vi "tvac_gui_chamber_backup.vi"() -> ()   [LabVIEW 2017]
uses:
  Zones.ctl
  <vilib>/Utility/miscctls.llb/LVPositionTypeDef.ctl
  <vilib>/httpClient/ClientHandle.ctl
  <vilib>/Utility/miscctls.llb/LVBoundsTypeDef.ctl
  <vilib>/Utility/error.llb/DialogType.ctl
  msg7171_linux.llb/send single message.vi
  <vilib>/httpClient/POSTBuffer.vi
  <vilib>/Utility/file.llb/Read Delimited Spreadsheet (string).vi
  <vilib>/Utility/file.llb/Write Delimited Spreadsheet (string).vi
  <vilib>/httpClient/LabVIEWHTTPClient.lvlib
panel:
  in  "TCs1to45InitialPositions":T1[](array[typedef])=[{"Left"=536, "Top"=477}, {"Left"=577, "Top"=477}, {"Left"=619, "Top"=477}, {"Left"=661, "Top"=477}, {"Left"=702, "Top"=477}, {"Left"=744, "Top"=477}, {"Left"=786, "Top"=477}, {"Left"=827, "Top"=477}, {"Left"=869, "Top"=477}, {"Left"=911, "Top"=477}, {"Left"=952, "Top"=477}, {"Left"=994, "Top"=477}, {"Left"=1036, "Top"=477}, {"Left"=1077, "Top"=477}, {"Left"=1119, "Top"=477}, {"Left"=536, "Top"=516}, {"Left"=577, "Top"=516}, {"Left"=619, "Top"=516}, {"Left"=661, "Top"=516}, {"Left"=702, "Top"=516}, {"Left"=744, "Top"=516}, {"Left"=786, "Top"=516}, {"Left"=827, "Top"=516}, {"Left"=869, "Top"=516}, {"Left"=911, "Top"=516}, {"Left"=952, "Top"=516}, {"Left"=994, "Top"=516}, {"Left"=1036, "Top"=516}, {"Left"=1077, "Top"=516}, {"Left"=1119, "Top"=516}, {"Left"=536, "Top"=555}, {"Left"=577, "Top"=555}, {"Left"=619, "Top"=555}, {"Left"=661, "Top"=555}, {"Left"=702, "Top"=555}, {"Left"=744, "Top"=555}, {"Left"=786, "Top"=555}, {"Left"=827, "Top"=555}, {"Left"=869, "Top"=555}, {"Left"=911, "Top"=555}, {"Left"=952, "Top"=555}, {"Left"=994, "Top"=555}, {"Left"=1036, "Top"=555}, {"Left"=1077, "Top"=555}, {"Left"=1119, "Top"=555}]
  in  "Moving 2":bool
  in  "Moving 1":bool
  in  "TC1to45PicRef":refnum<vi>
  in  "profilearray":dbl[][](array[numeric])
  in  "LastSetPt":i32
  in  "TVAC Labview":bool=TRUE
  in  "string":string
  in  "tprofilesheet":string[][](array[string])
  in  "Custom Graph Selector":i32
  in  "exit":bool
  in  "AlarmColor":u32(colorbox)
  in  "Alarm String":string
  in  "Plot Color":u32(colorbox)=16860
  in  "Temperature":dbl format="%#_13g"
  in  "TC Label":string
  in  "Graph ON/OFF":u32(colorbox)=4250624
  in  "index (col)":i32
  in  "index (row)":i32
  out "working array":bool[](array[boolean])
  in  "Local Debug":bool
  in  "Tab Control":T2(tab)
  in  "Log/Linear Y-Axis":u16(ring) items=["Linear", "Log"]
  in  "Total Time":dbl
  in  "Set Time TC Graph":bool
  in  "Graphing Selection":u16(ring) items=["User Selection", "Graph All Thermocouples", "Clear Graph"]
  in  "Time Scale":u16(ring) items=["Minutes", "Hours", "Seconds"]
  out "Waveform Chart":waveform(dbl)[](graph)
  out "Thermocouples":T3(array[cluster])
  in  "Log/Linear Y-Axis 6":u16(ring) items=["Linear", "Log"]
  in  "Log/Linear Y-Axis 5":u16(ring) items=["Linear", "Log"]
  in  "Log/Linear Y-Axis 3":u16(ring) items=["Linear", "Log"]
  in  "Log/Linear Y-Axis 2":u16(ring) items=["Linear", "Log"]
  in  "Total Time 6":dbl
  in  "Set Time TC Graph 6":bool
  in  "Time Scale 6":u16(ring) items=["Minutes", "Hours", "Seconds"]
  in  "Total Time 5":dbl
  in  "Set Time TC Graph 5":bool
  in  "Time Scale 5":u16(ring) items=["Minutes", "Hours", "Seconds"]
  in  "Total Time 4":dbl
  in  "Set Time TC Graph 4":bool
  in  "Time Scale 4":u16(ring) items=["Minutes", "Hours", "Seconds"]
  in  "Total Time 3":dbl
  in  "Set Time TC Graph 3":bool
  in  "Time Scale 3":u16(ring) items=["Minutes", "Hours", "Seconds"]
  in  "Total Time 2":dbl
  in  "Set Time TC Graph 2":bool
  in  "Time Scale 2":u16(ring) items=["Minutes", "Hours", "Seconds"]
  in  "Log/Linear Y-Axis 1":u16(ring) items=["Linear", "Log"]
  in  "Total Time 1":dbl
  in  "Set Time TC Graph 1":bool
  in  "Time Scale 1":u16(ring) items=["Minutes", "Hours", "Seconds"]
  in  "Custom Chart 2 Selection":i32[](listbox)=[0]
  in  "Custom Chart 1 Selection":i32[](listbox)=[0]
  out "Custom Chart 1":waveform(dbl)[](graph)
  in  "Custom Chart 3 Selection":i32[](listbox)=[0]
  in  "Custom Chart 4 Selection":i32[](listbox)=[0]
  in  "Custom Chart 5 Selection":i32[](listbox)=[0]
  in  "Custom Chart 6 Selection":i32[](listbox)=[0]
  out "Custom Chart 2":waveform(dbl)[](graph)
  out "Custom Chart 3":waveform(dbl)[](graph)
  out "Custom Chart 4":waveform(dbl)[](graph)
  out "Custom Chart 5":waveform(dbl)[](graph)
  out "Custom Chart 6":waveform(dbl)[](graph)
  in  "Log/Linear Y-Axis 4":u16(ring) items=["Linear", "Log"]
  out "ThermalProfileStatus":string
  in  "Import Profile":bool
  out "Thermal Profile":cluster{dbl, dbl, "temp":dbl[][]}(graph)
  in  "CreateTProfile":T4(tab)
  in  "ZoneSetup":T5={"Number of Set points"=0.0, "Zone Selection"=[8], "Initiate Setup"=FALSE, "Thermal Profile Name"=""}
  in  "RampSoakTimes":cluster{"RampSoakTimes":dbl[][]}
  in  "Zone 1":T6={"Zone Thermocouples"=[0], "Temperature Calculation"=0, "Thermocouples Selected"="", "Temperature Goal"=[], "Max Allowable Temp"="", "Min Allowable Temp"="", "Max Temp Slope"=""} {"Temperature Calculation" items=["Average", "Minimum", "Maximum"]}
  in  "Zone 2":T6={"Zone Thermocouples"=[0], "Temperature Calculation"=0, "Thermocouples Selected"="", "Temperature Goal"=[], "Max Allowable Temp"="", "Min Allowable Temp"="", "Max Temp Slope"=""} {"Temperature Calculation" items=["Average", "Minimum", "Maximum"]}
  in  "Zone 3":T6={"Zone Thermocouples"=[0], "Temperature Calculation"=0, "Thermocouples Selected"="", "Temperature Goal"=[], "Max Allowable Temp"="", "Min Allowable Temp"="", "Max Temp Slope"=""} {"Temperature Calculation" items=["Average", "Minimum", "Maximum"]}
  in  "Zone 4":T6={"Zone Thermocouples"=[0], "Temperature Calculation"=0, "Thermocouples Selected"="", "Temperature Goal"=[], "Max Allowable Temp"="", "Min Allowable Temp"="", "Max Temp Slope"=""} {"Temperature Calculation" items=["Average", "Minimum", "Maximum"]}
  in  "Zone 5":T6={"Zone Thermocouples"=[0], "Temperature Calculation"=0, "Thermocouples Selected"="", "Temperature Goal"=[], "Max Allowable Temp"="", "Min Allowable Temp"="", "Max Temp Slope"=""} {"Temperature Calculation" items=["Average", "Minimum", "Maximum"]}
  in  "Zone 6":T6={"Zone Thermocouples"=[0], "Temperature Calculation"=0, "Thermocouples Selected"="", "Temperature Goal"=[], "Max Allowable Temp"="", "Min Allowable Temp"="", "Max Temp Slope"=""} {"Temperature Calculation" items=["Average", "Minimum", "Maximum"]}
  in  "Zone 7":T6={"Zone Thermocouples"=[0], "Temperature Calculation"=0, "Thermocouples Selected"="", "Temperature Goal"=[], "Max Allowable Temp"="", "Min Allowable Temp"="", "Max Temp Slope"=""} {"Temperature Calculation" items=["Average", "Minimum", "Maximum"]}
  in  "Zone 8":T6={"Zone Thermocouples"=[0], "Temperature Calculation"=0, "Thermocouples Selected"="", "Temperature Goal"=[], "Max Allowable Temp"="", "Min Allowable Temp"="", "Max Temp Slope"=""} {"Temperature Calculation" items=["Average", "Minimum", "Maximum"]}
  in  "Zone 9":T6={"Zone Thermocouples"=[0], "Temperature Calculation"=0, "Thermocouples Selected"="", "Temperature Goal"=[], "Max Allowable Temp"="", "Min Allowable Temp"="", "Max Temp Slope"=""} {"Temperature Calculation" items=["Average", "Minimum", "Maximum"]}
  in  "New Name":string
  in  "Rename":bool
  in  "2. Save Into Database":bool
  in  "Save as CSV":bool
  in  "3. Load into Memory":bool
  in  "1. Compile Profile":bool
  in  "4. Run Profile":bool
  in  "Resume Profile":bool
  in  "Stop Profile":bool
  in  "Pause Profile":bool
  in  "Hold Profile":bool
  in  "Path":path
  in  "Tab Control 2":enum32{"TCs 1-45", "TCs 46-120"}(tab)
  out "TC1to45visual":T7={"1"=TRUE, "2"=TRUE, "3"=TRUE, "4"=TRUE, "5"=TRUE, "6"=TRUE, "7"=TRUE, "8"=TRUE, "9"=TRUE, "10"=TRUE, "11"=TRUE, "12"=TRUE, "13"=TRUE, "14"=TRUE, "15"=TRUE, "16"=TRUE, "17"=TRUE, "18"=TRUE, "19"=TRUE, "20"=TRUE, "21"=TRUE, "22"=TRUE, "23"=TRUE, "24"=TRUE, "25"=TRUE, "26"=TRUE, "27"=TRUE, "28"=TRUE, "29"=TRUE, "30"=TRUE, "31"=TRUE, "32"=TRUE, "33"=TRUE, "34"=TRUE, "35"=TRUE, "36"=TRUE, "37"=TRUE, "38"=TRUE, "39"=TRUE, "40"=TRUE, "41"=TRUE, "42"=TRUE, "43"=TRUE, "44"=TRUE, "45"=TRUE, "new picture"=bytes[0]}
  in  "Reset All TC Positions":bool
  in  "Events":enum32{"Current", "Past"}(tab)
  in  "Clear All Events":bool
  in  "Current Events (click to clear)":i32(listbox)
  in  "Export Events":bool
  in  "Event History":i32(listbox)
  in  "Errors":enum32{"Current Errors", "Cleared Errors"}(tab)
  in  "Current Errors (click to clear)":i32(listbox)
  in  "Clear All Errors":bool
  in  "Export Errors":bool
  in  "Error History":i32(listbox)
  in  "GetEvent":bool=TRUE
  in  "TCs On":bool=TRUE
  in  "Pressure On":bool=TRUE
  in  "MCC On":bool=TRUE
  in  "ZoneTemps On":bool=TRUE
  in  "Compressor On":bool
  in  "GetError":bool=TRUE
  out "flushed msgs":T8(array[cluster])
  out "system log event":string
  # "Hidden Controls"
  # "Set Pt #"
  # "Ramp Time (s)"
  # "Soak Time (s)"
  # "Set Pt #"
  # "Goal Temp (K)"
  # "Set Pt #"
  # "Goal Temp (K)"
  # "Set Pt #"
  # "Goal Temp (K)"
  # "Set Pt #"
  # "Goal Temp (K)"
  # "Set Pt #"
  # "Goal Temp (K)"
  # "Set Pt #"
  # "Goal Temp (K)"
  # "Set Pt #"
  # "Goal Temp (K)"
  # "Set Pt #"
  # "Goal Temp (K)"
  # "Set Pt #"
  # "Goal Temp (K)"
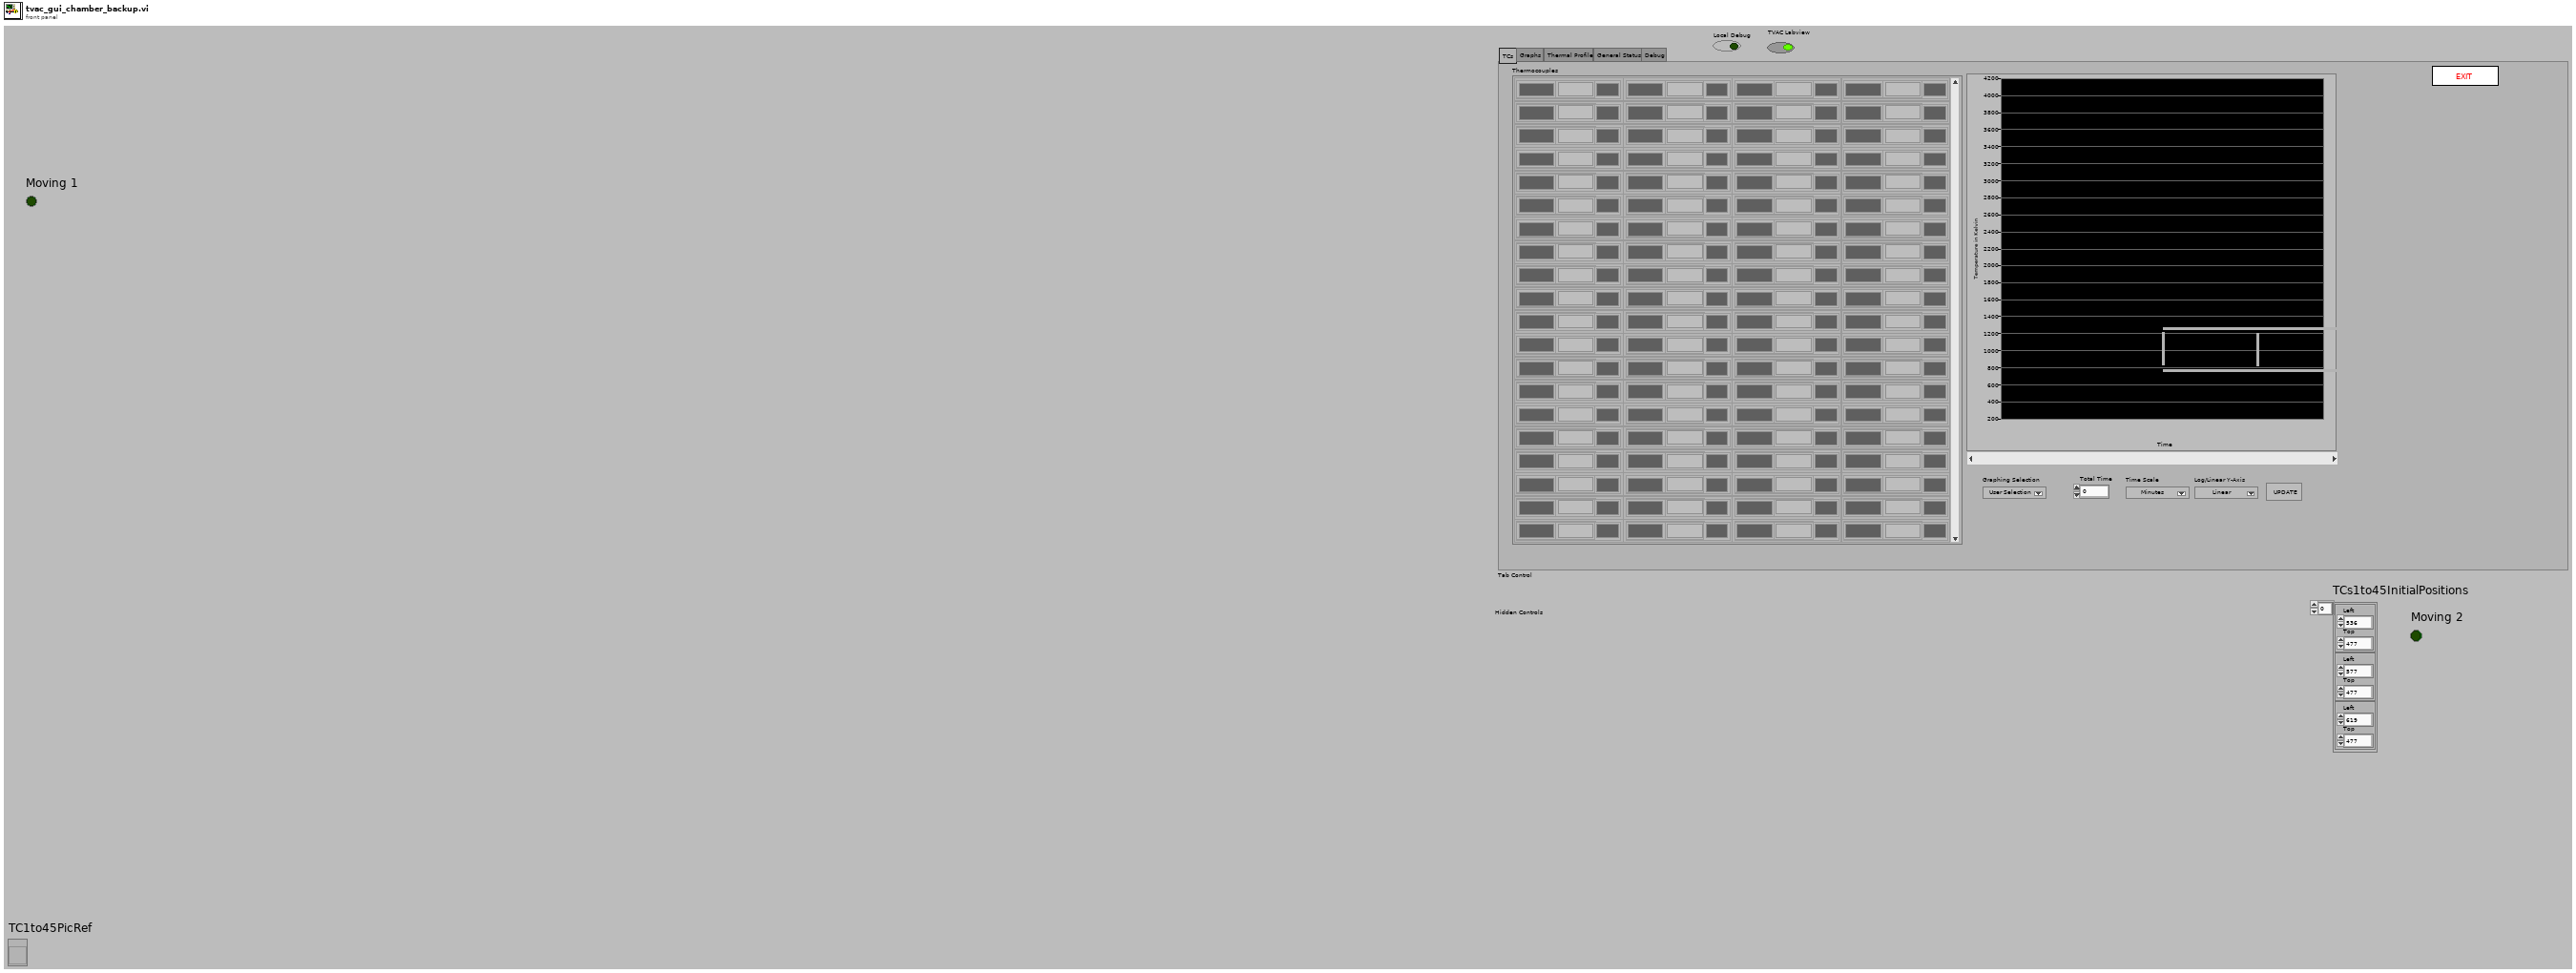
[diagram p1: front panel]
types:
  T1 = typedef "LVPositionTypeDef.ctl" = cluster{"Left":i32, "Top":i32}
  T2 = enum32{"TCs", "Graphs", "Thermal Profile", "General Status", "Debug"}
  T3 = cluster{"TC Label":string, "Alarm Status":string, "Alarm Color":u32, "Temperature":string, "PlotColor":u32, "Graph On/Off":u32}[][]
  T4 = enum32{"Setup", "Setup 2", "Zone 1", "Zone 2", "Zone 3", "Zone 4", "Zone 5", "Zone 6", "Zone 7", "Zone 8", "Zone 9", "Preview Profile"}
  T5 = cluster{"Number of Set points":dbl, "Zone Selection":i32[], "Initiate Setup":bool, "Thermal Profile Name":string}
  T6 = typedef "Zones.ctl" = cluster{"Zone Thermocouples":i32[], "Temperature Calculation":u16, "Thermocouples Selected":string, "Temperature Goal":dbl[][], "Max Allowable Temp":string, "Min Allowable Temp":string, "Max Temp Slope":string}
  T7 = cluster{"1":bool, "2":bool, "3":bool, "4":bool, "5":bool, "6":bool, "7":bool, "8":bool, "9":bool, "10":bool, "11":bool, "12":bool, "13":bool, "14":bool, "15":bool, "16":bool, "17":bool, "18":bool, "19":bool, "20":bool, "21":bool, "22":bool, "23":bool, "24":bool, "25":bool, "26":bool, "27":bool, "28":bool, "29":bool, "30":bool, "31":bool, "32":bool, "33":bool, "34":bool, "35":bool, "36":bool, "37":bool, "38":bool, "39":bool, "40":bool, "41":bool, "42":bool, "43":bool, "44":bool, "45":bool, "new picture":picture}
  T8 = cluster{"source":string, "event":string, "event buffer":string}[]
  T9 = cluster{"profiles":cluster{"zone":i32, "average":string, "thermocouples":i32[], "maxTemp":i32, "minTemp":i32, "maxSlope":i32, "thermalprofiles":cluster{"thermalsetpoint":i32, "tempgoal":i32, "ramp":i32, "soakduration":i32}[]}[]}
  T10 = cluster{"thermocouple":i32, "time":dbl, "temp":dbl, "working":bool, "alarm":i32}[]
  T11 = cluster{"Cp Stage 1 Temp":dbl[], "Cp Stage 2 Temp":dbl[]}
  T12 = typedef "LabVIEWHTTPClient.lvlib/ClientHandle.ctl" = refnum<k1>
  T13 = cluster{"ZoneSetup":cluster{"Number of Set points":dbl, "Zone Selection":i32[], "Initiate Setup":bool, "Thermal Profile Name":string}, "go":bool, "Http session":T12, "URL prefex":string, "index (row)":i32, "index (col)":i32, "Graph ON/OFF":u32, "TC Label":string, "Temperature":dbl, "AlarmColor":u32, "Plot Color":u32, "Alarm String":string, "Thermocouples":cluster{"TC Label":string, "Alarm Status":string, "Alarm Color":u32, "Temperature":string, "PlotColor":u32, "Graph On/Off":u32}[][], "working array":bool[], "i":i32, "NumberTCs":i32, "Waveform Chart":waveform(dbl)[], "Custom Chart 1":waveform(dbl)[], "Pressure":dbl[], "numSensors":i32, "Database":dbl[], "PumpTemps":cluster{"Cp Stage 1 Temp":dbl[], "Cp Stage 2 Temp":dbl[]}, "Zones":dbl[], "Time":i32, "TCs":cluster{"thermocouple":i32, "time":dbl, "temp":dbl, "working":bool, "alarm":i32}[], "ZoneTemps":cluster{"ZoneTemps":dbl[]}, "Compressor":cluster{"CompressorTemp":dbl}, "ErrorArray":string[][], "PrevErrorArray":string[][], "MasterErrorArray":string[][], "tprofilesheet":string[][], "Zone 1":T6, "ZoneProfile":cluster{"profiles":cluster{"zone":i32, "average":string, "thermocouples":i32[], "maxTemp":i32, "minTemp":i32, "maxSlope":i32, "thermalprofiles":cluster{"thermalsetpoint":i32, "tempgoal":i32, "ramp":i32, "soakduration":i32}[]}[]}, "ZonesSelected":bool[], "Zone 2":T6, "Zone 3":T6, "Zone 4":T6, "Zone 5":T6, "Zone 6":T6, "Zone 7":T6, "Zone 8":T6, "Zone 9":T6, "MasterEventArray":string[][], "PrevEventArray":string[][], "EventArray":string[][], "Moving 1":bool, "Moving 2":bool, "TCs1to45InitialPositions":T1[]}
  T14 = cluster{"TC Label":string, "Alarm Status":string, "Alarm Color":u32, "Temperature":string, "PlotColor":u32, "Graph On/Off":u32}
  T15 = cluster{"name":string, "profiles":cluster{"zone":i32, "average":string, "thermocouples":i32[], "maxTemp":i32, "minTemp":i32, "maxSlope":i32, "thermalprofiles":cluster{"thermalsetpoint":i32, "tempgoal":i32, "ramp":i32, "soakduration":i32}[]}[]}
  T16 = typedef "LVBoundsTypeDef.ctl" = cluster{"Width":u32, "Height":u32}
  T17 = enum16{"open", "replace", "create", "open or create", "replace or create", "replace or create with confirmation"}
  T18 = cluster{"zone":i32, "average":string, "thermocouples":i32[], "maxTemp":i32, "minTemp":i32, "maxSlope":i32, "thermalprofiles":cluster{"thermalsetpoint":i32, "tempgoal":i32, "ramp":i32, "soakduration":i32}[]}
  T19 = cluster{"thermalsetpoint":i32, "tempgoal":i32, "ramp":i32, "soakduration":i32}
  T20 = cluster{"DutyCycle":i32, "Stage1Temp":i32, "CryoPumpReadyState":cluster{"MotorOn":bool, "Ready":bool}, "PurgeValveState":bool, "RegenError":string, "RegenStep":string, "RoughingValveState":bool, "RoughingInterlock":cluster{"RoughingPermission":bool, "RoughingNeeded":bool, "Cryopumprunning":bool}, "Stage2Temp":i32, "Status":cluster{"PumpOn":bool, "RoughOpen":bool, "PurgeOpen":bool, "ThermocoupleGaugeOn":bool, "PowerFailureOccurred":bool}, "TcPressure":i32}
  T21 = cluster{"time":string[], "event":string[], "item":string[], "details":string[], "actions":string[]}
  T22 = enum32{"TCs", "Graphs", "Thermal Profile", "General Status"}
  T23 = cluster{"time":string[], "category":string[], "message":string[]}
  T24 = cluster{"CryoPressure":dbl, "ChamberPressure":dbl, "RoughingPressure":dbl}
  T25 = cluster{"time":string, "TCs":cluster{"thermocouple":i32, "time":dbl, "temp":dbl, "working":bool, "alarm":i32}[]}
  T26 = typedef "LVPoint32TypeDef.ctl" = cluster{"Horizontal":i32, "Vertical":i32}
  T27 = typedef "LVRangeTypeDef.ctl" = cluster{"Minimum":dbl, "Maximum":dbl, "Increment":dbl, "Minor Increment":dbl, "Start":dbl}
  T28 = cluster{"zone":i32, "average":string, "thermocouples":i32[], "maxTemp":i32, "minTemp":i32, "maxSlope":i32, "thermalprofiles":cluster{"thermalsetpoint":i32, "tempgoal":i32, "ramp":i32, "soakduration":i32}[]}[]
  T29 = typedef "LVRowAndColumnTypeDef.ctl" = cluster{"Row":i32, "Column":i32}
  T30 = cluster{"thermalsetpoint":i32, "tempgoal":i32, "ramp":i32, "soakduration":i32}[]
  T31 = cluster{"time":dbl[], "zone1":dbl[], "zone2":dbl[], "zone3":dbl[], "zone4":dbl[], "zone5":dbl[], "zone6":dbl[], "zone7":dbl[], "zone8":dbl[], "zone9":dbl[]}
  T32 = typedef "DialogType.ctl" = u16
  T33 = typedef "imagedata.ctl" = cluster{"image type":i32, "image depth":i32, "image":u8[], "mask":u8[], "colors":u32[], "Rectangle":cluster{"left":i16, "top":i16, "right":i16, "bottom":i16}}
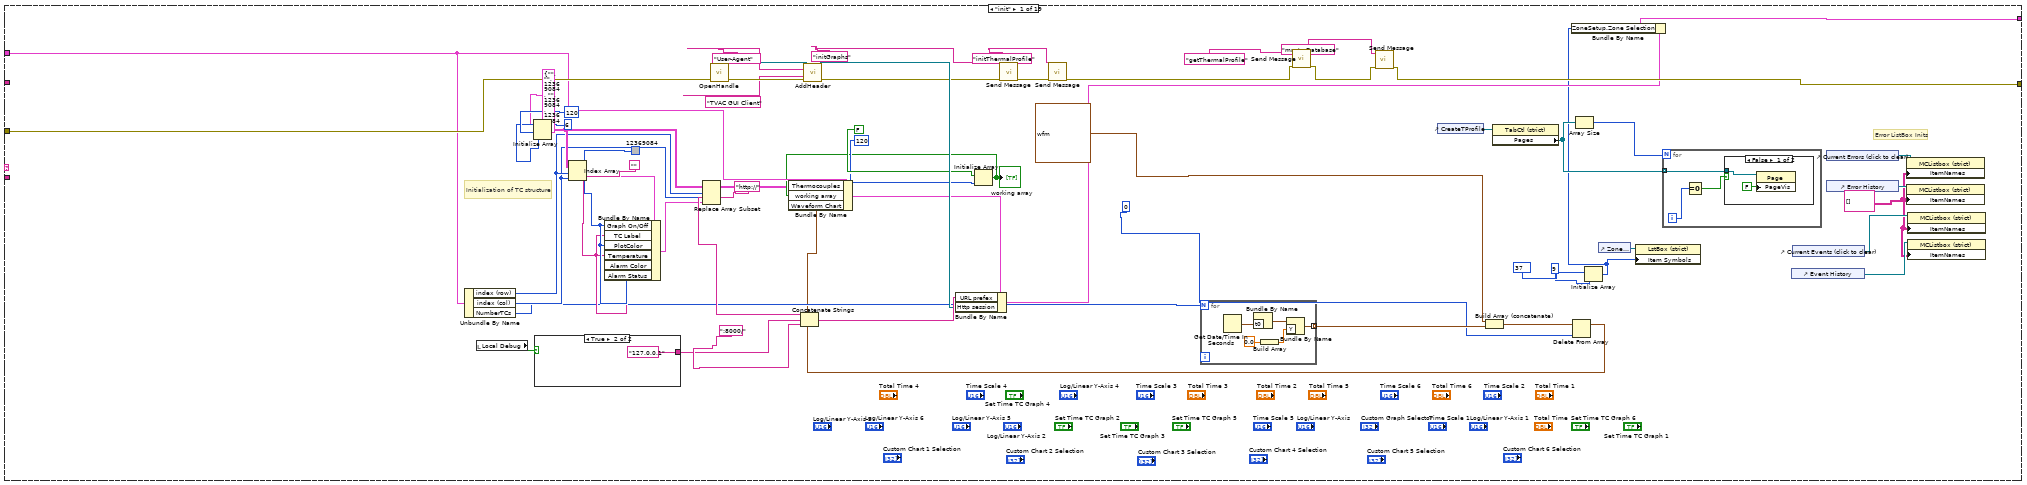
[diagram p2: hidden frame]
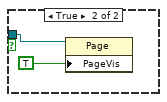
[diagram p3: hidden frame]
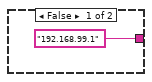
[diagram p4: hidden frame]
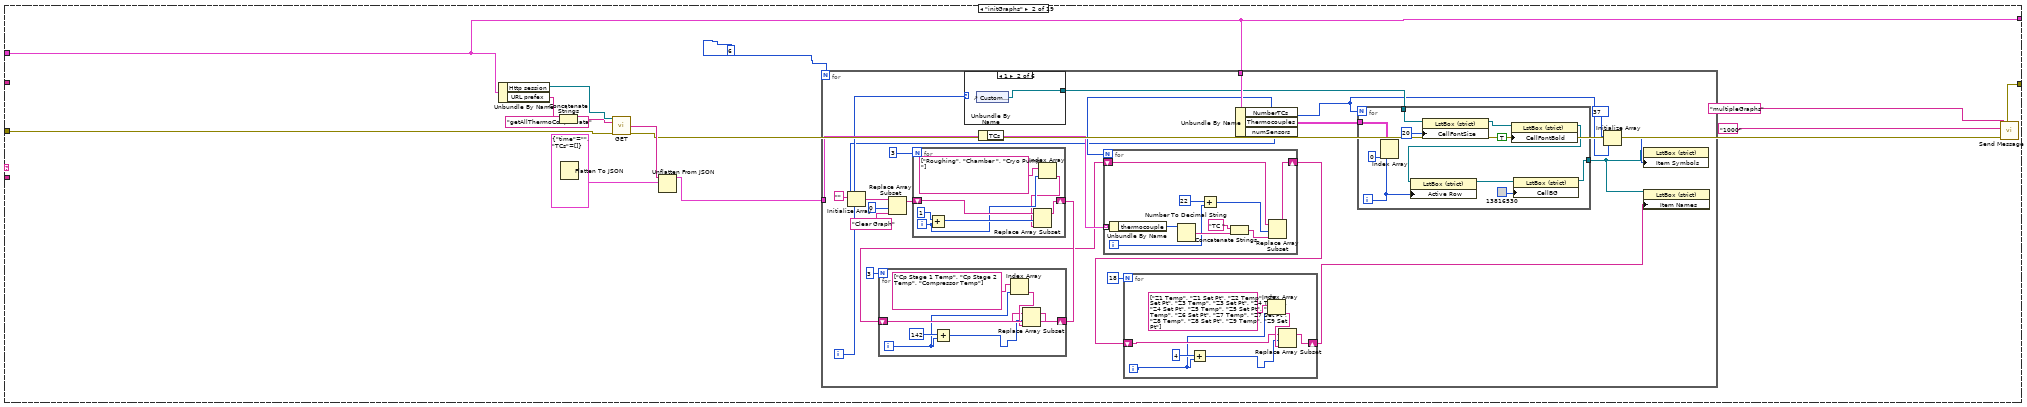
[diagram p5: hidden frame]
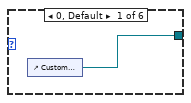
[diagram p6: hidden frame]
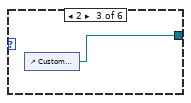
[diagram p7: hidden frame]
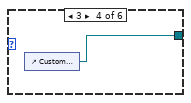
[diagram p8: hidden frame]
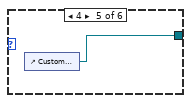
[diagram p9: hidden frame]
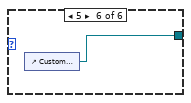
[diagram p10: hidden frame]
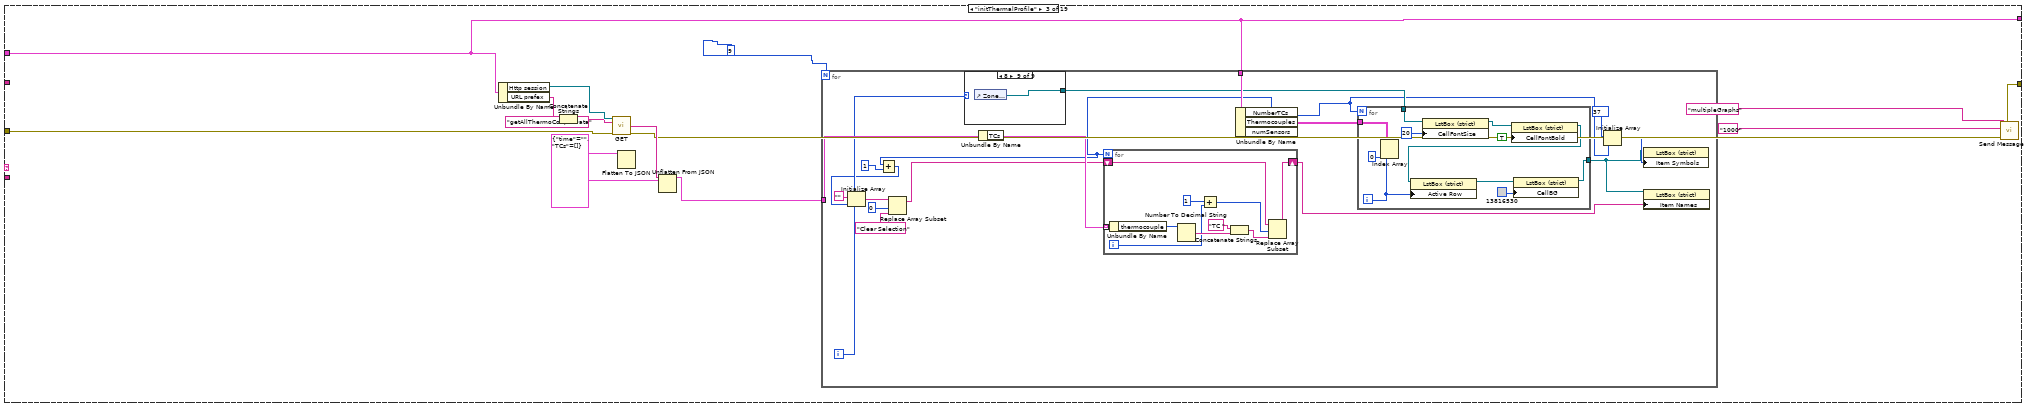
[diagram p11: hidden frame]
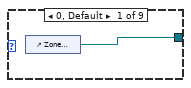
[diagram p12: hidden frame]
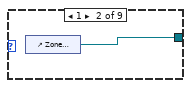
[diagram p13: hidden frame]
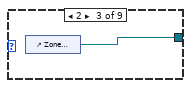
[diagram p14: hidden frame]
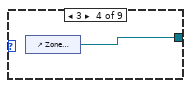
[diagram p15: hidden frame]
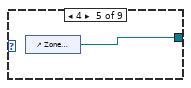
[diagram p16: hidden frame]
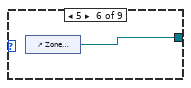
[diagram p17: hidden frame]
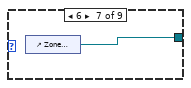
[diagram p18: hidden frame]
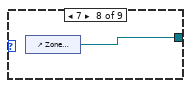
[diagram p19: hidden frame]
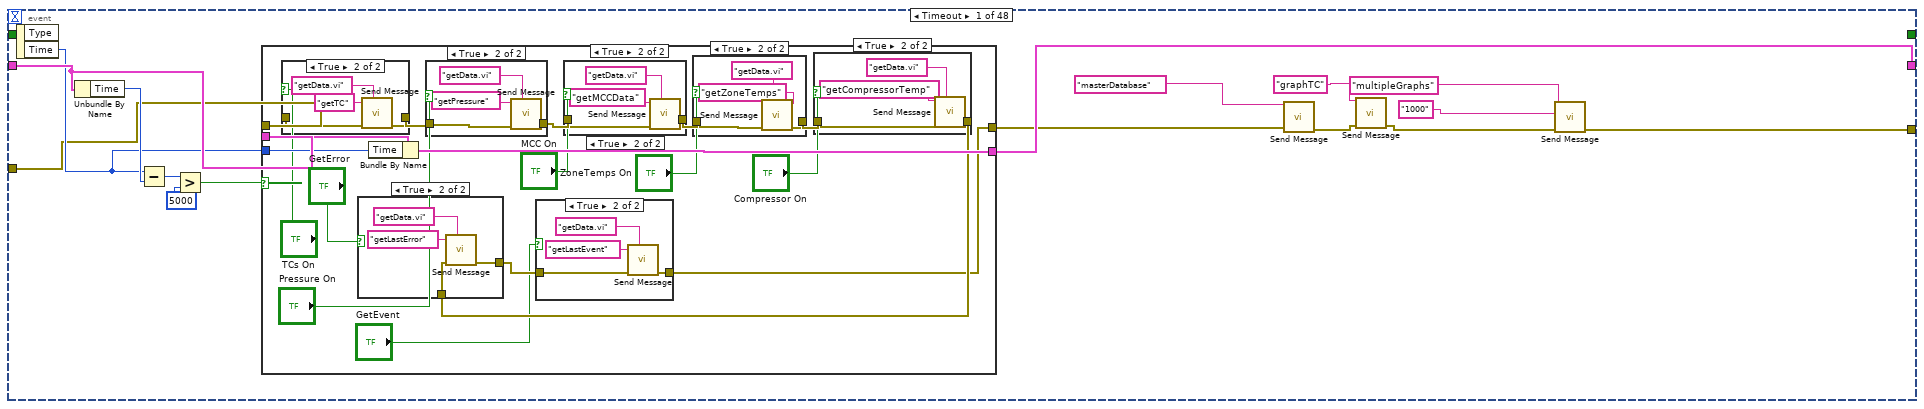
[diagram p20: hidden frame]
diagram:
  w17 = string[][] []  # MasterEventArray
  w15 = string[][] []  # EventArray
  w16 = string[][] []  # PrevEventArray
  w18 = string[][] []  # MasterErrorArray
  w22 = T9 {"profiles"=[]}  # ZoneProfile
  w31 = bool[] [FALSE, FALSE, FALSE, FALSE, FALSE, FALSE, FALSE, FALSE, FALSE]  # ZonesSelected
  w35 = string[][] []  # PrevErrorArray
  w36 = string[][] []  # ErrorArray
  w39 = cluster{"ZoneTemps":dbl[]} {"ZoneTemps"=[]}  # ZoneTemps
  w42 = dbl[] [24.54828257301887, 25.0, 20.035959453954195, 26.0, 28.926820041278148, 27.0, 21.321976066931608, 28.0, 29.197600688359813, 29.0, 29.117373424110085, 30.0, 21.092914485312942, 31.0, 27.791581465649088, 32.0, 24.70861457288988, 33.0]  # Zones
  w43 = T11 {"Cp Stage 1 Temp"=[0.0], "Cp Stage 2 Temp"=[0.0]}  # PumpTemps
  w44 = dbl[] [0.0, 1000.5841582194602, 1000.5841582194602, 1000.5841582194602, 0.6389895835935778, 0.7578061575842531, 1.153531014677555, 1.4572061556343079, 1.0192558642672256, 0.9245021790184325, 0.34311035179988925, 1.1970333160202968, 1.066989851322369, 0.5926593131154867, 0.7219240511326698, 1.0529790116491695, 1.4485694746891444, 0.9139060201605569, 0.7997359753068659, 0.6568795179977746, 0.8470104541419833, 1.0272585161866683, 0.6577301535824354, 0.645139941938139, 1.5235316442408067, 0.5128651184775285, 1.6421980587090137, 1.3961508335147417, 1.1242639015795428, 1.5954313466624428, 1.1919135255187876, 1.2615004458206727, 1.1320092264321664, 1.922759836270222, 1.1315561200367314, 1.4924621723754858, 0.6988771274186227, 1.069709701591943, 0.9920698240997152, 0.5395549253287656, 0.42891479657680576, 1.2794224940227927, 0.2687949632437338, 0.16127136772755854, 1.0174597006256374, 1.2079238230365172, 0.9745554383837218, 1.5348516925460962, 0.9488878852839246, 1.6634477658652282, 1.1924291951744272, 1.2231949298067308, 1.2223766746774598, 1.30664154589907, 1.2872878364107239, 0.5274250065177812, 0.7905999067114673, 1.2748974665085449, 1.216972941585413, 0.959115576325391, 0.5743502840762814, 0.8219540421676025, 0.613053899308251, 1.3785560870413707, 1.034117232127813, 1.1237698659753859, 1.4495548642149667, 0.6967905980938514, 0.6224497255665377, 1.6551326273040576, 1.2103048396824558, 0.6078721016951973, 1.3790669246280296, 0.5454332940871525, 1.5318777012492035, 1.2496539590411258, 0.9145395304446965, 1.3855381787793546, 1.0857600342029163, 1.3185833631438346, 0.9769688683142593, 1.026663691242448, 0.6744610422623843, 1.1965175398567691, 0.4847084945450119, 0.6435799980029115, 0.8079659363810663, 0.9130053929540112, 0.5271098423006861, 0.8088111736464799, 1.1455315536576556, 1.139809531926708, 1.5840192673434794, 1.0296748968089129, 1.7370669751200136, 1.3715484550405317, 0.3362063953932494, 1.0385868418202253, 1.4947740276021626, 1.0393600693910505, 0.8870410800672984, 1.2470388696569872, 0.9846724980375481, 0.9952471377109308, 1.0807485178906029, 1.1016630607035562, 1.3301039036808464, 0.8856852816151205, 0.4719509873120426, 0.5191430277856135, 0.12135113366044793, 0.4230478635224125, 1.1140562049976255, 1.5484968368781251, 1.1999891199114734, 1.8721302183420216, 1.071489235222563, 0.6260864330445979, 1.0305668002030492, 1.0223711899566386, 0.7842533472819472, 1.7301290335750898, 1.318694748426881, 0.6978662965493679]  # Database
  w46 = dbl[] [0.0, 0.0, 0.0]  # Pressure
  w65 = ""  # URL prefex
  w66 = T12 refnum  # Http session
  w67 = TRUE  # go
  n1 = call "Register Module.vi"() -> ("error out"=w63:errorcluster)  [unwired: 10 in, 1 out]
  n2 = call-poly "Send Message.vi"("error in (no error)"=w63, "event"="init") -> ("error out"=w62:errorcluster)  [unwired: 9 in]
  n3 = local read "Waveform Chart"() -> (w49:waveform(dbl)[])
  n4 = local read "Thermocouples"() -> (w48:T3)
  n5 = local read "Custom Chart 1"() -> (w47:waveform(dbl)[])
  n6 = Bundle("ZoneSetup"="ZoneSetup", "go"=w67, "Http session"=w66, "URL prefex"=w65, "index (row)"="index (row)", "index (col)"="index (col)", "Graph ON/OFF"="Graph ON/OFF", "TC Label"="TC Label", "Temperature"="Temperature", "AlarmColor"="AlarmColor", "Plot Color"="Plot Color", "Alarm String"="Alarm String", "Thermocouples"=w48, "working array"=bool[] [TRUE, TRUE, TRUE, TRUE, TRUE, TRUE, TRUE, TRUE, TRUE, TRUE, TRUE, TRUE, TRUE, TRUE, TRUE, TRUE, TRUE, TRUE, TRUE, TRUE, TRUE, TRUE, TRUE, TRUE, TRUE, TRUE, TRUE, TRUE, TRUE, TRUE, TRUE, TRUE, TRUE, TRUE, TRUE, TRUE, TRUE, TRUE, TRUE, TRUE, TRUE, TRUE, TRUE, TRUE, TRUE, TRUE, TRUE, TRUE, TRUE, TRUE, TRUE, TRUE, TRUE, TRUE, TRUE, TRUE, TRUE, TRUE, TRUE, TRUE, TRUE, TRUE, TRUE, TRUE, TRUE, TRUE, TRUE, TRUE, TRUE, TRUE, TRUE, TRUE, TRUE, TRUE, TRUE, TRUE, TRUE, TRUE, TRUE, TRUE, TRUE, TRUE, TRUE, TRUE, TRUE, TRUE, TRUE, TRUE, TRUE, TRUE, TRUE, TRUE, TRUE, TRUE, TRUE, TRUE, TRUE, TRUE, TRUE, TRUE, TRUE, TRUE, TRUE, TRUE, TRUE, TRUE, TRUE, TRUE, TRUE, TRUE, TRUE, TRUE, TRUE, TRUE, TRUE, TRUE, TRUE, TRUE, TRUE, TRUE], "i"=0, "NumberTCs"=120, "Waveform Chart"=w49, "Custom Chart 1"=w47, "Pressure"=w46, "numSensors"=145, "Database"=w44, "PumpTemps"=w43, "Zones"=w42, "Time"=0, "TCs"=T10 [], "ZoneTemps"=w39, "Compressor"=cluster{"CompressorTemp":dbl} {"CompressorTemp"=0.0}, "ErrorArray"=w36, "PrevErrorArray"=w35, "MasterErrorArray"=w18, "tprofilesheet"="tprofilesheet", "Zone 1"="Zone 1", "ZoneProfile"=w22, "ZonesSelected"=w31, "Zone 2"="Zone 2", "Zone 3"="Zone 3", "Zone 4"="Zone 4", "Zone 5"="Zone 5", "Zone 6"="Zone 6", "Zone 7"="Zone 7", "Zone 8"="Zone 8", "Zone 9"="Zone 9", "MasterEventArray"=w17, "PrevEventArray"=w16, "EventArray"=w15, "Moving 1"="Moving 1", "Moving 2"="Moving 2", "TCs1to45InitialPositions"="TCs1to45InitialPositions") -> (w53:T13)  [unwired: 1 in]
  n7 = while {
    shift-left: w53 -> [w73]
    shift-right: [w70] -> _
    shift-right: [w71] -> w21
    shift-left: w62 -> [w78]
    stop <- w69 continue-if-true
    n8 = call "Get Message.vi"("error in (no error)"=w78) -> ("error out"=w76:errorcluster, "event buffer"=w77:string, "event"=w75:string, "source"=w74:string)  [unwired: 7 in]
    n9 = case shown="\"\", \"Idle\"" w75 {
      selector: w75 -> [_ _ _ _ _ _ _ _ _ _ _ _ _ _ _ _ _ _ w3393]
      tunnel: [w84 w155 w240 w298 w2121 w2332 w2852 w2948 w3031 w3045 w3064 w3133 w3189 w3194 w3212 w3225 w3245 w3391 w3395] -> w70
      tunnel: w73 -> [w109 w155 w240 w301 w2122 w2346 w2853 w2953 w3030 w3044 w3058 w3127 w3190 w3200 w3211 w3226 w3245 w3387 w3395]
      tunnel: w77 -> [_ _ _ _ _ _ _ _ w3028 w3034 w3065 w3134 w3181 w3199 w3209 _ w3246 _ _]
      tunnel: w76 -> [w130 w154 w239 w303 w2113 w2331 w2855 w2943 w3029 w3035 w3062 w3131 w3182 w3198 w3210 w3231 _ w3390 w3394]
      tunnel: [w94 w150 w235 w302 w2097 w2339 w2855 w2943 w3029 w3035 w3062 w3131 w3182 w3198 w3210 w3231 _ w3389 w3392] -> w72
      tunnel: w74 -> [_ _ _ _ _ _ _ _ _ _ _ _ _ _ _ _ _ _ _]
      frame "init" {
        w79 = string[][] [] ("Item Names")
        w114 = ""
        w115 = u32 12369084 ("PlotColor")
        # "Error ListBox Inits"
        # "Initialization of TC structure"
        n10 = Unbundle By Name(w109) -> ("index (row)"=w117:i32, "index (col)"=w116:i32, "NumberTCs"=w106:i32)
        n11 = local read "Local Debug"() -> (w122:bool)
        n12 = Initialize Array(T14 {"TC Label"="", "Alarm Status"="", "Alarm Color"=12369084, "Temperature"="", "PlotColor"=12369084, "Graph On/Off"=12369084}, 120 ("dimension size"), 6 ("dimension size")) -> (w118:T3)
        n13 = case shown="True" w122 {
          tunnel: ["192.168.99.1" ("Address") "127.0.0.1" ("Address")] -> w123
          frame False {
          }
          frame True {
          }
        }
        n14 = Index Array(array=w118, index (row)=w117, index (col)=w116) -> (element=w113:T14)
        n15 = Bundle By Name(cluster=w113, "Graph On/Off"=w115, "TC Label"=w114, "PlotColor"=w115, "Temperature"=w114, "Alarm Color"=w115, "Alarm Status"=w114) -> (w112:T14)
        n16 = Replace Array Subset(array=w118, new element=w112, index (row)=w117, index (col)=w116) -> (w100:T3)
        n17 = call <vilib>:"OpenHandle.vi"("error in (no error)"=w130) -> ("client handle out"=w131:T12, "error out"=w134:errorcluster)  [unwired: 13 in]
        n18 = Concatenate Strings("http://" ("url"), w123, ":8000/" ("url")) -> (w127:string)
        n19 = call <vilib>:"AddHeader.vi"("client handle"=w131, "header"="User-Agent", "value"="TVAC GUI Client", "error in (no error)"=w134) -> ("client handle out"=w126:T12, "error out"=w125:errorcluster)  [unwired: 10 in]
        n20 = Initialize Array(FALSE ("Boolean"), 120 ("dimension size")) -> (w107:bool[])
        "working array" <- w107
        n21 = call-poly "Send Message.vi"("error in (no error)"=w125, "event"="initGraphs") -> ("error out"=w99:errorcluster)  [unwired: 9 in]
        n22 = call-poly "Send Message.vi"("error in (no error)"=w99, "event"="initThermalProfile") -> ("error out"=w97:errorcluster)  [unwired: 9 in]
        n23 = for {
          N: w106 -> [_]
          tunnel: [w142] -> w104 mode=indexing
          n24 = Get Date/Time In Seconds() -> (seconds since 1Jan1904=w146:timestamp)
          n25 = Bundle By Name("t0"=w146) -> (w143:waveform(dbl))  [unwired: 1 in]
          n26 = Build Array(0.0) -> (w145:dbl[])
          n27 = Bundle By Name(cluster=w143, "Y"=w145) -> (w142:waveform(dbl))
        }
        n28 = call-poly "Send Message.vi"("error in (no error)"=w97, "event"="getThermalProfile") -> ("error out"=w95:errorcluster)  [unwired: 9 in]
        n29 = call-poly "Send Message.vi"("error in (no error)"=w95, "event"="masterDatabase") -> ("error out"=w94:errorcluster)  [unwired: 9 in]
        n30 = control-ref of="CreateTProfile"() -> (w92:refnum<vi>)
        n31 = Build Array (concatenate)(waveform(dbl) {"t0"=timestamp(0 s since 1904-01-01), "dt"=1.0, "Y"=[0.0]} ("element"), w104) -> (w105:waveform(dbl)[])
        n32 = property on="Property Node" class="TabCtl (strict)"(reference=w92) -> ("Pages"=w90:refnum<vi>[])  [unwired: 1 in, 2 out]
        n33 = Delete From Array(array=w105, index=0) -> (array with subset deleted=w103:waveform(dbl)[])  [unwired: 1 in, 1 out]
        n34 = Bundle By Name(cluster=w109, "Thermocouples"=w100, "working array"=w107, "Waveform Chart"=w103) -> (w108:T13)
        n35 = Bundle By Name(cluster=w108, "URL prefex"=w127, "Http session"=w126) -> (w87:T13)
        n36 = Array Size(array=w90) -> (size(s)=w91:i32)
        n37 = Initialize Array(37, 9 ("dimension size")) -> (w85:i32[])
        n38 = Bundle By Name(cluster=w87, "ZoneSetup.Zone Selection"=w85) -> (w84:T13)
        n39 = control-ref of="Zone Selection"() -> (w86:refnum<vi>)
        n40 = property class="LstBox (strict)"(reference=w86, "Item Symbols"=w85) -> ()  [unwired: 1 in, 2 out]
        n41 = for {
          N: w91 -> [_]
          tunnel: w90 -> [w135] mode=indexing
          i -> [w137]
          n42 = Equal To 0?(x=w137) -> (x = 0?=w136:bool)
          n43 = case shown="False" w136 {
            tunnel: w135 -> [w138 w140]
            frame False {
              n44 = property on="Property Node" class="Page"(reference=w138, "PageVis"=FALSE ("Page Visible")) -> ()  [unwired: 1 in, 2 out]
            }
            frame True {
              n45 = property on="Property Node" class="Page"(reference=w140, "PageVis"=TRUE ("Page Selector Visible")) -> ()  [unwired: 1 in, 2 out]
            }
          }
        }
        n46 = control-ref of="Event History"() -> (w80:refnum<vi>)
        n47 = control-ref of="Current Events (click to clear)"() -> (w81:refnum<vi>)
        n48 = control-ref of="Current Errors (click to clear)"() -> (w83:refnum<vi>)
        n49 = control-ref of="Error History"() -> (w82:refnum<vi>)
        n50 = property on="Property Node" class="MCListbox (strict)"(reference=w83, "ItemNames"=w79) -> ()  [unwired: 1 in, 2 out]
        n51 = property on="Property Node" class="MCListbox (strict)"(reference=w82, "ItemNames"=w79) -> ()  [unwired: 1 in, 2 out]
        n52 = property on="Property Node" class="MCListbox (strict)"(reference=w81, "ItemNames"=w79) -> ()  [unwired: 1 in, 2 out]
        n53 = property on="Property Node" class="MCListbox (strict)"(reference=w80, "ItemNames"=w79) -> ()  [unwired: 1 in, 2 out]
      }
      frame "initGraphs" {
        w156 = T25 {"time"="", "TCs"=[]} ("Cluster")
        n54 = Unbundle By Name(w155) -> ("Http session"=w162:T12, "URL prefex"=w160:string)
        n55 = Concatenate Strings(w160, "getAllThermoCoupleData" ("url")) -> (w161:string)
        n56 = Flatten To JSON(anything=w156) -> ()  [unwired: 2 in, 2 out]
        n57 = call <vilib>:"GET.vi"("client handle"=w162, "url"=w161, "error in (no error)"=w154) -> ("body"=w158:string, "error out"=w151:errorcluster)  [unwired: 9 in, 2 out]
        n58 = Unflatten From JSON(JSON string=w158, type and defaults=w156) -> (value=w157:T25)  [unwired: 5 in, 1 out]
        n59 = for {
          N: 6 ("Numeric") -> [_]
          tunnel: w157 -> [w184]
          tunnel: w155 -> [w183]
          i -> [w166]
          n60 = case shown="1" w166 {
            tunnel: [w186 w187 w188 w189 w190 w191] -> w167
            frame 0, Default {
              n61 = control-ref of="Custom Chart 1 Selection"() -> (w186:refnum<vi>)
            }
            frame 1 {
              n62 = control-ref of="Custom Chart 2 Selection"() -> (w187:refnum<vi>)
            }
            frame 2 {
              n63 = control-ref of="Custom Chart 3 Selection"() -> (w188:refnum<vi>)
            }
            frame 3 {
              n64 = control-ref of="Custom Chart 4 Selection"() -> (w189:refnum<vi>)
            }
            frame 4 {
              n65 = control-ref of="Custom Chart 5 Selection"() -> (w190:refnum<vi>)
            }
            frame 5 {
              n66 = control-ref of="Custom Chart 6 Selection"() -> (w191:refnum<vi>)
            }
          }
          n67 = Unbundle By Name(w184) -> ("TCs"=w180:T10)
          n68 = Unbundle By Name(w183) -> ("NumberTCs"=w178:i32, "Thermocouples"=w185:T3, "numSensors"=w164:i32)
          n69 = Initialize Array("", w164) -> (w176:string[])
          n70 = Replace Array Subset(array=w176, new element="Clear Graph" ("new element/subarray"), index=0) -> (w173:string[])
          n71 = for {
            N: 3 -> [_]
            shift-right: [w211] -> w171
            shift-left: w173 -> [w212]
            i -> [w207]
            n72 = Add(x=1 ("index"), y=w207) -> (x+y=w209:i32)
            n73 = Index Array(array=string[] ["Roughing", "Chamber ", "Cryo Pump "], index=w207) -> (element=w206:string)
            n74 = Replace Array Subset(array=w212, new element=w206, index=w209) -> (w211:string[])
          }
          n75 = for {
            N: 3 -> [_]
            shift-right: [w202] -> w170
            shift-left: w171 -> [w203]
            i -> [w199]
            n76 = Add(x=142 ("index"), y=w199) -> (x+y=w200:i32)
            n77 = Index Array(array=string[] ["Cp Stage 1 Temp", "Cp Stage 2 Temp", "Compressor Temp"], index=w199) -> (element=w204:string)
            n78 = Replace Array Subset(array=w203, new element=w204, index=w200) -> (w202:string[])
          }
          n79 = for {
            N: w178 -> [_]
            tunnel: w180 -> [w219] mode=indexing
            shift-right: [w213] -> w163
            shift-left: w170 -> [w215]
            i -> [w217]
            n80 = Unbundle By Name(w219) -> ("thermocouple"=w220:i32)
            n81 = Number To Decimal String(number=w220) -> (decimal integer string=w222:string)  [unwired: 1 in]
            n82 = Add(x=22 ("index"), y=w217) -> (x+y=w216:i32)
            n83 = Concatenate Strings("TC " ("string"), w222) -> (w214:string)
            n84 = Replace Array Subset(array=w215, new element=w214, index=w216) -> (w213:string[])
          }
          n85 = for {
            N: 18 -> [_]
            shift-right: [w192] -> w169
            shift-left: w163 -> [w194]
            i -> [w193]
            n86 = Add(x=4 ("index"), y=w193) -> (x+y=w195:i32)
            n87 = Index Array(array=string[] ["Z1 Temp", "Z1 Set Pt", "Z2 Temp", "Z2 Set Pt", "Z3 Temp", "Z3 Set Pt", "Z4 Temp", "Z4 Set Pt", "Z5 Temp", "Z5 Set Pt", "Z6 Temp", "Z6 Set Pt", "Z7 Temp", "Z7 Set Pt", "Z8 Temp", "Z8 Set Pt", "Z9 Temp", "Z9 Set Pt"], index=w193) -> (element=w197:string)
            n88 = Replace Array Subset(array=w194, new element=w197, index=w195) -> (w192:string[])
          }
          n89 = for {
            N: w164 -> [_]
            tunnel: w185 -> [w233]
            tunnel: w167 -> [w227]
            tunnel: [w223] -> w165
            i -> [w230]
            n90 = Index Array(array=w233, index (row)=w230, index (col)=0 ("disabled index (col)")) -> ()  [unwired: 1 out]
            n91 = property on="Property Node" class="LstBox (strict)"(reference=w227, "CellFontSize"=u32 20 ("Active Row:Cell Font:Size")) -> (reference out=w226:refnum<vi>)  [unwired: 1 in, 1 out]
            n92 = property on="Property Node" class="LstBox (strict)"(reference=w226, "CellFontBold"=TRUE ("Active Row:Cell Font:Bold")) -> (reference out=w225:refnum<vi>)  [unwired: 1 in, 1 out]
            n93 = property on="Property Node" class="LstBox (strict)"(reference=w225, "Active Row"=w230) -> (reference out=w224:refnum<vi>)  [unwired: 1 in, 1 out]
            n94 = property on="Property Node" class="LstBox (strict)"(reference=w224, "CellBG"=u32 13816530 ("Active Row:Cell Background Color")) -> (reference out=w223:refnum<vi>)  [unwired: 1 in, 1 out]
          }
          n95 = Initialize Array(37, w164) -> (w181:i32[])
          n96 = property on="Property Node" class="LstBox (strict)"(reference=w165, "Item Symbols"=w181) -> ()  [unwired: 1 in, 2 out]
          n97 = property on="Property Node" class="LstBox (strict)"(reference=w165, "Item Names"=w169) -> ()  [unwired: 1 in, 2 out]
        }
        n98 = call-poly "Send Message.vi"("error in (no error)"=w151, "event buffer"="1000", "event"="multipleGraphs") -> ("error out"=w150:errorcluster)  [unwired: 8 in]
      }
      frame "initThermalProfile" {
        w241 = T25 {"time"="", "TCs"=[]} ("Cluster")
        n99 = Unbundle By Name(w240) -> ("Http session"=w247:T12, "URL prefex"=w245:string)
        n100 = Concatenate Strings(w245, "getAllThermoCoupleData" ("url")) -> (w246:string)
        n101 = call <vilib>:"GET.vi"("client handle"=w247, "url"=w246, "error in (no error)"=w239) -> ("body"=w243:string, "error out"=w236:errorcluster)  [unwired: 9 in, 2 out]
        n102 = Flatten To JSON(anything=w241) -> ()  [unwired: 2 in, 2 out]
        n103 = Unflatten From JSON(JSON string=w243, type and defaults=w241) -> (value=w242:T25)  [unwired: 5 in, 1 out]
        n104 = for {
          N: 9 ("Numeric") -> [_]
          tunnel: w242 -> [w265]
          tunnel: w240 -> [w264]
          i -> [w255]
          n105 = case shown="8" w255 {
            tunnel: [w267 w268 w269 w270 w271 w272 w273 w274 w275] -> w256
            frame 0, Default {
              n106 = control-ref of="Zone Thermocouples"() -> (w267:refnum<vi>)
            }
            frame 1 {
              n107 = control-ref of="Zone Thermocouples"() -> (w268:refnum<vi>)
            }
            frame 2 {
              n108 = control-ref of="Zone Thermocouples"() -> (w269:refnum<vi>)
            }
            frame 3 {
              n109 = control-ref of="Zone Thermocouples"() -> (w270:refnum<vi>)
            }
            frame 4 {
              n110 = control-ref of="Zone Thermocouples"() -> (w271:refnum<vi>)
            }
            frame 5 {
              n111 = control-ref of="Zone Thermocouples"() -> (w272:refnum<vi>)
            }
            frame 6 {
              n112 = control-ref of="Zone Thermocouples"() -> (w273:refnum<vi>)
            }
            frame 7 {
              n113 = control-ref of="Zone Thermocouples"() -> (w274:refnum<vi>)
            }
            frame 8 {
              n114 = control-ref of="Zone Thermocouples"() -> (w275:refnum<vi>)
            }
          }
          n115 = Unbundle By Name(w265) -> ("TCs"=w261:T10)
          n116 = Unbundle By Name(w264) -> ("NumberTCs"=w250:i32, "Thermocouples"=w266:T3, "numSensors"=w253:i32)
          n117 = Add(x=w250, y=1 ("index")) -> (x+y=w248:i32)
          n118 = Initialize Array("", w248) -> (w259:string[])
          n119 = Replace Array Subset(array=w259, new element="Clear Selection" ("new element/subarray"), index=0) -> (w252:string[])
          n120 = for {
            N: w250 -> [_]
            tunnel: w261 -> [w282] mode=indexing
            shift-right: [w276] -> w251
            shift-left: w252 -> [w278]
            i -> [w280]
            n121 = Unbundle By Name(w282) -> ("thermocouple"=w283:i32)
            n122 = Number To Decimal String(number=w283) -> (decimal integer string=w285:string)  [unwired: 1 in]
            n123 = Add(x=1 ("index"), y=w280) -> (x+y=w279:i32)
            n124 = Concatenate Strings("TC " ("string"), w285) -> (w277:string)
            n125 = Replace Array Subset(array=w278, new element=w277, index=w279) -> (w276:string[])
          }
          n126 = for {
            N: w253 -> [_]
            tunnel: w266 -> [w296]
            tunnel: w256 -> [w290]
            tunnel: [w286] -> w254
            i -> [w293]
            n127 = Index Array(array=w296, index (row)=w293, index (col)=0 ("disabled index (col)")) -> ()  [unwired: 1 out]
            n128 = property on="Property Node" class="LstBox (strict)"(reference=w290, "CellFontSize"=u32 20 ("Active Row:Cell Font:Size")) -> (reference out=w289:refnum<vi>)  [unwired: 1 in, 1 out]
            n129 = property on="Property Node" class="LstBox (strict)"(reference=w289, "CellFontBold"=TRUE ("Active Row:Cell Font:Bold")) -> (reference out=w288:refnum<vi>)  [unwired: 1 in, 1 out]
            n130 = property on="Property Node" class="LstBox (strict)"(reference=w288, "Active Row"=w293) -> (reference out=w287:refnum<vi>)  [unwired: 1 in, 1 out]
            n131 = property on="Property Node" class="LstBox (strict)"(reference=w287, "CellBG"=u32 13816530 ("Active Row:Cell Background Color")) -> (reference out=w286:refnum<vi>)  [unwired: 1 in, 1 out]
          }
          n132 = Initialize Array(37, w253) -> (w262:i32[])
          n133 = property on="Property Node" class="LstBox (strict)"(reference=w254, "Item Symbols"=w262) -> ()  [unwired: 1 in, 2 out]
          n134 = property on="Property Node" class="LstBox (strict)"(reference=w254, "Item Names"=w251) -> ()  [unwired: 1 in, 2 out]
        }
        n135 = call-poly "Send Message.vi"("error in (no error)"=w236, "event buffer"="1000", "event"="multipleGraphs") -> ("error out"=w235:errorcluster)  [unwired: 8 in]
      }
      frame "", "Idle" {
        n136 = Unbundle By Name(w301) -> ("Moving 1"=w300:bool)
        n137 = control-ref of="Thermocouples"() -> (w312:refnum<vi>)
        n138 = property on="Property Node" class="Arr (strict)"(reference=w312) -> ("Position"=w311:T1)  [unwired: 1 in, 2 out]
        n139 = Unbundle By Name(w311) -> ("Left"=w310:i32, "Top"=w308:i32)
        n140 = Add(x=4, y=w310) -> (x+y=w306:i32)
        n141 = Add(x=w308, y=23 ("x")) -> (x+y=w305:i32)
        n142 = event shown="[6] \"Custom Chart 6 Selection\": Mouse Down" {
          selector: _ -> [_ _ _ _ _ _ _ _ _ _ _ _ _ _ _ _ _ _ _ _ _ _ _ _ _ _ _ _ _ _ _ _ _ _ _ _ _ _ _ _ _ _ _ _ _ _ _ _]
          dyn-events: _ -> [_ _ _ _ _ _ _ _ _ _ _ _ _ _ _ _ _ _ _ _ _ _ _ _ _ _ _ _ _ _ _ _ _ _ _ _ _ _ _ _ _ _ _ _ _ _ _ _]
          timeout: 200 ("milliseconds to wait") -> [_ _ _ _ _ _ _ _ _ _ _ _ _ _ _ _ _ _ _ _ _ _ _ _ _ _ _ _ _ _ _ _ _ _ _ _ _ _ _ _ _ _ _ _ _ _ _ _]
          tunnel: [w328 w388 w402 w416 w430 w444 w458 w468 w484 w577 w641 w702 w763 w824 w885 w946 w1007 w1064 w1076 w1122 w1138 w1146 w1147 w1153 w1159 w1165 w1171 w1183 w1267 w1299 w1344 w1386 w1417 w1444 w1525 w1579 w1633 w1687 w1741 w1795 w1849 w1903 w1957 w2007 w2063 w2066 w2074 w2077] -> w302
          tunnel: [w321 w390 w404 w418 w432 w446 w460 w473 w485 w571 w642 w703 w764 w825 w886 w947 w1008 w1069 w1086 w1112 w1132 w1144 w1152 w1158 w1164 w1170 w1174 w1178 w1263 w1295 w1342 w1384 w1412 w1447 w1524 w1578 w1632 w1686 w1740 w1794 w1848 w1902 w1956 w2008 w2062 w2067 w2069 w2080] -> w299
          tunnel: w301 -> [w322 w390 w404 w418 w432 w446 w460 w473 w486 w573 w642 w703 w764 w825 w886 w947 w1008 w1070 w1075 w1113 w1133 w1145 w1152 w1158 w1164 w1170 w1174 w1179 w1264 w1296 w1343 w1385 w1413 w1447 w1524 w1578 w1632 w1686 w1740 w1794 w1848 w1902 w1956 w2008 w2062 w2067 w2069 w2080]
          tunnel: w306 -> [_ _ _ _ _ _ _ _ w483 _ _ _ _ _ _ _ _ _ _ _ _ _ _ _ _ _ _ _ _ _ _ _ _ _ _ _ _ _ _ _ _ _ _ _ _ _ _ _]
          tunnel: w305 -> [_ _ _ _ _ _ _ _ w480 _ _ _ _ _ _ _ _ _ _ _ _ _ _ _ _ _ _ _ _ _ _ _ _ _ _ _ _ _ _ _ _ _ _ _ _ _ _ _]
          tunnel: w303 -> [w317 w389 w403 w417 w431 w445 w459 w469 w484 w577 w641 w702 w763 w824 w885 w946 w1007 w1073 w1077 w1122 w1138 w1146 w1148 w1154 w1160 w1166 w1172 w1184 w1267 w1299 w1344 w1386 w1417 w1444 w1525 w1579 w1633 w1687 w1741 w1795 w1849 w1903 w1957 w2010 w2063 w2066 w2074 w2079]
          tunnel: w300 -> [_ _ _ _ _ _ _ _ _ _ _ _ _ _ _ _ _ _ _ _ _ _ _ _ _ _ _ _ _ _ _ _ _ _ _ _ _ _ _ _ _ _ _ w2009 _ _ _ _]
          tunnel: [_ _ _ _ _ _ _ _ _ _ _ _ _ _ _ _ _ _ _ _ _ _ _ _ _ _ _ _ _ _ _ _ _ _ _ _ _ _ _ _ _ _ _ w2009 FALSE TRUE _ _] -> w297
          event Timeout {
            n143 = event-data() -> ("Time"=w320:u32)  [unwired: 1 in, 1 out]
            n144 = Unbundle By Name(w322) -> ("Time"=w325:i32)
            n145 = Subtract(x=w320, y=w325) -> (x-y=w324:u32)
            n146 = Greater?(x=w324, y=u32 5000 ("millisecond multiple")) -> (0:w313:bool)
            n147 = case shown="True" w313 {
              tunnel: w322 -> [w330 w348]
              tunnel: [w330 w347] -> w321
              tunnel: w320 -> [_ w346]
              tunnel: [w329 w332] -> w319
              tunnel: w317 -> [w329 w345]
              frame False {
              }
              frame True {
                n148 = case shown="True" "TCs On" {
                  tunnel: w345 -> [w354 w358]
                  tunnel: [w354 w356] -> w344
                  frame False {
                  }
                  frame True {
                    n149 = call-poly "Send Message.vi"("Destination Module"="getData.vi", "error in (no error)"=w358, "event"="getTC") -> ("error out"=w356:errorcluster)  [unwired: 8 in]
                  }
                }
                n150 = Bundle By Name(cluster=w348, "Time"=w346) -> (w347:T13)
                n151 = case shown="True" "Pressure On" {
                  tunnel: w344 -> [w374 w377]
                  tunnel: [w374 w375] -> w343
                  frame False {
                  }
                  frame True {
                    n152 = call-poly "Send Message.vi"("Destination Module"="getData.vi", "error in (no error)"=w377, "event"="getPressure") -> ("error out"=w375:errorcluster)  [unwired: 8 in]
                  }
                }
                n153 = case shown="True" "MCC On" {
                  tunnel: w343 -> [w369 w371]
                  tunnel: [w369 w370] -> w342
                  frame False {
                  }
                  frame True {
                    n154 = call-poly "Send Message.vi"("Destination Module"="getData.vi", "error in (no error)"=w371, "event"="getMCCData") -> ("error out"=w370:errorcluster)  [unwired: 8 in]
                  }
                }
                n155 = case shown="True" "ZoneTemps On" {
                  tunnel: w342 -> [w364 w368]
                  tunnel: [w364 w365] -> w341
                  frame False {
                  }
                  frame True {
                    n156 = call-poly "Send Message.vi"("Destination Module"="getData.vi", "error in (no error)"=w368, "event"="getZoneTemps") -> ("error out"=w365:errorcluster)  [unwired: 8 in]
                  }
                }
                n157 = case shown="True" "Compressor On" {
                  tunnel: w341 -> [w359 w361]
                  tunnel: [w359 w360] -> w340
                  frame False {
                  }
                  frame True {
                    n158 = call-poly "Send Message.vi"("Destination Module"="getData.vi", "error in (no error)"=w361, "event"="getCompressorTemp") -> ("error out"=w360:errorcluster)  [unwired: 8 in]
                  }
                }
                n159 = case shown="True" "GetError" {
                  tunnel: w340 -> [w379 w381]
                  tunnel: [w379 w380] -> w333
                  frame False {
                  }
                  frame True {
                    n160 = call-poly "Send Message.vi"("Destination Module"="getData.vi", "error in (no error)"=w381, "event"="getLastError") -> ("error out"=w380:errorcluster)  [unwired: 8 in]
                  }
                }
                n161 = case shown="True" "GetEvent" {
                  tunnel: w333 -> [w349 w352]
                  tunnel: [w349 w351] -> w332
                  frame False {
                  }
                  frame True {
                    n162 = call-poly "Send Message.vi"("Destination Module"="getData.vi", "error in (no error)"=w352, "event"="getLastEvent") -> ("error out"=w351:errorcluster)  [unwired: 8 in]
                  }
                }
              }
            }
            n163 = call-poly "Send Message.vi"("error in (no error)"=w319, "event"="masterDatabase") -> ("error out"=w316:errorcluster)  [unwired: 9 in]
            n164 = call-poly "Send Message.vi"("error in (no error)"=w316, "event"="graphTC") -> ("error out"=w315:errorcluster)  [unwired: 9 in]
            n165 = call-poly "Send Message.vi"("error in (no error)"=w315, "event buffer"="1000", "event"="multipleGraphs") -> ("error out"=w328:errorcluster)  [unwired: 8 in]
          }
          event "Custom Chart 1 Selection": Mouse Down {
            n166 = event-data() -> ("CtlRef"=w387:refnum<vi>, "Coords"=w386:T26)  [unwired: 1 in, 6 out]
            n167 = invoke on="Invoke Node" class="LstBox (strict)" method="Point To Row"(reference=w387, "Point"=w386) -> ("InBounds"=w384:bool, "Row"=w385:i32)  [unwired: 5 in, 5 out]
            n168 = case shown="True" w384 {
              tunnel: w389 -> [w391 w397]
              tunnel: [w391 w396] -> w388
              tunnel: w385 -> [_ w392]
              frame False {
              }
              frame True {
                n169 = local write "Custom Graph Selector"(0) -> ()
                n170 = Number To Decimal String(number=w392) -> (decimal integer string=w394:string)  [unwired: 1 in]
                n171 = call-poly "Send Message.vi"("error in (no error)"=w397, "event buffer"=w394, "event"="multipleGraphs") -> ("error out"=w396:errorcluster)  [unwired: 8 in]
              }
            }
          }
          event "Custom Chart 2 Selection": Mouse Down {
            n172 = event-data() -> ("CtlRef"=w401:refnum<vi>, "Coords"=w400:T26)  [unwired: 1 in, 6 out]
            n173 = invoke on="Invoke Node" class="LstBox (strict)" method="Point To Row"(reference=w401, "Point"=w400) -> ("InBounds"=w398:bool, "Row"=w399:i32)  [unwired: 5 in, 5 out]
            n174 = case shown="True" w398 {
              tunnel: w403 -> [w405 w411]
              tunnel: [w405 w410] -> w402
              tunnel: w399 -> [_ w406]
              frame False {
              }
              frame True {
                n175 = local write "Custom Graph Selector"(1) -> ()
                n176 = Number To Decimal String(number=w406) -> (decimal integer string=w408:string)  [unwired: 1 in]
                n177 = call-poly "Send Message.vi"("error in (no error)"=w411, "event buffer"=w408, "event"="multipleGraphs") -> ("error out"=w410:errorcluster)  [unwired: 8 in]
              }
            }
          }
          event "Custom Chart 3 Selection": Mouse Down {
            n178 = event-data() -> ("CtlRef"=w415:refnum<vi>, "Coords"=w414:T26)  [unwired: 1 in, 6 out]
            n179 = invoke on="Invoke Node" class="LstBox (strict)" method="Point To Row"(reference=w415, "Point"=w414) -> ("InBounds"=w412:bool, "Row"=w413:i32)  [unwired: 5 in, 5 out]
            n180 = case shown="False" w412 {
              tunnel: w417 -> [w419 w425]
              tunnel: [w419 w424] -> w416
              tunnel: w413 -> [_ w420]
              frame False {
              }
              frame True {
                n181 = local write "Custom Graph Selector"(2) -> ()
                n182 = Number To Decimal String(number=w420) -> (decimal integer string=w422:string)  [unwired: 1 in]
                n183 = call-poly "Send Message.vi"("error in (no error)"=w425, "event buffer"=w422, "event"="multipleGraphs") -> ("error out"=w424:errorcluster)  [unwired: 8 in]
              }
            }
          }
          event "Custom Chart 4 Selection": Mouse Down {
            n184 = event-data() -> ("CtlRef"=w429:refnum<vi>, "Coords"=w428:T26)  [unwired: 1 in, 6 out]
            n185 = invoke on="Invoke Node" class="LstBox (strict)" method="Point To Row"(reference=w429, "Point"=w428) -> ("InBounds"=w426:bool, "Row"=w427:i32)  [unwired: 5 in, 5 out]
            n186 = case shown="False" w426 {
              tunnel: w431 -> [w433 w439]
              tunnel: [w433 w438] -> w430
              tunnel: w427 -> [_ w434]
              frame False {
              }
              frame True {
                n187 = local write "Custom Graph Selector"(3) -> ()
                n188 = Number To Decimal String(number=w434) -> (decimal integer string=w436:string)  [unwired: 1 in]
                n189 = call-poly "Send Message.vi"("error in (no error)"=w439, "event buffer"=w436, "event"="multipleGraphs") -> ("error out"=w438:errorcluster)  [unwired: 8 in]
              }
            }
          }
          event "Custom Chart 5 Selection": Mouse Down {
            n190 = event-data() -> ("CtlRef"=w443:refnum<vi>, "Coords"=w442:T26)  [unwired: 1 in, 6 out]
            n191 = invoke on="Invoke Node" class="LstBox (strict)" method="Point To Row"(reference=w443, "Point"=w442) -> ("InBounds"=w440:bool, "Row"=w441:i32)  [unwired: 5 in, 5 out]
            n192 = case shown="False" w440 {
              tunnel: w445 -> [w447 w453]
              tunnel: [w447 w452] -> w444
              tunnel: w441 -> [_ w448]
              frame False {
              }
              frame True {
                n193 = Number To Decimal String(number=w448) -> (decimal integer string=w450:string)  [unwired: 1 in]
                n194 = local write "Custom Graph Selector"(4) -> ()
                n195 = call-poly "Send Message.vi"("error in (no error)"=w453, "event buffer"=w450, "event"="multipleGraphs") -> ("error out"=w452:errorcluster)  [unwired: 8 in]
              }
            }
          }
          event "Custom Chart 6 Selection": Mouse Down {
            n196 = event-data() -> ("CtlRef"=w457:refnum<vi>, "Coords"=w456:T26)  [unwired: 1 in, 6 out]
            n197 = invoke on="Invoke Node" class="LstBox (strict)" method="Point To Row"(reference=w457, "Point"=w456) -> ("InBounds"=w454:bool, "Row"=w455:i32)  [unwired: 5 in, 5 out]
            n198 = case shown="False" w454 {
              tunnel: w459 -> [w461 w467]
              tunnel: [w461 w466] -> w458
              tunnel: w455 -> [_ w462]
              frame False {
              }
              frame True {
                n199 = local write "Custom Graph Selector"(5) -> ()
                n200 = Number To Decimal String(number=w462) -> (decimal integer string=w464:string)  [unwired: 1 in]
                n201 = call-poly "Send Message.vi"("error in (no error)"=w467, "event buffer"=w464, "event"="multipleGraphs") -> ("error out"=w466:errorcluster)  [unwired: 8 in]
              }
            }
          }
          event "Tab Control": Value Change {
            n202 = event-data() -> ("NewVal"=w472:T2)  [unwired: 1 in, 5 out]
            n203 = Equal?(x=w472, y=enum16{"Graphs"}."Graphs") -> (x = y?=w470:bool)
            n204 = case shown="True" w470 {
              tunnel: w469 -> [w474 w476]
              tunnel: [w474 w475] -> w468
              frame False {
              }
              frame True {
                n205 = call-poly "Send Message.vi"("error in (no error)"=w476, "event"="getGraphs") -> ("error out"=w475:errorcluster)  [unwired: 9 in]
              }
            }
          }
          event "Thermocouples": Mouse Down {
            n206 = event-data() -> ("CtlRef"=w488:refnum<vi>, "Coords"=w493:T26)  [unwired: 1 in, 3 out]
            n207 = Unbundle By Name(w493) -> ("Horizontal"=w491:i32, "Vertical"=w490:i32)
            n208 = Add(x=783 ("y"), y=w483) -> (x+y=w478:i32)
            n209 = Less?(x=w491, y=w478) -> (x < y?=w492:bool)
            n210 = Add(x=w480, y=854) -> (x+y=w479:i32)
            n211 = Less?(x=w490, y=w479) -> (x < y?=w489:bool)
            n212 = And(x=w492, y=w489) -> (x .and. y?=w487:bool)
            n213 = case shown="True" w487 {
              tunnel: w488 -> [_ w535]
              tunnel: w486 -> [_ w507]
              tunnel: w486 -> [w494 w505]
              tunnel: [w494 w497] -> w485
              tunnel: w483 -> [_ w496]
              tunnel: w480 -> [_ w495]
              frame False {
              }
              frame True {
                w529 = u16 0 items=["User Selection", "Graph All Thermocouples", "Clear Graph"] ("Graphing Selection")
                n214 = property class="Arr (strict)"(reference=w535) -> ("Array Element.Position"=w527:T1)  [unwired: 1 in, 2 out]
                n215 = local write "Graphing Selection"(w529) -> ()
                n216 = Unbundle By Name(w527) -> ("Left"=w525:i32, "Top"=w528:i32)
                n217 = property on="Thermocouples" class="Arr (strict)"() -> ("Index Values"=w519:u32[])  [unwired: 2 in, 2 out]
                n218 = Subtract(x=w496, y=w525) -> (x-y=w524:i32)
                n219 = Subtract(x=w495, y=w528) -> (x-y=w516:i32)
                n220 = Absolute Value(x=w516) -> (abs(x)=w526:i32)
                n221 = Index Array(array=w519, index=0) -> (element=w515:u32)
                n222 = To Byte Integer(number=w515) -> (8bit integer=w514:i8)
                n223 = Absolute Value(x=w524) -> (abs(x)=w523:i32)
                n224 = local read "Thermocouples"() -> (w498:T3)
                n225 = Quotient & Remainder(x=w526, y=42) -> (floor(x/y)=w513:i32)  [unwired: 1 out]
                n226 = Add(x=w514, y=w513) -> (x+y=w500:i32)
                n227 = Quotient & Remainder(x=w523, y=197 ("Numeric 2")) -> (floor(x/y)=w499:i32)  [unwired: 1 out]
                n228 = Index Array(array=w498, index (row)=w500, index (col)=w499) -> (element=w501:T14)
                n229 = Multiply(x=4, y=w500) -> (x*y=w520:i32)
                n230 = Unbundle By Name(w507) -> ("working array"=w506:bool[])  [unwired: 1 out]
                n231 = Unbundle By Name(w501) -> ("Alarm Color"=w533:u32, "Graph On/Off"=w532:u32, "TC Label"=w531:string, "PlotColor"=w512:u32, "Alarm Status"=w530:string, "Temperature"=w503:string)
                n232 = Add(x=w520, y=w499) -> (x+y=w509:i32)
                n233 = control-ref of="Waveform Chart"() -> (w534:refnum<vi>)
                n234 = Index Array(array=w506, index=w509) -> (element=w508:bool)
                n235 = Decimal String To Number(string=w503) -> ()  [unwired: 2 in, 2 out]
                n236 = Equal?(x=w532, y=u32 12369084) -> (x = y?=w510:bool)
                n237 = case shown="True" w508 {
                  selector: w508 -> [_ w541]
                  tunnel: w534 -> [_ w547]
                  tunnel: w533 -> [_ w546]
                  tunnel: w531 -> [_ w545]
                  tunnel: w530 -> [_ w544]
                  tunnel: w509 -> [_ w537]
                  tunnel: w512 -> [_ w543]
                  tunnel: w510 -> [_ w542]
                  tunnel: w503 -> [_ w540]
                  tunnel: [w536 w539] -> w502
                  tunnel: w501 -> [w536 w538]
                  frame False {
                  }
                  frame True {
                    n238 = case shown="True" w542 {
                      tunnel: w547 -> [w557 w568]
                      tunnel: w546 -> [w551 w563]
                      tunnel: w545 -> [w552 w562]
                      tunnel: w544 -> [w553 w564]
                      tunnel: w543 -> [_ w566]
                      tunnel: w541 -> [_ _]
                      tunnel: w540 -> [w554 w565]
                      tunnel: [w549 w561] -> w539
                      tunnel: w538 -> [w550 w560]
                      tunnel: w537 -> [w548 w559]
                      frame False {
                        w555 = u32 12369084
                        n239 = property on="Property Node" class="WFChart (strict)"(reference=w557, "Active Plot"=w548) -> (reference out=w558:refnum<vi>)  [unwired: 1 in, 1 out]
                        n240 = Bundle By Name(cluster=w550, "Graph On/Off"=w555, "TC Label"=w552, "PlotColor"=w555, "Temperature"=w554, "Alarm Color"=w551, "Alarm Status"=w553) -> (w549:T14)
                        n241 = property class="WFChart (strict)"(reference=w558, "Plot.Visible?"=FALSE ("Plot.Visible")) -> ()  [unwired: 1 in, 2 out]
                      }
                      frame True {
                        n242 = property class="WFChart (strict)"(reference=w568, "Active Plot"=w559) -> (reference out=w569:refnum<vi>)  [unwired: 1 in, 1 out]
                        n243 = Bundle By Name(cluster=w560, "Graph On/Off"=u32 6618880, "TC Label"=w562, "PlotColor"=w566, "Temperature"=w565, "Alarm Color"=w563, "Alarm Status"=w564) -> (w561:T14)
                        n244 = property class="WFChart (strict)"(reference=w569, "Plot.Visible?"=TRUE ("Plot.Visible")) -> ()  [unwired: 1 in, 2 out]
                      }
                    }
                  }
                }
                n245 = Replace Array Subset(array=w498, new element=w502, index (row)=w500, index (col)=w499) -> (w504:T3)
                n246 = Bundle By Name(cluster=w505, "Thermocouples"=w504) -> (w497:T13)
              }
            }
          }
          event "Graphing Selection": Value Change {
            n247 = event-data() -> ("NewVal"=w578:u16)  [unwired: 1 in, 5 out]
            n248 = Unbundle By Name(w573) -> ("Thermocouples"=w572:T3, "working array"=w575:bool[])
            n249 = control-ref of="Waveform Chart"() -> (w579:refnum<vi>)
            n250 = case shown="1" w578 {
              tunnel: w572 -> [w580 w585 w616]
              tunnel: w579 -> [_ w584 w615]
              tunnel: 120 ("disabled index (col)") -> [_ w583 w614]
              tunnel: w573 -> [_ _ _]
              tunnel: w575 -> [_ w582 _]
              tunnel: [w580 w581 w613] -> w574
              frame 0, Default {
              }
              frame 1 {
                n251 = for {
                  N: w583 -> [_]
                  tunnel: w584 -> [w591]
                  shift-right: [w586] -> w581
                  shift-left: w585 -> [w590]
                  tunnel: w582 -> [w587]
                  i -> [w589]
                  n252 = Index Array(array=w587, index=w589) -> (element=w588:bool)
                  n253 = case shown="True" w588 {
                    tunnel: w591 -> [_ w612]
                    tunnel: w590 -> [w592 w593]
                    tunnel: [w592 w594] -> w586
                    tunnel: w589 -> [_ w611]
                    frame False {
                    }
                    frame True {
                      n254 = Quotient & Remainder(x=w611, y=4) -> (x-y*floor(x/y)=w597:i32, floor(x/y)=w596:i32)
                      n255 = Multiply(x=4, y=w596) -> (x*y=w607:i32)
                      n256 = Add(x=w607, y=w597) -> (x+y=w606:i32)
                      n257 = property class="WFChart (strict)"(reference=w612, "Active Plot"=w606) -> (reference out=w609:refnum<vi>)  [unwired: 1 in, 1 out]
                      n258 = Index Array(array=w593, index (row)=w596, index (col)=w597) -> (element=w595:T14)
                      n259 = Unbundle By Name(w595) -> ("TC Label"=w598:string, "Alarm Status"=w604:string, "Temperature"=w603:string, "PlotColor"=w600:u32, "Alarm Color"=w599:u32)
                      n260 = property class="WFChart (strict)"(reference=w609, "Plot.Visible?"=TRUE ("Plot.Visible")) -> ()  [unwired: 1 in, 2 out]
                      n261 = Bundle By Name(cluster=w595, "TC Label"=w598, "Alarm Status"=w604, "Alarm Color"=w599, "Temperature"=w603, "PlotColor"=w600, "Graph On/Off"=u32 6618880) -> (w602:T14)
                      n262 = Replace Array Subset(array=w593, new element=w602, index (row)=w596, index (col)=w597) -> (w594:T3)
                    }
                  }
                }
              }
              frame 2 {
                n263 = for {
                  N: w614 -> [_]
                  tunnel: w615 -> [w634]
                  shift-right: [w617] -> w613
                  shift-left: w616 -> [w621]
                  i -> [w635]
                  w627 = u32 12369084
                  n264 = local read "working array"() -> (w636:bool[])
                  n265 = Quotient & Remainder(x=w635, y=4 ("Numeric")) -> (x-y*floor(x/y)=w619:i32, floor(x/y)=w618:i32)
                  n266 = Index Array(array=w621, index (row)=w618, index (col)=w619) -> (element=w626:T14)
                  n267 = Multiply(x=4, y=w618) -> (x*y=w630:i32)
                  n268 = Add(x=w630, y=w619) -> (x+y=w629:i32)
                  n269 = Index Array(array=w636, index=w635) -> ()  [unwired: 1 out]
                  n270 = property class="WFChart (strict)"(reference=w634, "Active Plot"=w629) -> (reference out=w632:refnum<vi>)  [unwired: 1 in, 1 out]
                  n271 = Unbundle By Name(w626) -> ("TC Label"=w625:string, "Alarm Status"=w624:string, "Temperature"=w623:string, "PlotColor"=w622:u32)
                  n272 = property class="WFChart (strict)"(reference=w632, "Plot.Visible?"=FALSE ("Plot.Visible")) -> ()  [unwired: 1 in, 2 out]
                  n273 = Bundle By Name(cluster=w626, "TC Label"=w625, "Alarm Status"=w624, "Alarm Color"=w627, "Temperature"=w623, "PlotColor"=w622, "Graph On/Off"=w627) -> (w620:T14)
                  n274 = Replace Array Subset(array=w621, new element=w620, index (row)=w618, index (col)=w619) -> (w617:T3)
                }
              }
            }
            n275 = Bundle By Name(cluster=w573, "Thermocouples"=w574) -> (w571:T13)
          }
          event "Set Time TC Graph": Mouse Down {
            n276 = event-data() -> ()  [unwired: 1 in, 8 out]
            n277 = local read "Log/Linear Y-Axis"() -> (w638:u16)
            n278 = control-ref of="Waveform Chart"() -> (w637:refnum<vi>)
            n279 = property on="Property Node" class="WFChart (strict)"(reference=w637, "YScale.Mapping Mode"=w638) -> ()  [unwired: 1 in, 2 out]
            n280 = local read "Total Time"() -> (w639:dbl)
            n281 = local read "Time Scale"() -> (w640:u16)
            n282 = case shown="2" w640 {
              tunnel: w637 -> [w645 w664 w683]
              tunnel: w639 -> [w643 w662 w681]
              frame 0, Default {
                n283 = Not Equal To 0?(x=w643) -> (x != 0?=w644:bool)
                n284 = case shown="True" w644 {
                  tunnel: w645 -> [w647 w659]
                  tunnel: w643 -> [_ w653]
                  frame False {
                    n285 = property on="Property Node" class="WFChart (strict)"(reference=w647) -> (reference out=w646:refnum<vi>, "XScale.Range"=w652:T27)  [unwired: 1 in, 1 out]
                    n286 = Bundle By Name(cluster=w652, "Minimum"=0.0, "Maximum"=3600.0, "Increment"=60.0) -> (w651:T27)
                    n287 = property on="Property Node" class="WFChart (strict)"(reference=w646, "XScale.Range"=w651) -> ()  [unwired: 1 in, 2 out]
                  }
                  frame True {
                    n288 = property on="Property Node" class="WFChart (strict)"(reference=w659) -> (reference out=w656:refnum<vi>, "XScale.Range"=w661:T27)  [unwired: 1 in, 1 out]
                    n289 = Multiply(x=w653, y=60.0) -> (x*y=w655:dbl)
                    n290 = Bundle By Name(cluster=w661, "Minimum"=0.0, "Maximum"=w655, "Increment"=1.0) -> (w660:T27)
                    n291 = property on="Property Node" class="WFChart (strict)"(reference=w656, "XScale.Range"=w660) -> ()  [unwired: 1 in, 2 out]
                  }
                }
              }
              frame 1 {
                n292 = Not Equal To 0?(x=w662) -> (x != 0?=w663:bool)
                n293 = case shown="True" w663 {
                  tunnel: w664 -> [w666 w676]
                  tunnel: w662 -> [_ w673]
                  frame False {
                    n294 = property on="Property Node" class="WFChart (strict)"(reference=w666) -> (reference out=w665:refnum<vi>, "XScale.Range"=w671:T27)  [unwired: 1 in, 1 out]
                    n295 = Bundle By Name(cluster=w671, "Minimum"=0.0, "Maximum"=43200.0, "Increment"=3600.0) -> (w667:T27)
                    n296 = property on="Property Node" class="WFChart (strict)"(reference=w665, "XScale.Range"=w667) -> ()  [unwired: 1 in, 2 out]
                  }
                  frame True {
                    n297 = Multiply(x=w673, y=3600.0) -> (x*y=w672:dbl)
                    n298 = property on="Property Node" class="WFChart (strict)"(reference=w676) -> (reference out=w675:refnum<vi>, "XScale.Range"=w680:T27)  [unwired: 1 in, 1 out]
                    n299 = Bundle By Name(cluster=w680, "Minimum"=0.0, "Maximum"=w672, "Increment"=3600.0) -> (w677:T27)
                    n300 = property on="Property Node" class="WFChart (strict)"(reference=w675, "XScale.Range"=w677) -> ()  [unwired: 1 in, 2 out]
                  }
                }
              }
              frame 2 {
                n301 = Not Equal To 0?(x=w681) -> (x != 0?=w682:bool)
                n302 = case shown="True" w682 {
                  tunnel: w683 -> [w685 w693]
                  tunnel: w681 -> [_ w691]
                  frame False {
                    n303 = property on="Property Node" class="WFChart (strict)"(reference=w685) -> (reference out=w684:refnum<vi>, "XScale.Range"=w690:T27)  [unwired: 1 in, 1 out]
                    n304 = Bundle By Name(cluster=w690, "Minimum"=0.0, "Maximum"=60.0, "Increment"=1.0) -> (w686:T27)
                    n305 = property on="Property Node" class="WFChart (strict)"(reference=w684, "XScale.Range"=w686) -> ()  [unwired: 1 in, 2 out]
                  }
                  frame True {
                    n306 = property on="Property Node" class="WFChart (strict)"(reference=w693) -> (reference out=w692:refnum<vi>, "XScale.Range"=w697:T27)  [unwired: 1 in, 1 out]
                    n307 = Bundle By Name(cluster=w697, "Minimum"=0.0, "Maximum"=w691, "Increment"=1.0) -> (w694:T27)
                    n308 = property on="Property Node" class="WFChart (strict)"(reference=w692, "XScale.Range"=w694) -> ()  [unwired: 1 in, 2 out]
                  }
                }
              }
            }
          }
          event "Set Time TC Graph 1": Mouse Down {
            n309 = event-data() -> ()  [unwired: 1 in, 8 out]
            n310 = local read "Log/Linear Y-Axis 1"() -> (w699:u16)
            n311 = control-ref of="Custom Chart 1"() -> (w698:refnum<vi>)
            n312 = property on="Property Node" class="WFChart (strict)"(reference=w698, "YScale.Mapping Mode"=w699) -> ()  [unwired: 1 in, 2 out]
            n313 = local read "Total Time 1"() -> (w700:dbl)
            n314 = local read "Time Scale 1"() -> (w701:u16)
            n315 = case shown="2" w701 {
              tunnel: w698 -> [w706 w725 w744]
              tunnel: w700 -> [w704 w723 w742]
              frame 0, Default {
                n316 = Not Equal To 0?(x=w704) -> (x != 0?=w705:bool)
                n317 = case shown="True" w705 {
                  tunnel: w706 -> [w708 w720]
                  tunnel: w704 -> [_ w714]
                  frame False {
                    n318 = property on="Property Node" class="WFChart (strict)"(reference=w708) -> (reference out=w707:refnum<vi>, "XScale.Range"=w713:T27)  [unwired: 1 in, 1 out]
                    n319 = Bundle By Name(cluster=w713, "Minimum"=0.0, "Maximum"=3600.0, "Increment"=60.0) -> (w712:T27)
                    n320 = property on="Property Node" class="WFChart (strict)"(reference=w707, "XScale.Range"=w712) -> ()  [unwired: 1 in, 2 out]
                  }
                  frame True {
                    n321 = property on="Property Node" class="WFChart (strict)"(reference=w720) -> (reference out=w717:refnum<vi>, "XScale.Range"=w722:T27)  [unwired: 1 in, 1 out]
                    n322 = Multiply(x=w714, y=60.0) -> (x*y=w716:dbl)
                    n323 = Bundle By Name(cluster=w722, "Minimum"=0.0, "Maximum"=w716, "Increment"=1.0) -> (w721:T27)
                    n324 = property on="Property Node" class="WFChart (strict)"(reference=w717, "XScale.Range"=w721) -> ()  [unwired: 1 in, 2 out]
                  }
                }
              }
              frame 1 {
                n325 = Not Equal To 0?(x=w723) -> (x != 0?=w724:bool)
                n326 = case shown="True" w724 {
                  tunnel: w725 -> [w727 w737]
                  tunnel: w723 -> [_ w734]
                  frame False {
                    n327 = property on="Property Node" class="WFChart (strict)"(reference=w727) -> (reference out=w726:refnum<vi>, "XScale.Range"=w732:T27)  [unwired: 1 in, 1 out]
                    n328 = Bundle By Name(cluster=w732, "Minimum"=0.0, "Maximum"=43200.0, "Increment"=3600.0) -> (w728:T27)
                    n329 = property on="Property Node" class="WFChart (strict)"(reference=w726, "XScale.Range"=w728) -> ()  [unwired: 1 in, 2 out]
                  }
                  frame True {
                    n330 = Multiply(x=w734, y=3600.0) -> (x*y=w733:dbl)
                    n331 = property on="Property Node" class="WFChart (strict)"(reference=w737) -> (reference out=w736:refnum<vi>, "XScale.Range"=w741:T27)  [unwired: 1 in, 1 out]
                    n332 = Bundle By Name(cluster=w741, "Minimum"=0.0, "Maximum"=w733, "Increment"=3600.0) -> (w738:T27)
                    n333 = property on="Property Node" class="WFChart (strict)"(reference=w736, "XScale.Range"=w738) -> ()  [unwired: 1 in, 2 out]
                  }
                }
              }
              frame 2 {
                n334 = Not Equal To 0?(x=w742) -> (x != 0?=w743:bool)
                n335 = case shown="True" w743 {
                  tunnel: w744 -> [w746 w754]
                  tunnel: w742 -> [_ w752]
                  frame False {
                    n336 = property on="Property Node" class="WFChart (strict)"(reference=w746) -> (reference out=w745:refnum<vi>, "XScale.Range"=w751:T27)  [unwired: 1 in, 1 out]
                    n337 = Bundle By Name(cluster=w751, "Minimum"=0.0, "Maximum"=60.0, "Increment"=1.0) -> (w747:T27)
                    n338 = property on="Property Node" class="WFChart (strict)"(reference=w745, "XScale.Range"=w747) -> ()  [unwired: 1 in, 2 out]
                  }
                  frame True {
                    n339 = property on="Property Node" class="WFChart (strict)"(reference=w754) -> (reference out=w753:refnum<vi>, "XScale.Range"=w758:T27)  [unwired: 1 in, 1 out]
                    n340 = Bundle By Name(cluster=w758, "Minimum"=0.0, "Maximum"=w752, "Increment"=1.0) -> (w755:T27)
                    n341 = property on="Property Node" class="WFChart (strict)"(reference=w753, "XScale.Range"=w755) -> ()  [unwired: 1 in, 2 out]
                  }
                }
              }
            }
          }
          event "Set Time TC Graph 2": Mouse Down {
            n342 = event-data() -> ()  [unwired: 1 in, 8 out]
            n343 = local read "Log/Linear Y-Axis 2"() -> (w760:u16)
            n344 = control-ref of="Custom Chart 2"() -> (w759:refnum<vi>)
            n345 = property on="Property Node" class="WFChart (strict)"(reference=w759, "YScale.Mapping Mode"=w760) -> ()  [unwired: 1 in, 2 out]
            n346 = local read "Total Time 2"() -> (w761:dbl)
            n347 = local read "Time Scale 2"() -> (w762:u16)
            n348 = case shown="2" w762 {
              tunnel: w759 -> [w767 w786 w805]
              tunnel: w761 -> [w765 w784 w803]
              frame 0, Default {
                n349 = Not Equal To 0?(x=w765) -> (x != 0?=w766:bool)
                n350 = case shown="True" w766 {
                  tunnel: w767 -> [w769 w781]
                  tunnel: w765 -> [_ w775]
                  frame False {
                    n351 = property on="Property Node" class="WFChart (strict)"(reference=w769) -> (reference out=w768:refnum<vi>, "XScale.Range"=w774:T27)  [unwired: 1 in, 1 out]
                    n352 = Bundle By Name(cluster=w774, "Minimum"=0.0, "Maximum"=3600.0, "Increment"=60.0) -> (w773:T27)
                    n353 = property on="Property Node" class="WFChart (strict)"(reference=w768, "XScale.Range"=w773) -> ()  [unwired: 1 in, 2 out]
                  }
                  frame True {
                    n354 = property on="Property Node" class="WFChart (strict)"(reference=w781) -> (reference out=w778:refnum<vi>, "XScale.Range"=w783:T27)  [unwired: 1 in, 1 out]
                    n355 = Multiply(x=w775, y=60.0) -> (x*y=w777:dbl)
                    n356 = Bundle By Name(cluster=w783, "Minimum"=0.0, "Maximum"=w777, "Increment"=1.0) -> (w782:T27)
                    n357 = property on="Property Node" class="WFChart (strict)"(reference=w778, "XScale.Range"=w782) -> ()  [unwired: 1 in, 2 out]
                  }
                }
              }
              frame 1 {
                n358 = Not Equal To 0?(x=w784) -> (x != 0?=w785:bool)
                n359 = case shown="True" w785 {
                  tunnel: w786 -> [w788 w798]
                  tunnel: w784 -> [_ w795]
                  frame False {
                    n360 = property on="Property Node" class="WFChart (strict)"(reference=w788) -> (reference out=w787:refnum<vi>, "XScale.Range"=w793:T27)  [unwired: 1 in, 1 out]
                    n361 = Bundle By Name(cluster=w793, "Minimum"=0.0, "Maximum"=43200.0, "Increment"=3600.0) -> (w789:T27)
                    n362 = property on="Property Node" class="WFChart (strict)"(reference=w787, "XScale.Range"=w789) -> ()  [unwired: 1 in, 2 out]
                  }
                  frame True {
                    n363 = Multiply(x=w795, y=3600.0) -> (x*y=w794:dbl)
                    n364 = property on="Property Node" class="WFChart (strict)"(reference=w798) -> (reference out=w797:refnum<vi>, "XScale.Range"=w802:T27)  [unwired: 1 in, 1 out]
                    n365 = Bundle By Name(cluster=w802, "Minimum"=0.0, "Maximum"=w794, "Increment"=3600.0) -> (w799:T27)
                    n366 = property on="Property Node" class="WFChart (strict)"(reference=w797, "XScale.Range"=w799) -> ()  [unwired: 1 in, 2 out]
                  }
                }
              }
              frame 2 {
                n367 = Not Equal To 0?(x=w803) -> (x != 0?=w804:bool)
                n368 = case shown="True" w804 {
                  tunnel: w805 -> [w807 w815]
                  tunnel: w803 -> [_ w813]
                  frame False {
                    n369 = property on="Property Node" class="WFChart (strict)"(reference=w807) -> (reference out=w806:refnum<vi>, "XScale.Range"=w812:T27)  [unwired: 1 in, 1 out]
                    n370 = Bundle By Name(cluster=w812, "Minimum"=0.0, "Maximum"=60.0, "Increment"=1.0) -> (w808:T27)
                    n371 = property on="Property Node" class="WFChart (strict)"(reference=w806, "XScale.Range"=w808) -> ()  [unwired: 1 in, 2 out]
                  }
                  frame True {
                    n372 = property on="Property Node" class="WFChart (strict)"(reference=w815) -> (reference out=w814:refnum<vi>, "XScale.Range"=w819:T27)  [unwired: 1 in, 1 out]
                    n373 = Bundle By Name(cluster=w819, "Minimum"=0.0, "Maximum"=w813, "Increment"=1.0) -> (w816:T27)
                    n374 = property on="Property Node" class="WFChart (strict)"(reference=w814, "XScale.Range"=w816) -> ()  [unwired: 1 in, 2 out]
                  }
                }
              }
            }
          }
          event "Set Time TC Graph 3": Mouse Down {
            n375 = event-data() -> ()  [unwired: 1 in, 8 out]
            n376 = local read "Log/Linear Y-Axis 3"() -> (w821:u16)
            n377 = control-ref of="Custom Chart 3"() -> (w820:refnum<vi>)
            n378 = property on="Property Node" class="WFChart (strict)"(reference=w820, "YScale.Mapping Mode"=w821) -> ()  [unwired: 1 in, 2 out]
            n379 = local read "Total Time 3"() -> (w822:dbl)
            n380 = local read "Time Scale 3"() -> (w823:u16)
            n381 = case shown="2" w823 {
              tunnel: w820 -> [w828 w847 w866]
              tunnel: w822 -> [w826 w845 w864]
              frame 0, Default {
                n382 = Not Equal To 0?(x=w826) -> (x != 0?=w827:bool)
                n383 = case shown="True" w827 {
                  tunnel: w828 -> [w830 w842]
                  tunnel: w826 -> [_ w836]
                  frame False {
                    n384 = property on="Property Node" class="WFChart (strict)"(reference=w830) -> (reference out=w829:refnum<vi>, "XScale.Range"=w835:T27)  [unwired: 1 in, 1 out]
                    n385 = Bundle By Name(cluster=w835, "Minimum"=0.0, "Maximum"=3600.0, "Increment"=60.0) -> (w834:T27)
                    n386 = property on="Property Node" class="WFChart (strict)"(reference=w829, "XScale.Range"=w834) -> ()  [unwired: 1 in, 2 out]
                  }
                  frame True {
                    n387 = property on="Property Node" class="WFChart (strict)"(reference=w842) -> (reference out=w839:refnum<vi>, "XScale.Range"=w844:T27)  [unwired: 1 in, 1 out]
                    n388 = Multiply(x=w836, y=60.0) -> (x*y=w838:dbl)
                    n389 = Bundle By Name(cluster=w844, "Minimum"=0.0, "Maximum"=w838, "Increment"=1.0) -> (w843:T27)
                    n390 = property on="Property Node" class="WFChart (strict)"(reference=w839, "XScale.Range"=w843) -> ()  [unwired: 1 in, 2 out]
                  }
                }
              }
              frame 1 {
                n391 = Not Equal To 0?(x=w845) -> (x != 0?=w846:bool)
                n392 = case shown="True" w846 {
                  tunnel: w847 -> [w849 w859]
                  tunnel: w845 -> [_ w856]
                  frame False {
                    n393 = property on="Property Node" class="WFChart (strict)"(reference=w849) -> (reference out=w848:refnum<vi>, "XScale.Range"=w854:T27)  [unwired: 1 in, 1 out]
                    n394 = Bundle By Name(cluster=w854, "Minimum"=0.0, "Maximum"=43200.0, "Increment"=3600.0) -> (w850:T27)
                    n395 = property on="Property Node" class="WFChart (strict)"(reference=w848, "XScale.Range"=w850) -> ()  [unwired: 1 in, 2 out]
                  }
                  frame True {
                    n396 = Multiply(x=w856, y=3600.0) -> (x*y=w855:dbl)
                    n397 = property on="Property Node" class="WFChart (strict)"(reference=w859) -> (reference out=w858:refnum<vi>, "XScale.Range"=w863:T27)  [unwired: 1 in, 1 out]
                    n398 = Bundle By Name(cluster=w863, "Minimum"=0.0, "Maximum"=w855, "Increment"=3600.0) -> (w860:T27)
                    n399 = property on="Property Node" class="WFChart (strict)"(reference=w858, "XScale.Range"=w860) -> ()  [unwired: 1 in, 2 out]
                  }
                }
              }
              frame 2 {
                n400 = Not Equal To 0?(x=w864) -> (x != 0?=w865:bool)
                n401 = case shown="True" w865 {
                  tunnel: w866 -> [w868 w876]
                  tunnel: w864 -> [_ w874]
                  frame False {
                    n402 = property on="Property Node" class="WFChart (strict)"(reference=w868) -> (reference out=w867:refnum<vi>, "XScale.Range"=w873:T27)  [unwired: 1 in, 1 out]
                    n403 = Bundle By Name(cluster=w873, "Minimum"=0.0, "Maximum"=60.0, "Increment"=1.0) -> (w869:T27)
                    n404 = property on="Property Node" class="WFChart (strict)"(reference=w867, "XScale.Range"=w869) -> ()  [unwired: 1 in, 2 out]
                  }
                  frame True {
                    n405 = property on="Property Node" class="WFChart (strict)"(reference=w876) -> (reference out=w875:refnum<vi>, "XScale.Range"=w880:T27)  [unwired: 1 in, 1 out]
                    n406 = Bundle By Name(cluster=w880, "Minimum"=0.0, "Maximum"=w874, "Increment"=1.0) -> (w877:T27)
                    n407 = property on="Property Node" class="WFChart (strict)"(reference=w875, "XScale.Range"=w877) -> ()  [unwired: 1 in, 2 out]
                  }
                }
              }
            }
          }
          event "Set Time TC Graph 4": Mouse Down {
            n408 = event-data() -> ()  [unwired: 1 in, 8 out]
            n409 = local read "Log/Linear Y-Axis 4"() -> (w882:u16)
            n410 = control-ref of="Custom Chart 4"() -> (w881:refnum<vi>)
            n411 = property on="Property Node" class="WFChart (strict)"(reference=w881, "YScale.Mapping Mode"=w882) -> ()  [unwired: 1 in, 2 out]
            n412 = local read "Total Time 4"() -> (w883:dbl)
            n413 = local read "Time Scale 4"() -> (w884:u16)
            n414 = case shown="2" w884 {
              tunnel: w881 -> [w889 w908 w927]
              tunnel: w883 -> [w887 w906 w925]
              frame 0, Default {
                n415 = Not Equal To 0?(x=w887) -> (x != 0?=w888:bool)
                n416 = case shown="True" w888 {
                  tunnel: w889 -> [w891 w903]
                  tunnel: w887 -> [_ w897]
                  frame False {
                    n417 = property on="Property Node" class="WFChart (strict)"(reference=w891) -> (reference out=w890:refnum<vi>, "XScale.Range"=w896:T27)  [unwired: 1 in, 1 out]
                    n418 = Bundle By Name(cluster=w896, "Minimum"=0.0, "Maximum"=3600.0, "Increment"=60.0) -> (w895:T27)
                    n419 = property on="Property Node" class="WFChart (strict)"(reference=w890, "XScale.Range"=w895) -> ()  [unwired: 1 in, 2 out]
                  }
                  frame True {
                    n420 = property on="Property Node" class="WFChart (strict)"(reference=w903) -> (reference out=w900:refnum<vi>, "XScale.Range"=w905:T27)  [unwired: 1 in, 1 out]
                    n421 = Multiply(x=w897, y=60.0) -> (x*y=w899:dbl)
                    n422 = Bundle By Name(cluster=w905, "Minimum"=0.0, "Maximum"=w899, "Increment"=1.0) -> (w904:T27)
                    n423 = property on="Property Node" class="WFChart (strict)"(reference=w900, "XScale.Range"=w904) -> ()  [unwired: 1 in, 2 out]
                  }
                }
              }
              frame 1 {
                n424 = Not Equal To 0?(x=w906) -> (x != 0?=w907:bool)
                n425 = case shown="True" w907 {
                  tunnel: w908 -> [w910 w920]
                  tunnel: w906 -> [_ w917]
                  frame False {
                    n426 = property on="Property Node" class="WFChart (strict)"(reference=w910) -> (reference out=w909:refnum<vi>, "XScale.Range"=w915:T27)  [unwired: 1 in, 1 out]
                    n427 = Bundle By Name(cluster=w915, "Minimum"=0.0, "Maximum"=43200.0, "Increment"=3600.0) -> (w911:T27)
                    n428 = property on="Property Node" class="WFChart (strict)"(reference=w909, "XScale.Range"=w911) -> ()  [unwired: 1 in, 2 out]
                  }
                  frame True {
                    n429 = Multiply(x=w917, y=3600.0) -> (x*y=w916:dbl)
                    n430 = property on="Property Node" class="WFChart (strict)"(reference=w920) -> (reference out=w919:refnum<vi>, "XScale.Range"=w924:T27)  [unwired: 1 in, 1 out]
                    n431 = Bundle By Name(cluster=w924, "Minimum"=0.0, "Maximum"=w916, "Increment"=3600.0) -> (w921:T27)
                    n432 = property on="Property Node" class="WFChart (strict)"(reference=w919, "XScale.Range"=w921) -> ()  [unwired: 1 in, 2 out]
                  }
                }
              }
              frame 2 {
                n433 = Not Equal To 0?(x=w925) -> (x != 0?=w926:bool)
                n434 = case shown="True" w926 {
                  tunnel: w927 -> [w929 w937]
                  tunnel: w925 -> [_ w935]
                  frame False {
                    n435 = property on="Property Node" class="WFChart (strict)"(reference=w929) -> (reference out=w928:refnum<vi>, "XScale.Range"=w934:T27)  [unwired: 1 in, 1 out]
                    n436 = Bundle By Name(cluster=w934, "Minimum"=0.0, "Maximum"=60.0, "Increment"=1.0) -> (w930:T27)
                    n437 = property on="Property Node" class="WFChart (strict)"(reference=w928, "XScale.Range"=w930) -> ()  [unwired: 1 in, 2 out]
                  }
                  frame True {
                    n438 = property on="Property Node" class="WFChart (strict)"(reference=w937) -> (reference out=w936:refnum<vi>, "XScale.Range"=w941:T27)  [unwired: 1 in, 1 out]
                    n439 = Bundle By Name(cluster=w941, "Minimum"=0.0, "Maximum"=w935, "Increment"=1.0) -> (w938:T27)
                    n440 = property on="Property Node" class="WFChart (strict)"(reference=w936, "XScale.Range"=w938) -> ()  [unwired: 1 in, 2 out]
                  }
                }
              }
            }
          }
          event "Set Time TC Graph 5": Mouse Down {
            n441 = event-data() -> ()  [unwired: 1 in, 8 out]
            n442 = local read "Log/Linear Y-Axis 5"() -> (w943:u16)
            n443 = control-ref of="Custom Chart 5"() -> (w942:refnum<vi>)
            n444 = property on="Property Node" class="WFChart (strict)"(reference=w942, "YScale.Mapping Mode"=w943) -> ()  [unwired: 1 in, 2 out]
            n445 = local read "Total Time 5"() -> (w944:dbl)
            n446 = local read "Time Scale 5"() -> (w945:u16)
            n447 = case shown="2" w945 {
              tunnel: w942 -> [w950 w969 w988]
              tunnel: w944 -> [w948 w967 w986]
              frame 0, Default {
                n448 = Not Equal To 0?(x=w948) -> (x != 0?=w949:bool)
                n449 = case shown="True" w949 {
                  tunnel: w950 -> [w952 w964]
                  tunnel: w948 -> [_ w958]
                  frame False {
                    n450 = property on="Property Node" class="WFChart (strict)"(reference=w952) -> (reference out=w951:refnum<vi>, "XScale.Range"=w957:T27)  [unwired: 1 in, 1 out]
                    n451 = Bundle By Name(cluster=w957, "Minimum"=0.0, "Maximum"=3600.0, "Increment"=60.0) -> (w956:T27)
                    n452 = property on="Property Node" class="WFChart (strict)"(reference=w951, "XScale.Range"=w956) -> ()  [unwired: 1 in, 2 out]
                  }
                  frame True {
                    n453 = property on="Property Node" class="WFChart (strict)"(reference=w964) -> (reference out=w961:refnum<vi>, "XScale.Range"=w966:T27)  [unwired: 1 in, 1 out]
                    n454 = Multiply(x=w958, y=60.0) -> (x*y=w960:dbl)
                    n455 = Bundle By Name(cluster=w966, "Minimum"=0.0, "Maximum"=w960, "Increment"=1.0) -> (w965:T27)
                    n456 = property on="Property Node" class="WFChart (strict)"(reference=w961, "XScale.Range"=w965) -> ()  [unwired: 1 in, 2 out]
                  }
                }
              }
              frame 1 {
                n457 = Not Equal To 0?(x=w967) -> (x != 0?=w968:bool)
                n458 = case shown="True" w968 {
                  tunnel: w969 -> [w971 w981]
                  tunnel: w967 -> [_ w978]
                  frame False {
                    n459 = property on="Property Node" class="WFChart (strict)"(reference=w971) -> (reference out=w970:refnum<vi>, "XScale.Range"=w976:T27)  [unwired: 1 in, 1 out]
                    n460 = Bundle By Name(cluster=w976, "Minimum"=0.0, "Maximum"=43200.0, "Increment"=3600.0) -> (w972:T27)
                    n461 = property on="Property Node" class="WFChart (strict)"(reference=w970, "XScale.Range"=w972) -> ()  [unwired: 1 in, 2 out]
                  }
                  frame True {
                    n462 = Multiply(x=w978, y=3600.0) -> (x*y=w977:dbl)
                    n463 = property on="Property Node" class="WFChart (strict)"(reference=w981) -> (reference out=w980:refnum<vi>, "XScale.Range"=w985:T27)  [unwired: 1 in, 1 out]
                    n464 = Bundle By Name(cluster=w985, "Minimum"=0.0, "Maximum"=w977, "Increment"=3600.0) -> (w982:T27)
                    n465 = property on="Property Node" class="WFChart (strict)"(reference=w980, "XScale.Range"=w982) -> ()  [unwired: 1 in, 2 out]
                  }
                }
              }
              frame 2 {
                n466 = Not Equal To 0?(x=w986) -> (x != 0?=w987:bool)
                n467 = case shown="True" w987 {
                  tunnel: w988 -> [w990 w998]
                  tunnel: w986 -> [_ w996]
                  frame False {
                    n468 = property on="Property Node" class="WFChart (strict)"(reference=w990) -> (reference out=w989:refnum<vi>, "XScale.Range"=w995:T27)  [unwired: 1 in, 1 out]
                    n469 = Bundle By Name(cluster=w995, "Minimum"=0.0, "Maximum"=60.0, "Increment"=1.0) -> (w991:T27)
                    n470 = property on="Property Node" class="WFChart (strict)"(reference=w989, "XScale.Range"=w991) -> ()  [unwired: 1 in, 2 out]
                  }
                  frame True {
                    n471 = property on="Property Node" class="WFChart (strict)"(reference=w998) -> (reference out=w997:refnum<vi>, "XScale.Range"=w1002:T27)  [unwired: 1 in, 1 out]
                    n472 = Bundle By Name(cluster=w1002, "Minimum"=0.0, "Maximum"=w996, "Increment"=1.0) -> (w999:T27)
                    n473 = property on="Property Node" class="WFChart (strict)"(reference=w997, "XScale.Range"=w999) -> ()  [unwired: 1 in, 2 out]
                  }
                }
              }
            }
          }
          event "Set Time TC Graph 6": Mouse Down {
            n474 = event-data() -> ()  [unwired: 1 in, 8 out]
            n475 = local read "Log/Linear Y-Axis 6"() -> (w1004:u16)
            n476 = control-ref of="Custom Chart 6"() -> (w1003:refnum<vi>)
            n477 = property on="Property Node" class="WFChart (strict)"(reference=w1003, "YScale.Mapping Mode"=w1004) -> ()  [unwired: 1 in, 2 out]
            n478 = local read "Total Time 6"() -> (w1005:dbl)
            n479 = local read "Time Scale 6"() -> (w1006:u16)
            n480 = case shown="2" w1006 {
              tunnel: w1003 -> [w1011 w1030 w1049]
              tunnel: w1005 -> [w1009 w1028 w1047]
              frame 0, Default {
                n481 = Not Equal To 0?(x=w1009) -> (x != 0?=w1010:bool)
                n482 = case shown="True" w1010 {
                  tunnel: w1011 -> [w1013 w1025]
                  tunnel: w1009 -> [_ w1019]
                  frame False {
                    n483 = property on="Property Node" class="WFChart (strict)"(reference=w1013) -> (reference out=w1012:refnum<vi>, "XScale.Range"=w1018:T27)  [unwired: 1 in, 1 out]
                    n484 = Bundle By Name(cluster=w1018, "Minimum"=0.0, "Maximum"=3600.0, "Increment"=60.0) -> (w1017:T27)
                    n485 = property on="Property Node" class="WFChart (strict)"(reference=w1012, "XScale.Range"=w1017) -> ()  [unwired: 1 in, 2 out]
                  }
                  frame True {
                    n486 = property on="Property Node" class="WFChart (strict)"(reference=w1025) -> (reference out=w1022:refnum<vi>, "XScale.Range"=w1027:T27)  [unwired: 1 in, 1 out]
                    n487 = Multiply(x=w1019, y=60.0) -> (x*y=w1021:dbl)
                    n488 = Bundle By Name(cluster=w1027, "Minimum"=0.0, "Maximum"=w1021, "Increment"=1.0) -> (w1026:T27)
                    n489 = property on="Property Node" class="WFChart (strict)"(reference=w1022, "XScale.Range"=w1026) -> ()  [unwired: 1 in, 2 out]
                  }
                }
              }
              frame 1 {
                n490 = Not Equal To 0?(x=w1028) -> (x != 0?=w1029:bool)
                n491 = case shown="True" w1029 {
                  tunnel: w1030 -> [w1032 w1042]
                  tunnel: w1028 -> [_ w1039]
                  frame False {
                    n492 = property on="Property Node" class="WFChart (strict)"(reference=w1032) -> (reference out=w1031:refnum<vi>, "XScale.Range"=w1037:T27)  [unwired: 1 in, 1 out]
                    n493 = Bundle By Name(cluster=w1037, "Minimum"=0.0, "Maximum"=43200.0, "Increment"=3600.0) -> (w1033:T27)
                    n494 = property on="Property Node" class="WFChart (strict)"(reference=w1031, "XScale.Range"=w1033) -> ()  [unwired: 1 in, 2 out]
                  }
                  frame True {
                    n495 = Multiply(x=w1039, y=3600.0) -> (x*y=w1038:dbl)
                    n496 = property on="Property Node" class="WFChart (strict)"(reference=w1042) -> (reference out=w1041:refnum<vi>, "XScale.Range"=w1046:T27)  [unwired: 1 in, 1 out]
                    n497 = Bundle By Name(cluster=w1046, "Minimum"=0.0, "Maximum"=w1038, "Increment"=3600.0) -> (w1043:T27)
                    n498 = property on="Property Node" class="WFChart (strict)"(reference=w1041, "XScale.Range"=w1043) -> ()  [unwired: 1 in, 2 out]
                  }
                }
              }
              frame 2 {
                n499 = Not Equal To 0?(x=w1047) -> (x != 0?=w1048:bool)
                n500 = case shown="True" w1048 {
                  tunnel: w1049 -> [w1051 w1059]
                  tunnel: w1047 -> [_ w1057]
                  frame False {
                    n501 = property on="Property Node" class="WFChart (strict)"(reference=w1051) -> (reference out=w1050:refnum<vi>, "XScale.Range"=w1056:T27)  [unwired: 1 in, 1 out]
                    n502 = Bundle By Name(cluster=w1056, "Minimum"=0.0, "Maximum"=60.0, "Increment"=1.0) -> (w1052:T27)
                    n503 = property on="Property Node" class="WFChart (strict)"(reference=w1050, "XScale.Range"=w1052) -> ()  [unwired: 1 in, 2 out]
                  }
                  frame True {
                    n504 = property on="Property Node" class="WFChart (strict)"(reference=w1059) -> (reference out=w1058:refnum<vi>, "XScale.Range"=w1063:T27)  [unwired: 1 in, 1 out]
                    n505 = Bundle By Name(cluster=w1063, "Minimum"=0.0, "Maximum"=w1057, "Increment"=1.0) -> (w1060:T27)
                    n506 = property on="Property Node" class="WFChart (strict)"(reference=w1058, "XScale.Range"=w1060) -> ()  [unwired: 1 in, 2 out]
                  }
                }
              }
            }
          }
          event "1. Compile Profile": Mouse Down {
            n507 = event-data() -> ()  [unwired: 1 in, 1 out]
            n508 = control-ref of="Number of Set points"() -> (w1071:refnum<vi>)
            n509 = property class="DigNum (strict)"(reference=w1071) -> ("Value"=w1068:dbl)  [unwired: 1 in, 2 out]
            n510 = Bundle By Name(cluster=w1070, "ZoneSetup.Number of Set points"=w1068) -> (w1069:T13)
            n511 = local write "ThermalProfileStatus"("Compiling..........." ("String")) -> ()
            n512 = call-poly "Send Message.vi"("error in (no error)"=w1073, "event"="compileProfile") -> ("error out"=w1065:errorcluster)  [unwired: 9 in]
            n513 = call-poly "Send Message.vi"("error in (no error)"=w1065, "event"="compileProfile") -> ("error out"=w1064:errorcluster)  [unwired: 9 in]
          }
          event "2. Save Into Database": Mouse Down {
            n514 = event-data() -> ()  [unwired: 1 in, 1 out]
            n515 = Unbundle By Name(w1075) -> ("Http session"=w1094:T12, "URL prefex"=w1090:string, "ZoneProfile.profiles"=w1089:T28, "ZoneSetup.Thermal Profile Name"=w1079:string)
            n516 = Empty String/Path?(string/path=w1079) -> (empty?=w1080:bool)
            n517 = case shown="True" w1080 {
              tunnel: w1079 -> [w1097 _]
              tunnel: [w1097 w1098] -> w1078
              tunnel: w1077 -> [w1096 w1102]
              tunnel: [w1096 w1101] -> w1076
              tunnel: w1075 -> [w1095 w1100]
              tunnel: [w1095 w1099] -> w1074
              frame False {
              }
              frame True {
                n518 = call "Prompt User for Input"("error in (no error)"=w1102) -> ("Profile Name"=w1098:string, "error out"=w1101:errorcluster)  [unwired: 16 in, 1 out]
                n519 = Bundle By Name(cluster=w1100, "ZoneSetup.Thermal Profile Name"=w1098) -> (w1099:T13)
              }
            }
            n520 = Bundle By Name(cluster=T15 {"name"="", "profiles"=[]}, "name"=w1078, "profiles"=w1089) -> (w1087:T15)
            n521 = Concatenate Strings(w1090, "saveProfile" ("url")) -> (w1093:string)
            n522 = Flatten To JSON(anything=w1087) -> (JSON string=w1092:string)  [unwired: 2 in, 1 out]
            n523 = call-poly <vilib>:"POST.vi"("client handle"=w1094, "url"=w1093, "buffer"=w1092) -> ("client handle out"=w1085:T12, "body"=w1081:string)  [unwired: 9 in, 2 out]
            n524 = Match True/False String(2:"" ("false string"), 3:"{'result':'success'}" ("true string"), 4:w1081) -> (0:w1082:bool)  [unwired: 1 out]
            n525 = Bundle By Name(cluster=w1074, "Http session"=w1085) -> (w1086:T13)
            n526 = case shown="True" w1082 {
              tunnel: w1081 -> [w1104 _]
              frame False {
                n527 = Concatenate Strings("Error While Saving : " ("string"), w1104) -> (w1103:string)
                n528 = One Button Dialog(message=w1103) -> ()  [unwired: 1 in, 1 out]
              }
              frame True {
                n529 = One Button Dialog(message="Profile Saved To Database Successfully") -> ()  [unwired: 1 in, 1 out]
              }
            }
          }
          event "3. Load into Memory": Mouse Down {
            n530 = event-data() -> ()  [unwired: 1 in, 1 out]
            n531 = Unbundle By Name(w1113) -> ("Http session"=w1114:T12, "URL prefex"=w1121:string, "ZoneSetup.Thermal Profile Name"=w1117:string)  [unwired: 1 out]
            n532 = Bundle By Name(cluster=cluster{"profile_name":string} {"profile_name"=""}, "profile_name"=w1117) -> (w1116:cluster{"profile_name":string})
            n533 = Flatten To JSON(anything=w1116) -> (JSON string=w1115:string)  [unwired: 2 in, 1 out]
            n534 = Concatenate Strings(w1121, "loadProfile" ("url")) -> (w1119:string)
            n535 = call-poly <vilib>:"POST.vi"("client handle"=w1114, "url"=w1119, "buffer"=w1115) -> ("client handle out"=w1111:T12, "body"=w1107:string)  [unwired: 9 in, 2 out]
            n536 = Match True/False String(2:"" ("false string"), 3:"{'result':'success'}" ("true string"), 4:w1107) -> (0:w1108:bool)  [unwired: 1 out]
            n537 = case shown="True" w1108 {
              tunnel: w1107 -> [w1124 _]
              frame False {
                n538 = Concatenate Strings("Error While Loading : " ("string"), w1124) -> (w1123:string)
                n539 = One Button Dialog(message=w1123) -> ()  [unwired: 1 in, 1 out]
              }
              frame True {
                n540 = One Button Dialog(message="Profile Loaded into Memory Successfully") -> ()  [unwired: 1 in, 1 out]
              }
            }
            n541 = Bundle By Name(cluster=w1113, "Http session"=w1111) -> (w1112:T13)
          }
          event "4. Run Profile": Mouse Down {
            n542 = event-data() -> ()  [unwired: 1 in, 1 out]
            n543 = Unbundle By Name(w1133) -> ("Http session"=w1134:T12, "URL prefex"=w1135:string)
            n544 = Concatenate Strings(w1135, "runProfile" ("url")) -> (w1136:string)
            n545 = call <vilib>:"GET.vi"("client handle"=w1134, "url"=w1136) -> ("client handle out"=w1131:T12, "body"=w1127:string)  [unwired: 10 in, 2 out]
            n546 = Match True/False String(2:"" ("false string"), 3:"{'result':'success'}" ("true string"), 4:w1127) -> (0:w1128:bool)  [unwired: 1 out]
            n547 = case shown="True" w1128 {
              tunnel: w1127 -> [w1140 _]
              frame False {
                n548 = Concatenate Strings("Error While Starting : " ("string"), w1140) -> (w1139:string)
                n549 = One Button Dialog(message=w1139) -> ()  [unwired: 1 in, 1 out]
              }
              frame True {
                n550 = One Button Dialog(message="Success: Profile is Running") -> ()  [unwired: 1 in, 1 out]
              }
            }
            n551 = Bundle By Name(cluster=w1133, "Http session"=w1131) -> (w1132:T13)
          }
          event "Rename": Mouse Down {
            n552 = event-data() -> ()  [unwired: 1 in, 1 out]
            n553 = Unbundle By Name(w1145) -> ()  [unwired: 1 out]
            n554 = Bundle By Name(cluster=w1145, "ZoneSetup.Thermal Profile Name"="New Name") -> (w1144:T13)
          }
          event "Hold Profile": Mouse Down {
            n555 = event-data() -> ()  [unwired: 1 in, 1 out]
            n556 = Unbundle By Name(w1152) -> ("URL prefex"=w1150:string)  [unwired: 1 out]
            n557 = Concatenate Strings(w1150, "hold" ("url")) -> (w1149:string)
            n558 = call <vilib>:"GET.vi"("url"=w1149, "error in (no error)"=w1148) -> ("error out"=w1147:errorcluster)  [unwired: 10 in, 3 out]
          }
          event "Pause Profile": Mouse Down {
            n559 = event-data() -> ()  [unwired: 1 in, 1 out]
            n560 = Unbundle By Name(w1158) -> ("URL prefex"=w1156:string)  [unwired: 1 out]
            n561 = Concatenate Strings(w1156, "pause" ("url")) -> (w1155:string)
            n562 = call <vilib>:"GET.vi"("url"=w1155, "error in (no error)"=w1154) -> ("error out"=w1153:errorcluster)  [unwired: 10 in, 3 out]
          }
          event "Resume Profile": Mouse Down {
            n563 = event-data() -> ()  [unwired: 1 in, 1 out]
            n564 = Unbundle By Name(w1164) -> ("URL prefex"=w1162:string)  [unwired: 1 out]
            n565 = Concatenate Strings(w1162, "resume" ("url")) -> (w1161:string)
            n566 = call <vilib>:"GET.vi"("url"=w1161, "error in (no error)"=w1160) -> ("error out"=w1159:errorcluster)  [unwired: 10 in, 3 out]
          }
          event "Stop Profile": Mouse Down {
            n567 = event-data() -> ()  [unwired: 1 in, 1 out]
            n568 = Unbundle By Name(w1170) -> ("URL prefex"=w1168:string)  [unwired: 1 out]
            n569 = Concatenate Strings(w1168, "hardStop" ("url")) -> (w1167:string)
            n570 = call <vilib>:"GET.vi"("url"=w1167, "error in (no error)"=w1166) -> ("error out"=w1165:errorcluster)  [unwired: 10 in, 3 out]
          }
          event "Save as CSV": Mouse Down {
            n571 = event-data() -> ()  [unwired: 1 in, 1 out]
            n572 = call-poly "Send Message.vi"("error in (no error)"=w1172, "event"="saveProfile") -> ("error out"=w1171:errorcluster)  [unwired: 9 in]
          }
          event "Import Profile": Value Change {
            w1194 = TRUE ("Page Visible")
            n573 = event-data() -> ("CtlRef"=w1180:refnum<vi>, "OldVal"=w1181:bool)  [unwired: 1 in, 4 out]
            n574 = local read "Path"() -> (w1186:path)
            n575 = control-ref of="CreateTProfile"() -> (w1204:refnum<vi>)
            n576 = control-ref of="Zone Selection"() -> (w1203:refnum<vi>)
            n577 = property on="Property Node" class="TabCtl (strict)"(reference=w1204) -> ("Pages"=w1197:refnum<vi>[])  [unwired: 1 in, 2 out]
            n578 = property class="Bool (strict)"(reference=w1180, "Value"=w1181) -> ()  [unwired: 1 in, 2 out]
            n579 = property on="Property Node" class="LstBox (strict)"(reference=w1203) -> ("Item Symbols"=w1202:i32[])  [unwired: 1 in, 2 out]
            n580 = call-poly <vilib>:"Read Delimited Spreadsheet.vi"("file path (dialog if empty)"=w1186, "delimiter (\\t)"="," ("delimiter (\\t)")) -> ("all rows"=w1187:string[][])  [unwired: 8 in, 5 out]
            n581 = Array Size(array=w1187) -> (size(s)=w1192:i32[])
            n582 = Index Array(array=w1192, index=0) -> (element=w1190:i32)
            n583 = Subtract(x=w1190, y=7) -> (x-y=w1188:i32)
            n584 = To Double Precision Float(number=w1188) -> (double precision float=w1185:dbl)
            n585 = Unbundle By Name(w1179) -> ("ZonesSelected"=w1176:bool[])
            n586 = for {
              N: 13 -> [_]
              tunnel: w1202 -> [w1239]
              tunnel: w1197 -> [w1240] mode=indexing
              shift-right: [w1232] -> w1177
              shift-left: w1176 -> [w1231]
              i -> [w1234]
              n587 = Greater?(x=w1234, y=1) -> (0:w1236:bool)
              n588 = Less?(x=w1234, y=11 ("x")) -> (x < y?=w1237:bool)
              n589 = And(x=w1237, y=w1236) -> (x .and. y?=w1235:bool)
              n590 = case shown="True" w1235 {
                tunnel: w1240 -> [_ w1251]
                tunnel: w1239 -> [_ w1248]
                tunnel: w1234 -> [_ w1247]
                tunnel: w1231 -> [w1241 w1244]
                tunnel: [w1241 w1242] -> w1232
                frame False {
                }
                frame True {
                  n591 = Subtract(x=w1247, y=2) -> (x-y=w1243:i32)
                  n592 = Index Array(array=w1248, index=w1243) -> (element=w1245:i32)
                  n593 = Equal?(x=38, y=w1245) -> (x = y?=w1249:bool)
                  n594 = case shown="False" w1249 {
                    tunnel: w1251 -> [w1256 w1261]
                    tunnel: w1244 -> [w1255 w1260]
                    tunnel: w1243 -> [w1253 w1259]
                    tunnel: [w1254 w1257] -> w1242
                    frame False {
                      w1252 = FALSE ("Page Visible")
                      n595 = property class="Page"(reference=w1256, "Page Visible"=w1252) -> ()  [unwired: 1 in, 2 out]
                      n596 = Replace Array Subset(array=w1255, new element=w1252, index=w1253) -> (w1254:bool[])
                    }
                    frame True {
                      w1258 = TRUE ("Page Visible")
                      n597 = property class="Page"(reference=w1261, "Page Visible"=w1258) -> ()  [unwired: 1 in, 2 out]
                      n598 = Replace Array Subset(array=w1260, new element=w1258, index=w1259) -> (w1257:bool[])
                    }
                  }
                }
              }
            }
            n599 = local write "ThermalProfileStatus"("Compiling..........." ("String")) -> ()
            n600 = Bundle By Name(cluster=w1179, "ZonesSelected"=w1177) -> (w1178:T13)
            n601 = Index Array(array=w1197, index #1=11 ("index"), index #2=1 ("index")) -> (element #1=w1199:refnum<vi>, element #2=w1195:refnum<vi>)
            n602 = property class="Page"(reference=w1199, "Page Visible"=w1194) -> ()  [unwired: 1 in, 2 out]
            n603 = property class="Page"(reference=w1195, "Page Visible"=w1194) -> ()  [unwired: 1 in, 2 out]
            n604 = for {
              N: 9 -> [_]
              tunnel: w1185 -> [w1210]
              n605 = Initialize Array(0, w1210, 2 ("dimension size")) -> (w1209:i32[][])
              n606 = Initialize Array(0, w1210, 3 ("dimension size")) -> (w1215:i32[][])
              n607 = for {
                N: w1210 -> [_]
                shift-right: [w1229] -> w1206
                shift-left: w1215 -> [w1230]
                shift-right: [w1220] -> w1208
                shift-left: w1209 -> [w1221]
                i -> [w1218]
                w1222 = 0 ("disabled index (col)")
                w1224 = 0 ("disabled index (col)")
                n608 = Increment(x=w1218) -> (x+1=w1223:i32)
                n609 = Increment(x=w1218) -> (x+1=w1225:i32)
                n610 = Replace Array Subset(array=i32[][] [[0]], new element=w1223, index (row)=w1222, index (col)=w1222) -> (w1216:i32[][])
                n611 = Replace Array Subset(array=i32[][] [[0, 0, 0]], new element=w1225, index (row)=w1224, index (col)=w1224) -> (w1228:i32[][])
                n612 = Index Array(array=w1216, index (row)=w1222) -> (element=w1219:i32[])  [unwired: 1 in]
                n613 = Index Array(array=w1228, index (row)=w1224) -> (element=w1227:i32[])  [unwired: 1 in]
                n614 = Replace Array Subset(array=w1221, new element=w1219, index (row)=w1218) -> (w1220:i32[][])  [unwired: 1 in]
                n615 = Replace Array Subset(array=w1230, new element=w1227, index (row)=w1218) -> (w1229:i32[][])  [unwired: 1 in]
              }
              n616 = Number To Decimal String(number=w1208) -> ()  [unwired: 1 in, 1 out]
              n617 = To Double Precision Float(number=w1206) -> (double precision float=w1205:dbl[][])
              n618 = control-ref of="RampSoakTimes"() -> (w1207:refnum<vi>)
              n619 = property class="Arr (strict)"(reference=w1207, "Value"=w1205) -> ()  [unwired: 1 in, 2 out]
            }
            n620 = call-poly "Send Message.vi"("error in (no error)"=w1184, "event"="importProfile") -> ("error out"=w1183:errorcluster)  [unwired: 9 in]
          }
          event "Current Errors (click to clear)": Mouse Down {
            n621 = event-data() -> ("CtlRef"=w1269:refnum<vi>, "Coords"=w1268:T26)  [unwired: 1 in]
            n622 = invoke on="Invoke Node" class="MCListbox (strict)" method="Point To Row Column"(reference=w1269, "Point"=w1268) -> (reference out=w1265:refnum<vi>, "InBounds"=w1262:bool, "CellPosition"=w1266:T29)  [unwired: 5 in, 4 out]
            n623 = case shown="True" w1262 {
              tunnel: w1266 -> [_ w1282]
              tunnel: w1265 -> [_ w1281]
              tunnel: w1264 -> [w1270 w1280]
              tunnel: [w1270 w1279] -> w1263
              frame False {
              }
              frame True {
                n624 = Unbundle By Name(w1282) -> ("Row"=w1275:i32)
                n625 = property on="Property Node" class="MCListbox (strict)"(reference=w1281, "ActiveCell"=w1282) -> (reference out=w1277:refnum<vi>)  [unwired: 1 in, 1 out]
                n626 = Unbundle By Name(w1280) -> ("ErrorArray"=w1276:string[][], "PrevErrorArray"=w1278:string[][])
                n627 = Index Array(array=w1276, index (row)=w1275, index (col)=1 ("disabled index (col)")) -> (element=w1271:string)
                n628 = Equal?(x=w1271, y="") -> (x = y?=w1273:bool)
                n629 = case shown="False" w1273 {
                  tunnel: w1280 -> [w1292 w1293]
                  tunnel: [w1291 w1293] -> w1279
                  tunnel: w1278 -> [w1290 _]
                  tunnel: w1277 -> [w1288 _]
                  tunnel: w1276 -> [w1284 _]
                  tunnel: w1275 -> [w1283 _]
                  frame False {
                    n630 = control-ref of="Error History"() -> (w1287:refnum<vi>)
                    n631 = Delete From Array(array=w1284, index (row)=w1283) -> (deleted portion=w1289:string[], array with subset deleted=w1285:string[][])  [unwired: 2 in]
                    n632 = Build Array (concatenate)(w1289, w1290) -> (w1286:string[][])
                    n633 = property on="Property Node" class="MCListbox (strict)"(reference=w1288, "ItemNames"=w1285) -> ()  [unwired: 1 in, 2 out]
                    n634 = property on="Property Node" class="MCListbox (strict)"(reference=w1287, "ItemNames"=w1286) -> ()  [unwired: 1 in, 2 out]
                    n635 = Bundle By Name(cluster=w1292, "ErrorArray"=w1285, "PrevErrorArray"=w1286) -> (w1291:T13)
                  }
                  frame True {
                  }
                }
              }
            }
          }
          event "Current Events (click to clear)": Mouse Down {
            n636 = event-data() -> ("CtlRef"=w1301:refnum<vi>, "Coords"=w1300:T26)  [unwired: 1 in]
            n637 = invoke on="Invoke Node" class="MCListbox (strict)" method="Point To Row Column"(reference=w1301, "Point"=w1300) -> (reference out=w1297:refnum<vi>, "InBounds"=w1294:bool, "CellPosition"=w1298:T29)  [unwired: 5 in, 4 out]
            n638 = case shown="True" w1294 {
              tunnel: w1298 -> [_ w1314]
              tunnel: w1297 -> [_ w1313]
              tunnel: w1296 -> [w1302 w1312]
              tunnel: [w1302 w1311] -> w1295
              frame False {
              }
              frame True {
                n639 = Unbundle By Name(w1314) -> ("Row"=w1307:i32)
                n640 = property on="Property Node" class="MCListbox (strict)"(reference=w1313, "ActiveCell"=w1314) -> (reference out=w1309:refnum<vi>)  [unwired: 1 in, 1 out]
                n641 = Unbundle By Name(w1312) -> ("EventArray"=w1308:string[][], "PrevEventArray"=w1310:string[][])
                n642 = Index Array(array=w1308, index (row)=w1307, index (col)=1 ("disabled index (col)")) -> (element=w1303:string)
                n643 = Equal?(x=w1303, y="") -> (x = y?=w1305:bool)
                n644 = case shown="False" w1305 {
                  tunnel: w1312 -> [w1324 w1325]
                  tunnel: [w1323 w1325] -> w1311
                  tunnel: w1310 -> [w1322 _]
                  tunnel: w1309 -> [w1320 _]
                  tunnel: w1308 -> [w1316 _]
                  tunnel: w1307 -> [w1315 _]
                  frame False {
                    n645 = control-ref of="Event History"() -> (w1319:refnum<vi>)
                    n646 = Delete From Array(array=w1316, index (row)=w1315) -> (deleted portion=w1321:string[], array with subset deleted=w1317:string[][])  [unwired: 2 in]
                    n647 = Build Array (concatenate)(w1321, w1322) -> (w1318:string[][])
                    n648 = property on="Property Node" class="MCListbox (strict)"(reference=w1320, "ItemNames"=w1317) -> ()  [unwired: 1 in, 2 out]
                    n649 = property on="Property Node" class="MCListbox (strict)"(reference=w1319, "ItemNames"=w1318) -> ()  [unwired: 1 in, 2 out]
                    n650 = Bundle By Name(cluster=w1324, "EventArray"=w1317, "PrevEventArray"=w1318) -> (w1323:T13)
                  }
                  frame True {
                  }
                }
              }
            }
          }
          event "Clear All Errors": Mouse Down {
            w1330 = 0 ("index")
            n651 = event-data() -> ()  [unwired: 1 in, 5 out]
            n652 = Unbundle By Name(w1343) -> ("ErrorArray"=w1329:string[][], "PrevErrorArray"=w1341:string[][])
            n653 = Array Size(array=w1329) -> (size(s)=w1339:i32[])
            n654 = Index Array(array=w1339, index #1=w1330, index #2=1 ("index")) -> (element #1=w1337:i32)  [unwired: 1 out]
            n655 = Index Array(array=w1329, index (col)=1 ("disabled index (col)")) -> (element=w1332:string[])  [unwired: 1 in]
            n656 = Array Size(array=w1329) -> (size(s)=w1328:i32[])
            n657 = Initialize Array(0, w1337) -> (w1335:i32[])
            n658 = Index Array(array=w1332, index=w1330) -> (element=w1331:string)
            n659 = Index Array(array=w1328, index=0) -> (element=w1326:i32)
            n660 = Not Equal?(x=w1331, y="") -> (x != y?=w1334:bool)
            n661 = case shown="True" w1334 {
              tunnel: w1343 -> [w1345 w1356]
              tunnel: [w1345 w1355] -> w1342
              tunnel: w1341 -> [_ w1354]
              tunnel: w1329 -> [_ w1350]
              tunnel: w1335 -> [_ w1353]
              tunnel: w1326 -> [_ w1347]
              frame False {
              }
              frame True {
                w1346 = string[][] [] ("Item Names")
                n662 = for {
                  N: w1347 -> [_]
                  shift-right: [w1362] -> w1348
                  shift-left: w1354 -> [w1363]
                  shift-right: [w1361] -> w1351
                  shift-left: w1353 -> [w1361]
                  tunnel: w1350 -> [w1357] mode=indexing
                  n663 = Index Array(array=w1357, index=1) -> (element=w1358:string)
                  n664 = Empty String/Path?(string/path=w1358) -> (empty?=w1360:bool)
                  n665 = case shown="False" w1360 {
                    tunnel: w1363 -> [w1366 w1367]
                    tunnel: [w1365 w1367] -> w1362
                    tunnel: w1357 -> [w1364 _]
                    frame False {
                      n666 = Build Array (concatenate)(w1364, w1366) -> (w1365:string[][])
                    }
                    frame True {
                    }
                  }
                }
                n667 = Bundle By Name(cluster=w1356, "ErrorArray"=w1346, "PrevErrorArray"=w1348) -> (w1355:T13)
                n668 = control-ref of="Current Errors (click to clear)"() -> (w1352:refnum<vi>)
                n669 = property on="Property Node" class="MCListbox (strict)"(reference=w1352, "ItemNames"=w1346) -> ()  [unwired: 1 in, 2 out]
                n670 = property on="Property Node" class="MCListbox (strict)"(reference=w1352, "ItemSyms"=w1351) -> ()  [unwired: 1 in, 2 out]
                n671 = control-ref of="Error History"() -> (w1349:refnum<vi>)
                n672 = property on="Property Node" class="MCListbox (strict)"(reference=w1349, "ItemNames"=w1348) -> ()  [unwired: 1 in, 2 out]
              }
            }
          }
          event "Clear All Events": Mouse Down {
            w1372 = 0 ("index")
            n673 = event-data() -> ()  [unwired: 1 in, 5 out]
            n674 = Unbundle By Name(w1385) -> ("EventArray"=w1371:string[][], "PrevEventArray"=w1383:string[][])
            n675 = Array Size(array=w1371) -> (size(s)=w1381:i32[])
            n676 = Index Array(array=w1381, index #1=w1372, index #2=1 ("index")) -> (element #1=w1379:i32)  [unwired: 1 out]
            n677 = Index Array(array=w1371, index (col)=1 ("disabled index (col)")) -> (element=w1374:string[])  [unwired: 1 in]
            n678 = Array Size(array=w1371) -> (size(s)=w1370:i32[])
            n679 = Initialize Array(0, w1379) -> (w1377:i32[])
            n680 = Index Array(array=w1374, index=w1372) -> (element=w1373:string)
            n681 = Index Array(array=w1370, index=0) -> (element=w1368:i32)
            n682 = Not Equal?(x=w1373, y="") -> (x != y?=w1376:bool)
            n683 = case shown="True" w1376 {
              tunnel: w1385 -> [w1387 w1398]
              tunnel: [w1387 w1397] -> w1384
              tunnel: w1383 -> [_ w1396]
              tunnel: w1371 -> [_ w1392]
              tunnel: w1377 -> [_ w1395]
              tunnel: w1368 -> [_ w1389]
              frame False {
              }
              frame True {
                w1388 = string[][] [] ("Item Names")
                n684 = for {
                  N: w1389 -> [_]
                  shift-right: [w1404] -> w1390
                  shift-left: w1396 -> [w1405]
                  shift-right: [w1403] -> w1393
                  shift-left: w1395 -> [w1403]
                  tunnel: w1392 -> [w1399] mode=indexing
                  n685 = Index Array(array=w1399, index=1) -> (element=w1400:string)
                  n686 = Empty String/Path?(string/path=w1400) -> (empty?=w1402:bool)
                  n687 = case shown="False" w1402 {
                    tunnel: w1405 -> [w1408 w1409]
                    tunnel: [w1407 w1409] -> w1404
                    tunnel: w1399 -> [w1406 _]
                    frame False {
                      n688 = Build Array (concatenate)(w1406, w1408) -> (w1407:string[][])
                    }
                    frame True {
                    }
                  }
                }
                n689 = Bundle By Name(cluster=w1398, "EventArray"=w1388, "PrevEventArray"=w1390) -> (w1397:T13)
                n690 = control-ref of="Current Events (click to clear)"() -> (w1394:refnum<vi>)
                n691 = property on="Property Node" class="MCListbox (strict)"(reference=w1394, "ItemNames"=w1388) -> ()  [unwired: 1 in, 2 out]
                n692 = property on="Property Node" class="MCListbox (strict)"(reference=w1394, "ItemSyms"=w1393) -> ()  [unwired: 1 in, 2 out]
                n693 = control-ref of="Event History"() -> (w1391:refnum<vi>)
                n694 = property on="Property Node" class="MCListbox (strict)"(reference=w1391, "ItemNames"=w1390) -> ()  [unwired: 1 in, 2 out]
              }
            }
          }
          event "ZoneSetup.Zone Selection": Mouse Down {
            n695 = event-data() -> ("CtlRef"=w1416:refnum<vi>, "Coords"=w1422:T26)  [unwired: 1 in]
            n696 = Unbundle By Name(w1413) -> ("ZonesSelected"=w1414:bool[])
            n697 = invoke on="Invoke Node" class="LstBox (strict)" method="Point To Row"(reference=w1416, "Point"=w1422) -> ("Row"=w1415:i32)  [unwired: 5 in, 6 out]
            n698 = property on="Property Node" class="LstBox (strict)"(reference=w1416) -> ("Item Symbols"=w1418:i32[])  [unwired: 1 in, 2 out]
            n699 = Index Array(array=w1418, index=w1415) -> (element=w1420:i32)
            n700 = Equal?(x=w1420, y=37) -> (x = y?=w1421:bool)
            n701 = case shown="True" w1421 {
              tunnel: w1418 -> [w1428 w1436]
              tunnel: w1415 -> [w1424 w1433]
              tunnel: [w1427 w1434] -> w1410
              tunnel: w1414 -> [w1426 w1431]
              tunnel: [w1423 w1430] -> w1411
              frame False {
                n702 = Replace Array Subset(array=w1426, new element=FALSE ("Boolean"), index=w1424) -> (w1423:bool[])
                n703 = Replace Array Subset(array=w1428, new element=37, index=w1424) -> (w1427:i32[])
              }
              frame True {
                n704 = Replace Array Subset(array=w1431, new element=TRUE ("Boolean"), index=w1433) -> (w1430:bool[])
                n705 = Replace Array Subset(array=w1436, new element=38, index=w1433) -> (w1434:i32[])
              }
            }
            n706 = Bundle By Name(cluster=w1413, "ZonesSelected"=w1411, "ZoneSetup.Zone Selection"=w1410) -> (w1412:T13)
            n707 = property on="Property Node" class="LstBox (strict)"(reference=w1416, "Item Symbols"=w1410) -> ()  [unwired: 1 in, 2 out]
          }
          event "ZoneSetup.Initiate Setup": Value Change {
            w1440 = TRUE ("Page Visible")
            n708 = event-data() -> ("CtlRef"=w1439:refnum<vi>, "OldVal"=w1438:bool)  [unwired: 1 in, 4 out]
            n709 = control-ref of="CreateTProfile"() -> (w1453:refnum<vi>)
            n710 = property class="Bool (strict)"(reference=w1439, "Value"=w1438) -> ()  [unwired: 1 in, 2 out]
            n711 = control-ref of="Zone Selection"() -> (w1452:refnum<vi>)
            n712 = property on="Property Node" class="TabCtl (strict)"(reference=w1453) -> ("Pages"=w1443:refnum<vi>[])  [unwired: 1 in, 2 out]
            n713 = property on="Property Node" class="LstBox (strict)"(reference=w1452) -> ("Item Symbols"=w1451:i32[])  [unwired: 1 in, 2 out]
            n714 = for {
              N: 13 -> [_]
              tunnel: w1451 -> [w1507]
              tunnel: w1443 -> [w1508] mode=indexing
              i -> [w1502]
              n715 = Greater?(x=w1502, y=1) -> (0:w1504:bool)
              n716 = Less?(x=w1502, y=11 ("x")) -> (x < y?=w1505:bool)
              n717 = And(x=w1505, y=w1504) -> (x .and. y?=w1503:bool)
              n718 = case shown="True" w1503 {
                tunnel: w1508 -> [_ w1516]
                tunnel: w1507 -> [_ w1513]
                tunnel: w1502 -> [_ w1512]
                frame False {
                }
                frame True {
                  n719 = Subtract(x=w1512, y=2) -> (x-y=w1510:i32)
                  n720 = Index Array(array=w1513, index=w1510) -> (element=w1509:i32)
                  n721 = Equal?(x=38, y=w1509) -> (x = y?=w1514:bool)
                  n722 = case shown="True" w1514 {
                    tunnel: w1516 -> [w1517 w1519]
                    frame False {
                      n723 = property class="Page"(reference=w1517, "Page Visible"=FALSE) -> ()  [unwired: 1 in, 2 out]
                    }
                    frame True {
                      n724 = property class="Page"(reference=w1519, "Page Visible"=TRUE) -> ()  [unwired: 1 in, 2 out]
                    }
                  }
                }
              }
            }
            n725 = Index Array(array=w1443, index #1=11 ("index"), index #2=1 ("index")) -> (element #1=w1448:refnum<vi>, element #2=w1441:refnum<vi>)
            n726 = property on="Number of Set points" class="DigNum (strict)"() -> ("NumText.Text"=w1445:string)  [unwired: 2 in, 2 out]
            n727 = property class="Page"(reference=w1448, "Page Visible"=w1440) -> ()  [unwired: 1 in, 2 out]
            n728 = property class="Page"(reference=w1441, "Page Visible"=w1440) -> ()  [unwired: 1 in, 2 out]
            n729 = Decimal String To Number(string=w1445) -> (number=w1437:i32)  [unwired: 2 in, 1 out]
            n730 = for {
              N: 9 -> [_]
              tunnel: w1437 -> [w1460]
              i -> [w1458]
              n731 = Initialize Array(0, w1460, 2 ("dimension size")) -> (w1459:i32[][])
              n732 = Initialize Array(0, w1460, 3 ("dimension size")) -> (w1465:i32[][])
              n733 = for {
                N: w1460 -> [_]
                shift-right: [w1499] -> w1456
                shift-left: w1465 -> [w1500]
                shift-right: [w1490] -> w1455
                shift-left: w1459 -> [w1491]
                i -> [w1488]
                w1492 = 0 ("disabled index (col)")
                w1494 = 0 ("disabled index (col)")
                n734 = Increment(x=w1488) -> (x+1=w1493:i32)
                n735 = Increment(x=w1488) -> (x+1=w1495:i32)
                n736 = Replace Array Subset(array=i32[][] [[0, 0]], new element=w1493, index (row)=w1492, index (col)=w1492) -> (w1486:i32[][])
                n737 = Replace Array Subset(array=i32[][] [[0, 0, 0]], new element=w1495, index (row)=w1494, index (col)=w1494) -> (w1498:i32[][])
                n738 = Index Array(array=w1486, index (row)=w1492) -> (element=w1489:i32[])  [unwired: 1 in]
                n739 = Index Array(array=w1498, index (row)=w1494) -> (element=w1497:i32[])  [unwired: 1 in]
                n740 = Replace Array Subset(array=w1491, new element=w1489, index (row)=w1488) -> (w1490:i32[][])  [unwired: 1 in]
                n741 = Replace Array Subset(array=w1500, new element=w1497, index (row)=w1488) -> (w1499:i32[][])  [unwired: 1 in]
              }
              n742 = To Double Precision Float(number=w1455) -> (double precision float=w1454:dbl[][])
              n743 = To Double Precision Float(number=w1456) -> (double precision float=w1457:dbl[][])
              n744 = case shown="0, Default" w1458 {
                tunnel: w1457 -> [w1467 _ _ _ _ _ _ _ _]
                tunnel: w1454 -> [w1466 w1470 w1472 w1474 w1476 w1478 w1480 w1482 w1484]
                frame 0, Default {
                  n745 = control-ref of="Temperature Goal"() -> (w1469:refnum<vi>)
                  n746 = control-ref of="RampSoakTimes"() -> (w1468:refnum<vi>)
                  n747 = property class="Arr (strict)"(reference=w1469, "Value"=w1466) -> ()  [unwired: 1 in, 2 out]
                  n748 = property class="Arr (strict)"(reference=w1468, "Value"=w1467) -> ()  [unwired: 1 in, 2 out]
                }
                frame 1 {
                  n749 = control-ref of="Temperature Goal"() -> (w1471:refnum<vi>)
                  n750 = property class="Arr (strict)"(reference=w1471, "Value"=w1470) -> ()  [unwired: 1 in, 2 out]
                }
                frame 2 {
                  n751 = control-ref of="Temperature Goal"() -> (w1473:refnum<vi>)
                  n752 = property class="Arr (strict)"(reference=w1473, "Value"=w1472) -> ()  [unwired: 1 in, 2 out]
                }
                frame 3 {
                  n753 = control-ref of="Temperature Goal"() -> (w1475:refnum<vi>)
                  n754 = property class="Arr (strict)"(reference=w1475, "Value"=w1474) -> ()  [unwired: 1 in, 2 out]
                }
                frame 4 {
                  n755 = control-ref of="Temperature Goal"() -> (w1477:refnum<vi>)
                  n756 = property class="Arr (strict)"(reference=w1477, "Value"=w1476) -> ()  [unwired: 1 in, 2 out]
                }
                frame 5 {
                  n757 = control-ref of="Temperature Goal"() -> (w1479:refnum<vi>)
                  n758 = property class="Arr (strict)"(reference=w1479, "Value"=w1478) -> ()  [unwired: 1 in, 2 out]
                }
                frame 6 {
                  n759 = control-ref of="Temperature Goal"() -> (w1481:refnum<vi>)
                  n760 = property class="Arr (strict)"(reference=w1481, "Value"=w1480) -> ()  [unwired: 1 in, 2 out]
                }
                frame 7 {
                  n761 = control-ref of="Temperature Goal"() -> (w1483:refnum<vi>)
                  n762 = property class="Arr (strict)"(reference=w1483, "Value"=w1482) -> ()  [unwired: 1 in, 2 out]
                }
                frame 8 {
                  n763 = control-ref of="Temperature Goal"() -> (w1485:refnum<vi>)
                  n764 = property class="Arr (strict)"(reference=w1485, "Value"=w1484) -> ()  [unwired: 1 in, 2 out]
                }
              }
            }
          }
          event Mouse Down {
            n765 = event-data() -> ("CtlRef"=w1521:refnum<vi>, "Coords"=w1527:T26)  [unwired: 1 in, 6 out]
            n766 = invoke on="Invoke Node" class="LstBox (strict)" method="Point To Row"(reference=w1521, "Point"=w1527) -> ("InBounds"=w1522:bool, "Row"=w1523:i32)  [unwired: 5 in, 5 out]
            n767 = property on="Property Node" class="LstBox (strict)"(reference=w1521) -> ("Item Symbols"=w1526:i32[])  [unwired: 1 in, 2 out]
            n768 = case shown="True" w1522 {
              tunnel: w1521 -> [_ w1529]
              tunnel: w1526 -> [_ w1537]
              tunnel: w1523 -> [_ w1536]
              frame False {
              }
              frame True {
                n769 = Index Array(array=w1537, index=w1536) -> (element=w1539:i32)
                n770 = control-ref of="Thermocouples Selected"() -> (w1528:refnum<vi>)
                n771 = Equal?(x=w1539, y=37) -> (x = y?=w1534:bool)
                n772 = case shown="True" w1534 {
                  tunnel: w1537 -> [w1552 w1566]
                  tunnel: w1536 -> [w1549 w1562]
                  tunnel: [w1551 w1564] -> w1531
                  tunnel: w1528 -> [w1550 w1563]
                  frame False {
                    n773 = Not Equal To 0?(x=w1549) -> (x != 0?=w1548:bool)
                    n774 = case shown="True" w1548 {
                      tunnel: w1549 -> [_ w1560]
                      tunnel: w1550 -> [_ w1559]
                      frame False {
                      }
                      frame True {
                        n775 = property class="Str"(reference=w1559) -> (reference out=w1558:refnum<vi>, "Text.Text"=w1555:string)  [unwired: 1 in, 1 out]
                        n776 = Number To Decimal String(number=w1560) -> (decimal integer string=w1557:string)  [unwired: 1 in]
                        n777 = call <vilib>:"Space Constant.vi"() -> ("String"=w1556:string)
                        n778 = Search and Replace String(input string=w1555, search string=w1557, replace string=w1556) -> (result string=w1554:string)  [unwired: 5 in, 3 out]
                        n779 = property class="Str"(reference=w1558, "Text.Text"=w1554) -> ()  [unwired: 1 in, 2 out]
                      }
                    }
                    n780 = Replace Array Subset(array=w1552, new element=37, index=w1549) -> (w1551:i32[])
                  }
                  frame True {
                    n781 = Not Equal To 0?(x=w1562) -> (x != 0?=w1561:bool)
                    n782 = case shown="False" w1561 {
                      tunnel: w1563 -> [w1567 w1574]
                      tunnel: w1562 -> [_ w1573]
                      frame False {
                        n783 = property class="Str"(reference=w1567, "Text.Text"="") -> ()  [unwired: 1 in, 2 out]
                      }
                      frame True {
                        n784 = property class="Str"(reference=w1574) -> ("Text.Text"=w1572:string)  [unwired: 1 in, 2 out]
                        n785 = Number To Decimal String(number=w1573) -> (decimal integer string=w1569:string)  [unwired: 1 in]
                        n786 = call <vilib>:"Space Constant.vi"() -> ("String"=w1570:string)
                        n787 = Concatenate Strings(w1572, w1570, w1569) -> (w1571:string)
                        n788 = property class="Str"(reference=w1574, "Text.Text"=w1571) -> ()  [unwired: 1 in, 2 out]
                      }
                    }
                    n789 = Replace Array Subset(array=w1566, new element=38, index=w1562) -> (w1564:i32[])
                  }
                }
                n790 = Equal To 0?(x=w1536) -> (x = 0?=w1535:bool)
                n791 = Array Size(array=w1531) -> (size(s)=w1530:i32)
                n792 = And(x=w1534, y=w1535) -> (x .and. y?=w1533:bool)
                n793 = case shown="True" w1533 {
                  tunnel: w1531 -> [w1540 w1543]
                  tunnel: [w1540 w1542] -> w1532
                  tunnel: w1530 -> [_ w1541]
                  frame False {
                  }
                  frame True {
                    n794 = for {
                      N: w1541 -> [_]
                      shift-right: [w1544] -> w1542
                      shift-left: w1543 -> [w1547]
                      i -> [w1546]
                      n795 = Replace Array Subset(array=w1547, new element=37, index=w1546) -> (w1544:i32[])
                    }
                  }
                }
                n796 = property on="Property Node" class="LstBox (strict)"(reference=w1529, "Item Symbols"=w1532) -> ()  [unwired: 1 in, 2 out]
              }
            }
          }
          event Mouse Down {
            n797 = event-data() -> ("CtlRef"=w1575:refnum<vi>, "Coords"=w1581:T26)  [unwired: 1 in, 6 out]
            n798 = invoke on="Invoke Node" class="LstBox (strict)" method="Point To Row"(reference=w1575, "Point"=w1581) -> ("InBounds"=w1576:bool, "Row"=w1577:i32)  [unwired: 5 in, 5 out]
            n799 = property on="Property Node" class="LstBox (strict)"(reference=w1575) -> ("Item Symbols"=w1580:i32[])  [unwired: 1 in, 2 out]
            n800 = case shown="True" w1576 {
              tunnel: w1575 -> [_ w1583]
              tunnel: w1580 -> [_ w1591]
              tunnel: w1577 -> [_ w1590]
              frame False {
              }
              frame True {
                n801 = Index Array(array=w1591, index=w1590) -> (element=w1593:i32)
                n802 = control-ref of="Thermocouples Selected"() -> (w1582:refnum<vi>)
                n803 = Equal?(x=w1593, y=37) -> (x = y?=w1588:bool)
                n804 = case shown="True" w1588 {
                  tunnel: w1591 -> [w1606 w1620]
                  tunnel: w1590 -> [w1603 w1616]
                  tunnel: [w1605 w1618] -> w1585
                  tunnel: w1582 -> [w1604 w1617]
                  frame False {
                    n805 = Not Equal To 0?(x=w1603) -> (x != 0?=w1602:bool)
                    n806 = case shown="True" w1602 {
                      tunnel: w1603 -> [_ w1614]
                      tunnel: w1604 -> [_ w1613]
                      frame False {
                      }
                      frame True {
                        n807 = property class="Str"(reference=w1613) -> (reference out=w1612:refnum<vi>, "Text.Text"=w1609:string)  [unwired: 1 in, 1 out]
                        n808 = Number To Decimal String(number=w1614) -> (decimal integer string=w1611:string)  [unwired: 1 in]
                        n809 = call <vilib>:"Space Constant.vi"() -> ("String"=w1610:string)
                        n810 = Search and Replace String(input string=w1609, search string=w1611, replace string=w1610) -> (result string=w1608:string)  [unwired: 5 in, 3 out]
                        n811 = property class="Str"(reference=w1612, "Text.Text"=w1608) -> ()  [unwired: 1 in, 2 out]
                      }
                    }
                    n812 = Replace Array Subset(array=w1606, new element=37, index=w1603) -> (w1605:i32[])
                  }
                  frame True {
                    n813 = Not Equal To 0?(x=w1616) -> (x != 0?=w1615:bool)
                    n814 = case shown="True" w1615 {
                      tunnel: w1617 -> [w1621 w1628]
                      tunnel: w1616 -> [_ w1627]
                      frame False {
                        n815 = property class="Str"(reference=w1621, "Text.Text"="") -> ()  [unwired: 1 in, 2 out]
                      }
                      frame True {
                        n816 = property class="Str"(reference=w1628) -> ("Text.Text"=w1626:string)  [unwired: 1 in, 2 out]
                        n817 = Number To Decimal String(number=w1627) -> (decimal integer string=w1623:string)  [unwired: 1 in]
                        n818 = call <vilib>:"Space Constant.vi"() -> ("String"=w1624:string)
                        n819 = Concatenate Strings(w1626, w1624, w1623) -> (w1625:string)
                        n820 = property class="Str"(reference=w1628, "Text.Text"=w1625) -> ()  [unwired: 1 in, 2 out]
                      }
                    }
                    n821 = Replace Array Subset(array=w1620, new element=38, index=w1616) -> (w1618:i32[])
                  }
                }
                n822 = Equal To 0?(x=w1590) -> (x = 0?=w1589:bool)
                n823 = Array Size(array=w1585) -> (size(s)=w1584:i32)
                n824 = And(x=w1588, y=w1589) -> (x .and. y?=w1587:bool)
                n825 = case shown="True" w1587 {
                  tunnel: w1585 -> [w1594 w1597]
                  tunnel: [w1594 w1596] -> w1586
                  tunnel: w1584 -> [_ w1595]
                  frame False {
                  }
                  frame True {
                    n826 = for {
                      N: w1595 -> [_]
                      shift-right: [w1598] -> w1596
                      shift-left: w1597 -> [w1601]
                      i -> [w1600]
                      n827 = Replace Array Subset(array=w1601, new element=37, index=w1600) -> (w1598:i32[])
                    }
                  }
                }
                n828 = property on="Property Node" class="LstBox (strict)"(reference=w1583, "Item Symbols"=w1586) -> ()  [unwired: 1 in, 2 out]
              }
            }
          }
          event Mouse Down {
            n829 = event-data() -> ("CtlRef"=w1629:refnum<vi>, "Coords"=w1635:T26)  [unwired: 1 in, 6 out]
            n830 = invoke on="Invoke Node" class="LstBox (strict)" method="Point To Row"(reference=w1629, "Point"=w1635) -> ("InBounds"=w1630:bool, "Row"=w1631:i32)  [unwired: 5 in, 5 out]
            n831 = property on="Property Node" class="LstBox (strict)"(reference=w1629) -> ("Item Symbols"=w1634:i32[])  [unwired: 1 in, 2 out]
            n832 = case shown="True" w1630 {
              tunnel: w1629 -> [_ w1637]
              tunnel: w1634 -> [_ w1645]
              tunnel: w1631 -> [_ w1644]
              frame False {
              }
              frame True {
                n833 = Index Array(array=w1645, index=w1644) -> (element=w1647:i32)
                n834 = control-ref of="Thermocouples Selected"() -> (w1636:refnum<vi>)
                n835 = Equal?(x=w1647, y=37) -> (x = y?=w1642:bool)
                n836 = case shown="True" w1642 {
                  tunnel: w1645 -> [w1660 w1674]
                  tunnel: w1644 -> [w1657 w1670]
                  tunnel: [w1659 w1672] -> w1639
                  tunnel: w1636 -> [w1658 w1671]
                  frame False {
                    n837 = Not Equal To 0?(x=w1657) -> (x != 0?=w1656:bool)
                    n838 = case shown="True" w1656 {
                      tunnel: w1657 -> [_ w1668]
                      tunnel: w1658 -> [_ w1667]
                      frame False {
                      }
                      frame True {
                        n839 = property class="Str"(reference=w1667) -> (reference out=w1666:refnum<vi>, "Text.Text"=w1663:string)  [unwired: 1 in, 1 out]
                        n840 = Number To Decimal String(number=w1668) -> (decimal integer string=w1665:string)  [unwired: 1 in]
                        n841 = call <vilib>:"Space Constant.vi"() -> ("String"=w1664:string)
                        n842 = Search and Replace String(input string=w1663, search string=w1665, replace string=w1664) -> (result string=w1662:string)  [unwired: 5 in, 3 out]
                        n843 = property class="Str"(reference=w1666, "Text.Text"=w1662) -> ()  [unwired: 1 in, 2 out]
                      }
                    }
                    n844 = Replace Array Subset(array=w1660, new element=37, index=w1657) -> (w1659:i32[])
                  }
                  frame True {
                    n845 = Not Equal To 0?(x=w1670) -> (x != 0?=w1669:bool)
                    n846 = case shown="True" w1669 {
                      tunnel: w1671 -> [w1675 w1682]
                      tunnel: w1670 -> [_ w1681]
                      frame False {
                        n847 = property class="Str"(reference=w1675, "Text.Text"="") -> ()  [unwired: 1 in, 2 out]
                      }
                      frame True {
                        n848 = property class="Str"(reference=w1682) -> ("Text.Text"=w1680:string)  [unwired: 1 in, 2 out]
                        n849 = Number To Decimal String(number=w1681) -> (decimal integer string=w1677:string)  [unwired: 1 in]
                        n850 = call <vilib>:"Space Constant.vi"() -> ("String"=w1678:string)
                        n851 = Concatenate Strings(w1680, w1678, w1677) -> (w1679:string)
                        n852 = property class="Str"(reference=w1682, "Text.Text"=w1679) -> ()  [unwired: 1 in, 2 out]
                      }
                    }
                    n853 = Replace Array Subset(array=w1674, new element=38, index=w1670) -> (w1672:i32[])
                  }
                }
                n854 = Equal To 0?(x=w1644) -> (x = 0?=w1643:bool)
                n855 = Array Size(array=w1639) -> (size(s)=w1638:i32)
                n856 = And(x=w1642, y=w1643) -> (x .and. y?=w1641:bool)
                n857 = case shown="True" w1641 {
                  tunnel: w1639 -> [w1648 w1651]
                  tunnel: [w1648 w1650] -> w1640
                  tunnel: w1638 -> [_ w1649]
                  frame False {
                  }
                  frame True {
                    n858 = for {
                      N: w1649 -> [_]
                      shift-right: [w1652] -> w1650
                      shift-left: w1651 -> [w1655]
                      i -> [w1654]
                      n859 = Replace Array Subset(array=w1655, new element=37, index=w1654) -> (w1652:i32[])
                    }
                  }
                }
                n860 = property on="Property Node" class="LstBox (strict)"(reference=w1637, "Item Symbols"=w1640) -> ()  [unwired: 1 in, 2 out]
              }
            }
          }
          event Mouse Down {
            n861 = event-data() -> ("CtlRef"=w1683:refnum<vi>, "Coords"=w1689:T26)  [unwired: 1 in, 6 out]
            n862 = invoke on="Invoke Node" class="LstBox (strict)" method="Point To Row"(reference=w1683, "Point"=w1689) -> ("InBounds"=w1684:bool, "Row"=w1685:i32)  [unwired: 5 in, 5 out]
            n863 = property on="Property Node" class="LstBox (strict)"(reference=w1683) -> ("Item Symbols"=w1688:i32[])  [unwired: 1 in, 2 out]
            n864 = case shown="True" w1684 {
              tunnel: w1683 -> [_ w1691]
              tunnel: w1688 -> [_ w1699]
              tunnel: w1685 -> [_ w1698]
              frame False {
              }
              frame True {
                n865 = Index Array(array=w1699, index=w1698) -> (element=w1701:i32)
                n866 = control-ref of="Thermocouples Selected"() -> (w1690:refnum<vi>)
                n867 = Equal?(x=w1701, y=37) -> (x = y?=w1696:bool)
                n868 = case shown="True" w1696 {
                  tunnel: w1699 -> [w1714 w1728]
                  tunnel: w1698 -> [w1711 w1724]
                  tunnel: [w1713 w1726] -> w1693
                  tunnel: w1690 -> [w1712 w1725]
                  frame False {
                    n869 = Not Equal To 0?(x=w1711) -> (x != 0?=w1710:bool)
                    n870 = case shown="True" w1710 {
                      tunnel: w1711 -> [_ w1722]
                      tunnel: w1712 -> [_ w1721]
                      frame False {
                      }
                      frame True {
                        n871 = property class="Str"(reference=w1721) -> (reference out=w1720:refnum<vi>, "Text.Text"=w1717:string)  [unwired: 1 in, 1 out]
                        n872 = Number To Decimal String(number=w1722) -> (decimal integer string=w1719:string)  [unwired: 1 in]
                        n873 = call <vilib>:"Space Constant.vi"() -> ("String"=w1718:string)
                        n874 = Search and Replace String(input string=w1717, search string=w1719, replace string=w1718) -> (result string=w1716:string)  [unwired: 5 in, 3 out]
                        n875 = property class="Str"(reference=w1720, "Text.Text"=w1716) -> ()  [unwired: 1 in, 2 out]
                      }
                    }
                    n876 = Replace Array Subset(array=w1714, new element=37, index=w1711) -> (w1713:i32[])
                  }
                  frame True {
                    n877 = Not Equal To 0?(x=w1724) -> (x != 0?=w1723:bool)
                    n878 = case shown="True" w1723 {
                      tunnel: w1725 -> [w1729 w1736]
                      tunnel: w1724 -> [_ w1735]
                      frame False {
                        n879 = property class="Str"(reference=w1729, "Text.Text"="") -> ()  [unwired: 1 in, 2 out]
                      }
                      frame True {
                        n880 = property class="Str"(reference=w1736) -> ("Text.Text"=w1734:string)  [unwired: 1 in, 2 out]
                        n881 = Number To Decimal String(number=w1735) -> (decimal integer string=w1731:string)  [unwired: 1 in]
                        n882 = call <vilib>:"Space Constant.vi"() -> ("String"=w1732:string)
                        n883 = Concatenate Strings(w1734, w1732, w1731) -> (w1733:string)
                        n884 = property class="Str"(reference=w1736, "Text.Text"=w1733) -> ()  [unwired: 1 in, 2 out]
                      }
                    }
                    n885 = Replace Array Subset(array=w1728, new element=38, index=w1724) -> (w1726:i32[])
                  }
                }
                n886 = Equal To 0?(x=w1698) -> (x = 0?=w1697:bool)
                n887 = Array Size(array=w1693) -> (size(s)=w1692:i32)
                n888 = And(x=w1696, y=w1697) -> (x .and. y?=w1695:bool)
                n889 = case shown="True" w1695 {
                  tunnel: w1693 -> [w1702 w1705]
                  tunnel: [w1702 w1704] -> w1694
                  tunnel: w1692 -> [_ w1703]
                  frame False {
                  }
                  frame True {
                    n890 = for {
                      N: w1703 -> [_]
                      shift-right: [w1706] -> w1704
                      shift-left: w1705 -> [w1709]
                      i -> [w1708]
                      n891 = Replace Array Subset(array=w1709, new element=37, index=w1708) -> (w1706:i32[])
                    }
                  }
                }
                n892 = property on="Property Node" class="LstBox (strict)"(reference=w1691, "Item Symbols"=w1694) -> ()  [unwired: 1 in, 2 out]
              }
            }
          }
          event Mouse Down {
            n893 = event-data() -> ("CtlRef"=w1737:refnum<vi>, "Coords"=w1743:T26)  [unwired: 1 in, 6 out]
            n894 = invoke on="Invoke Node" class="LstBox (strict)" method="Point To Row"(reference=w1737, "Point"=w1743) -> ("InBounds"=w1738:bool, "Row"=w1739:i32)  [unwired: 5 in, 5 out]
            n895 = property on="Property Node" class="LstBox (strict)"(reference=w1737) -> ("Item Symbols"=w1742:i32[])  [unwired: 1 in, 2 out]
            n896 = case shown="True" w1738 {
              tunnel: w1737 -> [_ w1745]
              tunnel: w1742 -> [_ w1753]
              tunnel: w1739 -> [_ w1752]
              frame False {
              }
              frame True {
                n897 = Index Array(array=w1753, index=w1752) -> (element=w1755:i32)
                n898 = control-ref of="Thermocouples Selected"() -> (w1744:refnum<vi>)
                n899 = Equal?(x=w1755, y=37) -> (x = y?=w1750:bool)
                n900 = case shown="True" w1750 {
                  tunnel: w1753 -> [w1768 w1782]
                  tunnel: w1752 -> [w1765 w1778]
                  tunnel: [w1767 w1780] -> w1747
                  tunnel: w1744 -> [w1766 w1779]
                  frame False {
                    n901 = Not Equal To 0?(x=w1765) -> (x != 0?=w1764:bool)
                    n902 = case shown="True" w1764 {
                      tunnel: w1765 -> [_ w1776]
                      tunnel: w1766 -> [_ w1775]
                      frame False {
                      }
                      frame True {
                        n903 = property class="Str"(reference=w1775) -> (reference out=w1774:refnum<vi>, "Text.Text"=w1771:string)  [unwired: 1 in, 1 out]
                        n904 = Number To Decimal String(number=w1776) -> (decimal integer string=w1773:string)  [unwired: 1 in]
                        n905 = call <vilib>:"Space Constant.vi"() -> ("String"=w1772:string)
                        n906 = Search and Replace String(input string=w1771, search string=w1773, replace string=w1772) -> (result string=w1770:string)  [unwired: 5 in, 3 out]
                        n907 = property class="Str"(reference=w1774, "Text.Text"=w1770) -> ()  [unwired: 1 in, 2 out]
                      }
                    }
                    n908 = Replace Array Subset(array=w1768, new element=37, index=w1765) -> (w1767:i32[])
                  }
                  frame True {
                    n909 = Not Equal To 0?(x=w1778) -> (x != 0?=w1777:bool)
                    n910 = case shown="True" w1777 {
                      tunnel: w1779 -> [w1783 w1790]
                      tunnel: w1778 -> [_ w1789]
                      frame False {
                        n911 = property class="Str"(reference=w1783, "Text.Text"="") -> ()  [unwired: 1 in, 2 out]
                      }
                      frame True {
                        n912 = property class="Str"(reference=w1790) -> ("Text.Text"=w1788:string)  [unwired: 1 in, 2 out]
                        n913 = Number To Decimal String(number=w1789) -> (decimal integer string=w1785:string)  [unwired: 1 in]
                        n914 = call <vilib>:"Space Constant.vi"() -> ("String"=w1786:string)
                        n915 = Concatenate Strings(w1788, w1786, w1785) -> (w1787:string)
                        n916 = property class="Str"(reference=w1790, "Text.Text"=w1787) -> ()  [unwired: 1 in, 2 out]
                      }
                    }
                    n917 = Replace Array Subset(array=w1782, new element=38, index=w1778) -> (w1780:i32[])
                  }
                }
                n918 = Equal To 0?(x=w1752) -> (x = 0?=w1751:bool)
                n919 = Array Size(array=w1747) -> (size(s)=w1746:i32)
                n920 = And(x=w1750, y=w1751) -> (x .and. y?=w1749:bool)
                n921 = case shown="True" w1749 {
                  tunnel: w1747 -> [w1756 w1759]
                  tunnel: [w1756 w1758] -> w1748
                  tunnel: w1746 -> [_ w1757]
                  frame False {
                  }
                  frame True {
                    n922 = for {
                      N: w1757 -> [_]
                      shift-right: [w1760] -> w1758
                      shift-left: w1759 -> [w1763]
                      i -> [w1762]
                      n923 = Replace Array Subset(array=w1763, new element=37, index=w1762) -> (w1760:i32[])
                    }
                  }
                }
                n924 = property on="Property Node" class="LstBox (strict)"(reference=w1745, "Item Symbols"=w1748) -> ()  [unwired: 1 in, 2 out]
              }
            }
          }
          event Mouse Down {
            n925 = event-data() -> ("CtlRef"=w1791:refnum<vi>, "Coords"=w1797:T26)  [unwired: 1 in, 6 out]
            n926 = invoke on="Invoke Node" class="LstBox (strict)" method="Point To Row"(reference=w1791, "Point"=w1797) -> ("InBounds"=w1792:bool, "Row"=w1793:i32)  [unwired: 5 in, 5 out]
            n927 = property on="Property Node" class="LstBox (strict)"(reference=w1791) -> ("Item Symbols"=w1796:i32[])  [unwired: 1 in, 2 out]
            n928 = case shown="True" w1792 {
              tunnel: w1791 -> [_ w1799]
              tunnel: w1796 -> [_ w1807]
              tunnel: w1793 -> [_ w1806]
              frame False {
              }
              frame True {
                n929 = Index Array(array=w1807, index=w1806) -> (element=w1809:i32)
                n930 = control-ref of="Thermocouples Selected"() -> (w1798:refnum<vi>)
                n931 = Equal?(x=w1809, y=37) -> (x = y?=w1804:bool)
                n932 = case shown="True" w1804 {
                  tunnel: w1807 -> [w1822 w1836]
                  tunnel: w1806 -> [w1819 w1832]
                  tunnel: [w1821 w1834] -> w1801
                  tunnel: w1798 -> [w1820 w1833]
                  frame False {
                    n933 = Not Equal To 0?(x=w1819) -> (x != 0?=w1818:bool)
                    n934 = case shown="True" w1818 {
                      tunnel: w1819 -> [_ w1830]
                      tunnel: w1820 -> [_ w1829]
                      frame False {
                      }
                      frame True {
                        n935 = property class="Str"(reference=w1829) -> (reference out=w1828:refnum<vi>, "Text.Text"=w1825:string)  [unwired: 1 in, 1 out]
                        n936 = Number To Decimal String(number=w1830) -> (decimal integer string=w1827:string)  [unwired: 1 in]
                        n937 = call <vilib>:"Space Constant.vi"() -> ("String"=w1826:string)
                        n938 = Search and Replace String(input string=w1825, search string=w1827, replace string=w1826) -> (result string=w1824:string)  [unwired: 5 in, 3 out]
                        n939 = property class="Str"(reference=w1828, "Text.Text"=w1824) -> ()  [unwired: 1 in, 2 out]
                      }
                    }
                    n940 = Replace Array Subset(array=w1822, new element=37, index=w1819) -> (w1821:i32[])
                  }
                  frame True {
                    n941 = Not Equal To 0?(x=w1832) -> (x != 0?=w1831:bool)
                    n942 = case shown="True" w1831 {
                      tunnel: w1833 -> [w1837 w1844]
                      tunnel: w1832 -> [_ w1843]
                      frame False {
                        n943 = property class="Str"(reference=w1837, "Text.Text"="") -> ()  [unwired: 1 in, 2 out]
                      }
                      frame True {
                        n944 = property class="Str"(reference=w1844) -> ("Text.Text"=w1842:string)  [unwired: 1 in, 2 out]
                        n945 = Number To Decimal String(number=w1843) -> (decimal integer string=w1839:string)  [unwired: 1 in]
                        n946 = call <vilib>:"Space Constant.vi"() -> ("String"=w1840:string)
                        n947 = Concatenate Strings(w1842, w1840, w1839) -> (w1841:string)
                        n948 = property class="Str"(reference=w1844, "Text.Text"=w1841) -> ()  [unwired: 1 in, 2 out]
                      }
                    }
                    n949 = Replace Array Subset(array=w1836, new element=38, index=w1832) -> (w1834:i32[])
                  }
                }
                n950 = Equal To 0?(x=w1806) -> (x = 0?=w1805:bool)
                n951 = Array Size(array=w1801) -> (size(s)=w1800:i32)
                n952 = And(x=w1804, y=w1805) -> (x .and. y?=w1803:bool)
                n953 = case shown="True" w1803 {
                  tunnel: w1801 -> [w1810 w1813]
                  tunnel: [w1810 w1812] -> w1802
                  tunnel: w1800 -> [_ w1811]
                  frame False {
                  }
                  frame True {
                    n954 = for {
                      N: w1811 -> [_]
                      shift-right: [w1814] -> w1812
                      shift-left: w1813 -> [w1817]
                      i -> [w1816]
                      n955 = Replace Array Subset(array=w1817, new element=37, index=w1816) -> (w1814:i32[])
                    }
                  }
                }
                n956 = property on="Property Node" class="LstBox (strict)"(reference=w1799, "Item Symbols"=w1802) -> ()  [unwired: 1 in, 2 out]
              }
            }
          }
          event Mouse Down {
            n957 = event-data() -> ("CtlRef"=w1845:refnum<vi>, "Coords"=w1851:T26)  [unwired: 1 in, 6 out]
            n958 = invoke on="Invoke Node" class="LstBox (strict)" method="Point To Row"(reference=w1845, "Point"=w1851) -> ("InBounds"=w1846:bool, "Row"=w1847:i32)  [unwired: 5 in, 5 out]
            n959 = property on="Property Node" class="LstBox (strict)"(reference=w1845) -> ("Item Symbols"=w1850:i32[])  [unwired: 1 in, 2 out]
            n960 = case shown="True" w1846 {
              tunnel: w1845 -> [_ w1853]
              tunnel: w1850 -> [_ w1861]
              tunnel: w1847 -> [_ w1860]
              frame False {
              }
              frame True {
                n961 = Index Array(array=w1861, index=w1860) -> (element=w1863:i32)
                n962 = control-ref of="Thermocouples Selected"() -> (w1852:refnum<vi>)
                n963 = Equal?(x=w1863, y=37) -> (x = y?=w1858:bool)
                n964 = case shown="True" w1858 {
                  tunnel: w1861 -> [w1876 w1890]
                  tunnel: w1860 -> [w1873 w1886]
                  tunnel: [w1875 w1888] -> w1855
                  tunnel: w1852 -> [w1874 w1887]
                  frame False {
                    n965 = Not Equal To 0?(x=w1873) -> (x != 0?=w1872:bool)
                    n966 = case shown="True" w1872 {
                      tunnel: w1873 -> [_ w1884]
                      tunnel: w1874 -> [_ w1883]
                      frame False {
                      }
                      frame True {
                        n967 = property class="Str"(reference=w1883) -> (reference out=w1882:refnum<vi>, "Text.Text"=w1879:string)  [unwired: 1 in, 1 out]
                        n968 = Number To Decimal String(number=w1884) -> (decimal integer string=w1881:string)  [unwired: 1 in]
                        n969 = call <vilib>:"Space Constant.vi"() -> ("String"=w1880:string)
                        n970 = Search and Replace String(input string=w1879, search string=w1881, replace string=w1880) -> (result string=w1878:string)  [unwired: 5 in, 3 out]
                        n971 = property class="Str"(reference=w1882, "Text.Text"=w1878) -> ()  [unwired: 1 in, 2 out]
                      }
                    }
                    n972 = Replace Array Subset(array=w1876, new element=37, index=w1873) -> (w1875:i32[])
                  }
                  frame True {
                    n973 = Not Equal To 0?(x=w1886) -> (x != 0?=w1885:bool)
                    n974 = case shown="True" w1885 {
                      tunnel: w1887 -> [w1891 w1898]
                      tunnel: w1886 -> [_ w1897]
                      frame False {
                        n975 = property class="Str"(reference=w1891, "Text.Text"="") -> ()  [unwired: 1 in, 2 out]
                      }
                      frame True {
                        n976 = property class="Str"(reference=w1898) -> ("Text.Text"=w1896:string)  [unwired: 1 in, 2 out]
                        n977 = Number To Decimal String(number=w1897) -> (decimal integer string=w1893:string)  [unwired: 1 in]
                        n978 = call <vilib>:"Space Constant.vi"() -> ("String"=w1894:string)
                        n979 = Concatenate Strings(w1896, w1894, w1893) -> (w1895:string)
                        n980 = property class="Str"(reference=w1898, "Text.Text"=w1895) -> ()  [unwired: 1 in, 2 out]
                      }
                    }
                    n981 = Replace Array Subset(array=w1890, new element=38, index=w1886) -> (w1888:i32[])
                  }
                }
                n982 = Equal To 0?(x=w1860) -> (x = 0?=w1859:bool)
                n983 = Array Size(array=w1855) -> (size(s)=w1854:i32)
                n984 = And(x=w1858, y=w1859) -> (x .and. y?=w1857:bool)
                n985 = case shown="True" w1857 {
                  tunnel: w1855 -> [w1864 w1867]
                  tunnel: [w1864 w1866] -> w1856
                  tunnel: w1854 -> [_ w1865]
                  frame False {
                  }
                  frame True {
                    n986 = for {
                      N: w1865 -> [_]
                      shift-right: [w1868] -> w1866
                      shift-left: w1867 -> [w1871]
                      i -> [w1870]
                      n987 = Replace Array Subset(array=w1871, new element=37, index=w1870) -> (w1868:i32[])
                    }
                  }
                }
                n988 = property on="Property Node" class="LstBox (strict)"(reference=w1853, "Item Symbols"=w1856) -> ()  [unwired: 1 in, 2 out]
              }
            }
          }
          event Mouse Down {
            n989 = event-data() -> ("CtlRef"=w1899:refnum<vi>, "Coords"=w1905:T26)  [unwired: 1 in, 6 out]
            n990 = invoke on="Invoke Node" class="LstBox (strict)" method="Point To Row"(reference=w1899, "Point"=w1905) -> ("InBounds"=w1900:bool, "Row"=w1901:i32)  [unwired: 5 in, 5 out]
            n991 = property on="Property Node" class="LstBox (strict)"(reference=w1899) -> ("Item Symbols"=w1904:i32[])  [unwired: 1 in, 2 out]
            n992 = case shown="True" w1900 {
              tunnel: w1899 -> [_ w1907]
              tunnel: w1904 -> [_ w1915]
              tunnel: w1901 -> [_ w1914]
              frame False {
              }
              frame True {
                n993 = Index Array(array=w1915, index=w1914) -> (element=w1917:i32)
                n994 = control-ref of="Thermocouples Selected"() -> (w1906:refnum<vi>)
                n995 = Equal?(x=w1917, y=37) -> (x = y?=w1912:bool)
                n996 = case shown="True" w1912 {
                  tunnel: w1915 -> [w1930 w1944]
                  tunnel: w1914 -> [w1927 w1940]
                  tunnel: [w1929 w1942] -> w1909
                  tunnel: w1906 -> [w1928 w1941]
                  frame False {
                    n997 = Not Equal To 0?(x=w1927) -> (x != 0?=w1926:bool)
                    n998 = case shown="True" w1926 {
                      tunnel: w1927 -> [_ w1938]
                      tunnel: w1928 -> [_ w1937]
                      frame False {
                      }
                      frame True {
                        n999 = property class="Str"(reference=w1937) -> (reference out=w1936:refnum<vi>, "Text.Text"=w1933:string)  [unwired: 1 in, 1 out]
                        n1000 = Number To Decimal String(number=w1938) -> (decimal integer string=w1935:string)  [unwired: 1 in]
                        n1001 = call <vilib>:"Space Constant.vi"() -> ("String"=w1934:string)
                        n1002 = Search and Replace String(input string=w1933, search string=w1935, replace string=w1934) -> (result string=w1932:string)  [unwired: 5 in, 3 out]
                        n1003 = property class="Str"(reference=w1936, "Text.Text"=w1932) -> ()  [unwired: 1 in, 2 out]
                      }
                    }
                    n1004 = Replace Array Subset(array=w1930, new element=37, index=w1927) -> (w1929:i32[])
                  }
                  frame True {
                    n1005 = Not Equal To 0?(x=w1940) -> (x != 0?=w1939:bool)
                    n1006 = case shown="True" w1939 {
                      tunnel: w1941 -> [w1945 w1952]
                      tunnel: w1940 -> [_ w1951]
                      frame False {
                        n1007 = property class="Str"(reference=w1945, "Text.Text"="") -> ()  [unwired: 1 in, 2 out]
                      }
                      frame True {
                        n1008 = property class="Str"(reference=w1952) -> ("Text.Text"=w1950:string)  [unwired: 1 in, 2 out]
                        n1009 = Number To Decimal String(number=w1951) -> (decimal integer string=w1947:string)  [unwired: 1 in]
                        n1010 = call <vilib>:"Space Constant.vi"() -> ("String"=w1948:string)
                        n1011 = Concatenate Strings(w1950, w1948, w1947) -> (w1949:string)
                        n1012 = property class="Str"(reference=w1952, "Text.Text"=w1949) -> ()  [unwired: 1 in, 2 out]
                      }
                    }
                    n1013 = Replace Array Subset(array=w1944, new element=38, index=w1940) -> (w1942:i32[])
                  }
                }
                n1014 = Equal To 0?(x=w1914) -> (x = 0?=w1913:bool)
                n1015 = Array Size(array=w1909) -> (size(s)=w1908:i32)
                n1016 = And(x=w1912, y=w1913) -> (x .and. y?=w1911:bool)
                n1017 = case shown="True" w1911 {
                  tunnel: w1909 -> [w1918 w1921]
                  tunnel: [w1918 w1920] -> w1910
                  tunnel: w1908 -> [_ w1919]
                  frame False {
                  }
                  frame True {
                    n1018 = for {
                      N: w1919 -> [_]
                      shift-right: [w1922] -> w1920
                      shift-left: w1921 -> [w1925]
                      i -> [w1924]
                      n1019 = Replace Array Subset(array=w1925, new element=37, index=w1924) -> (w1922:i32[])
                    }
                  }
                }
                n1020 = property on="Property Node" class="LstBox (strict)"(reference=w1907, "Item Symbols"=w1910) -> ()  [unwired: 1 in, 2 out]
              }
            }
          }
          event Mouse Down {
            n1021 = event-data() -> ("CtlRef"=w1953:refnum<vi>, "Coords"=w1959:T26)  [unwired: 1 in, 6 out]
            n1022 = invoke on="Invoke Node" class="LstBox (strict)" method="Point To Row"(reference=w1953, "Point"=w1959) -> ("InBounds"=w1954:bool, "Row"=w1955:i32)  [unwired: 5 in, 5 out]
            n1023 = property on="Property Node" class="LstBox (strict)"(reference=w1953) -> ("Item Symbols"=w1958:i32[])  [unwired: 1 in, 2 out]
            n1024 = case shown="True" w1954 {
              tunnel: w1953 -> [_ w1961]
              tunnel: w1958 -> [_ w1969]
              tunnel: w1955 -> [_ w1968]
              frame False {
              }
              frame True {
                n1025 = Index Array(array=w1969, index=w1968) -> (element=w1971:i32)
                n1026 = control-ref of="Thermocouples Selected"() -> (w1960:refnum<vi>)
                n1027 = Equal?(x=w1971, y=37) -> (x = y?=w1966:bool)
                n1028 = case shown="True" w1966 {
                  tunnel: w1969 -> [w1984 w1998]
                  tunnel: w1968 -> [w1981 w1994]
                  tunnel: [w1983 w1996] -> w1963
                  tunnel: w1960 -> [w1982 w1995]
                  frame False {
                    n1029 = Not Equal To 0?(x=w1981) -> (x != 0?=w1980:bool)
                    n1030 = case shown="True" w1980 {
                      tunnel: w1981 -> [_ w1992]
                      tunnel: w1982 -> [_ w1991]
                      frame False {
                      }
                      frame True {
                        n1031 = property class="Str"(reference=w1991) -> (reference out=w1990:refnum<vi>, "Text.Text"=w1987:string)  [unwired: 1 in, 1 out]
                        n1032 = Number To Decimal String(number=w1992) -> (decimal integer string=w1989:string)  [unwired: 1 in]
                        n1033 = call <vilib>:"Space Constant.vi"() -> ("String"=w1988:string)
                        n1034 = Search and Replace String(input string=w1987, search string=w1989, replace string=w1988) -> (result string=w1986:string)  [unwired: 5 in, 3 out]
                        n1035 = property class="Str"(reference=w1990, "Text.Text"=w1986) -> ()  [unwired: 1 in, 2 out]
                      }
                    }
                    n1036 = Replace Array Subset(array=w1984, new element=37, index=w1981) -> (w1983:i32[])
                  }
                  frame True {
                    n1037 = Not Equal To 0?(x=w1994) -> (x != 0?=w1993:bool)
                    n1038 = case shown="True" w1993 {
                      tunnel: w1995 -> [w1999 w2006]
                      tunnel: w1994 -> [_ w2005]
                      frame False {
                        n1039 = property class="Str"(reference=w1999, "Text.Text"="") -> ()  [unwired: 1 in, 2 out]
                      }
                      frame True {
                        n1040 = property class="Str"(reference=w2006) -> ("Text.Text"=w2004:string)  [unwired: 1 in, 2 out]
                        n1041 = Number To Decimal String(number=w2005) -> (decimal integer string=w2001:string)  [unwired: 1 in]
                        n1042 = call <vilib>:"Space Constant.vi"() -> ("String"=w2002:string)
                        n1043 = Concatenate Strings(w2004, w2002, w2001) -> (w2003:string)
                        n1044 = property class="Str"(reference=w2006, "Text.Text"=w2003) -> ()  [unwired: 1 in, 2 out]
                      }
                    }
                    n1045 = Replace Array Subset(array=w1998, new element=38, index=w1994) -> (w1996:i32[])
                  }
                }
                n1046 = Equal To 0?(x=w1968) -> (x = 0?=w1967:bool)
                n1047 = Array Size(array=w1963) -> (size(s)=w1962:i32)
                n1048 = And(x=w1966, y=w1967) -> (x .and. y?=w1965:bool)
                n1049 = case shown="True" w1965 {
                  tunnel: w1963 -> [w1972 w1975]
                  tunnel: [w1972 w1974] -> w1964
                  tunnel: w1962 -> [_ w1973]
                  frame False {
                  }
                  frame True {
                    n1050 = for {
                      N: w1973 -> [_]
                      shift-right: [w1976] -> w1974
                      shift-left: w1975 -> [w1979]
                      i -> [w1978]
                      n1051 = Replace Array Subset(array=w1979, new element=37, index=w1978) -> (w1976:i32[])
                    }
                  }
                }
                n1052 = property on="Property Node" class="LstBox (strict)"(reference=w1961, "Item Symbols"=w1964) -> ()  [unwired: 1 in, 2 out]
              }
            }
          }
          event "TC1to45visual": Mouse Move {
            n1053 = event-data() -> ("Coords"=w2011:T26)  [unwired: 1 in]
            n1054 = local read "Moving 1"() -> (w2012:bool)
            n1055 = case shown="False" w2012 {
              tunnel: w2011 -> [w2017 w2050]
              tunnel: w2010 -> [w2015 w2053]
              tunnel: [w2015 w2053] -> w2007
              tunnel: w2009 -> [w2014 w2052]
              frame False {
                n1056 = control-ref of="TC1to45visual"() -> (w2013:refnum<vi>)
                n1057 = property class="Clust (strict)"(reference=w2013) -> ("Controls[]"=w2016:refnum<vi>[])  [unwired: 1 in, 2 out]
                n1058 = for {
                  N: 45 -> [_]
                  shift-right: [w2019] -> _
                  shift-left: w2017 -> [w2021]
                  tunnel: w2016 -> [w2035] mode=indexing
                  tunnel: w2014 -> [w2020]
                  n1059 = property class="Ctl"(reference=w2035) -> (reference out=w2022:refnum<vi>, "Position"=w2025:T1)  [unwired: 1 in, 1 out]
                  n1060 = Unbundle By Name(w2021) -> ("Horizontal"=w2031:i32, "Vertical"=w2030:i32)
                  n1061 = Unbundle By Name(w2025) -> ("Left"=w2023:i32, "Top"=w2028:i32)
                  n1062 = Add(x=w2028, y=24) -> (x+y=w2029:i32)
                  n1063 = Add(x=w2023, y=32) -> (x+y=w2034:i32)
                  n1064 = In Range and Coerce(upper limit=w2034, x=w2031, lower limit=w2023) -> (In Range?=w2027:bool)  [unwired: 1 out]
                  n1065 = In Range and Coerce(upper limit=w2029, x=w2030, lower limit=w2028) -> (In Range?=w2026:bool)  [unwired: 1 out]
                  n1066 = And(x=w2027, y=w2026) -> (x .and. y?=w2024:bool)
                  n1067 = case shown="True" w2024 {
                    tunnel: w2022 -> [_ w2038]
                    tunnel: w2021 -> [w2036 w2039]
                    tunnel: w2020 -> [_ w2040]
                    tunnel: [w2036 w2037] -> w2019
                    frame False {
                    }
                    frame True {
                      n1068 = local write "TC1to45PicRef"(w2038) -> ()
                      n1069 = case shown="True" w2040 {
                        selector: w2040 -> [_ w2049]
                        tunnel: w2039 -> [w2041 w2042]
                        tunnel: w2038 -> [_ w2044]
                        tunnel: [w2041 w2042] -> w2037
                        frame False {
                        }
                        frame True {
                          # "Place control where the mouse is."
                          n1070 = local write "Moving 1"(w2049) -> ()
                          n1071 = property on="Property Node" class="Ctl"(reference=w2044) -> (reference out=w2043:refnum<vi>, "Bounds"=w2048:T16)  [unwired: 1 in, 1 out]
                          n1072 = Divide(x=w2048, y=T16 {"Width"=2, "Height"=2}) -> (x/y=w2046:cluster{"Width":dbl, "Height":dbl})
                          n1073 = Subtract(x=w2042, y=w2046) -> (x-y=w2047:cluster{dbl, dbl})
                          n1074 = property on="Property Node" class="Ctl"(reference=w2043, "Position"=w2047) -> ()  [unwired: 1 in, 2 out]
                        }
                      }
                    }
                  }
                }
              }
              frame True {
                n1075 = local read "TC1to45PicRef"() -> (w2051:refnum<vi>)
                n1076 = case shown="True" w2052 {
                  selector: w2052 -> [_ w2061]
                  tunnel: w2051 -> [_ w2055]
                  tunnel: w2050 -> [_ w2056]
                  frame False {
                  }
                  frame True {
                    # "Place control where the mouse is."
                    n1077 = local write "Moving 1"(w2061) -> ()
                    n1078 = property on="Property Node" class="Ctl"(reference=w2055) -> (reference out=w2054:refnum<vi>, "Bounds"=w2060:T16)  [unwired: 1 in, 1 out]
                    n1079 = Divide(x=w2060, y=T16 {"Width"=2, "Height"=2}) -> (x/y=w2058:cluster{"Width":dbl, "Height":dbl})
                    n1080 = Subtract(x=w2056, y=w2058) -> (x-y=w2059:cluster{dbl, dbl})
                    n1081 = property on="Property Node" class="Ctl"(reference=w2054, "Position"=w2059) -> ()  [unwired: 1 in, 2 out]
                  }
                }
              }
            }
          }
          event "TC1to45visual": Mouse Up {
            # "This case is needed to unlock cursor from the Boolean."
            n1082 = event-data() -> ()  [unwired: 1 in, 1 out]
            n1083 = local write "Moving 1"(FALSE ("stop")) -> ()
          }
          event "TC1to45visual": Mouse Down {
            # "Begin moving Boolean with cursor when the mouse button is pressed."
            n1084 = event-data() -> ()  [unwired: 1 in, 1 out]
          }
          event "Reset All TC Positions": Mouse Down {
            n1085 = event-data() -> ()  [unwired: 1 in, 1 out]
            n1086 = control-ref of="TC1to45visual"() -> (w2073:refnum<vi>)
            n1087 = Unbundle By Name(w2069) -> ("TCs1to45InitialPositions"=w2070:T1[])
            n1088 = property class="Clust (strict)"(reference=w2073) -> ("Controls[]"=w2071:refnum<vi>[])  [unwired: 1 in, 2 out]
            n1089 = for {
              N: 45 -> [_]
              tunnel: w2071 -> [w2076] mode=indexing
              tunnel: w2070 -> [w2075] mode=indexing
              n1090 = property class="Ctl"(reference=w2076, "Position"=w2075) -> ()  [unwired: 1 in, 2 out]
            }
          }
          event "exit": Value Change {
            n1091 = event-data() -> ()  [unwired: 1 in, 1 out]
            n1092 = call "Broadcast Message.vi"("error in (no error)"=w2079, "event"="exit") -> ("error out"=w2077:errorcluster)  [unwired: 9 in]
          }
        }
        n1093 = Bundle By Name(cluster=w299, "Moving 1"=w297) -> (w298:T13)
      }
      frame "compileProfile" {
        n1094 = local write "ThermalProfileStatus"("Compiling..........." ("String")) -> ()
        n1095 = Initialize Array(T18 {"zone"=0, "average"="", "thermocouples"=[0], "maxTemp"=0, "minTemp"=0, "maxSlope"=0, "thermalprofiles"=[{"thermalsetpoint"=0, "tempgoal"=0, "ramp"=0, "soakduration"=0}]} ("ThermalProfileCluster.profiles"), 1 ("dimension size")) -> (w2119:T28)
        n1096 = Unbundle By Name(w2122) -> ("ZonesSelected"=w2123:bool[], "ZoneSetup.Number of Set points"=w2120:dbl)
        n1097 = for {
          N: 9 -> [_]
          tunnel: w2122 -> [w2207]
          tunnel: w2123 -> [w2206] mode=indexing
          shift-right: [w2204] -> w2091
          shift-left: w2122 -> [w2205]
          tunnel: w2120 -> [w2200]
          shift-right: [w2198] -> w2116
          shift-left: w2119 -> [w2199]
          i -> [w2197]
          w2203 = 0  # zone
          n1098 = Add(x=w2203, y=w2197) -> (x+y=w2202:i32)
          n1099 = Increment(x=w2202) -> (x+1=w2201:i32)
          n1100 = case shown="True" w2206 {
            tunnel: w2207 -> [_ _]
            tunnel: w2197 -> [_ w2239]
            tunnel: w2205 -> [w2209 w2243]
            tunnel: [w2209 w2243] -> w2204
            tunnel: w2201 -> [_ w2244]
            tunnel: w2200 -> [_ w2237]
            tunnel: w2199 -> [w2208 w2213]
            tunnel: [w2208 w2212] -> w2198
            tunnel: w2197 -> [_ _]
            frame False {
            }
            frame True {
              n1101 = case shown="0, Default" w2239 {
                tunnel: [w2264 w2270 w2276 w2282 w2288 w2294 w2300 w2306 w2312] -> w2233
                tunnel: [w2263 w2269 w2275 w2281 w2287 w2293 w2299 w2305 w2311] -> w2238
                tunnel: [w2262 w2268 w2274 w2280 w2286 w2292 w2298 w2304 w2310] -> w2228
                tunnel: [w2261 w2267 w2273 w2279 w2285 w2291 w2297 w2303 w2309] -> w2223
                tunnel: [w2260 w2266 w2272 w2278 w2284 w2290 w2296 w2302 w2308] -> w2222
                tunnel: [w2259 w2265 w2271 w2277 w2283 w2289 w2295 w2301 w2307] -> w2218
                frame 0, Default {
                  n1102 = control-ref of="Zone Thermocouples"() -> (w2264:refnum<vi>)
                  n1103 = control-ref of="Temperature Goal"() -> (w2262:refnum<vi>)
                  n1104 = control-ref of="Max Temp Slope"() -> (w2259:refnum<vi>)
                  n1105 = control-ref of="Max Allowable Temp"() -> (w2261:refnum<vi>)
                  n1106 = control-ref of="Temperature Calculation"() -> (w2263:refnum<vi>)
                  n1107 = control-ref of="Min Allowable Temp"() -> (w2260:refnum<vi>)
                }
                frame 1 {
                  n1108 = control-ref of="Zone Thermocouples"() -> (w2270:refnum<vi>)
                  n1109 = control-ref of="Max Temp Slope"() -> (w2265:refnum<vi>)
                  n1110 = control-ref of="Temperature Goal"() -> (w2268:refnum<vi>)
                  n1111 = control-ref of="Max Allowable Temp"() -> (w2267:refnum<vi>)
                  n1112 = control-ref of="Temperature Calculation"() -> (w2269:refnum<vi>)
                  n1113 = control-ref of="Min Allowable Temp"() -> (w2266:refnum<vi>)
                }
                frame 2 {
                  n1114 = control-ref of="Zone Thermocouples"() -> (w2276:refnum<vi>)
                  n1115 = control-ref of="Min Allowable Temp"() -> (w2271:refnum<vi>)
                  n1116 = control-ref of="Temperature Goal"() -> (w2274:refnum<vi>)
                  n1117 = control-ref of="Max Allowable Temp"() -> (w2273:refnum<vi>)
                  n1118 = control-ref of="Temperature Calculation"() -> (w2275:refnum<vi>)
                  n1119 = control-ref of="Min Allowable Temp"() -> (w2272:refnum<vi>)
                }
                frame 3 {
                  n1120 = control-ref of="Zone Thermocouples"() -> (w2282:refnum<vi>)
                  n1121 = control-ref of="Max Temp Slope"() -> (w2277:refnum<vi>)
                  n1122 = control-ref of="Temperature Goal"() -> (w2280:refnum<vi>)
                  n1123 = control-ref of="Max Allowable Temp"() -> (w2279:refnum<vi>)
                  n1124 = control-ref of="Temperature Calculation"() -> (w2281:refnum<vi>)
                  n1125 = control-ref of="Min Allowable Temp"() -> (w2278:refnum<vi>)
                }
                frame 4 {
                  n1126 = control-ref of="Zone Thermocouples"() -> (w2288:refnum<vi>)
                  n1127 = control-ref of="Max Temp Slope"() -> (w2283:refnum<vi>)
                  n1128 = control-ref of="Temperature Goal"() -> (w2286:refnum<vi>)
                  n1129 = control-ref of="Max Allowable Temp"() -> (w2285:refnum<vi>)
                  n1130 = control-ref of="Temperature Calculation"() -> (w2287:refnum<vi>)
                  n1131 = control-ref of="Min Allowable Temp"() -> (w2284:refnum<vi>)
                }
                frame 5 {
                  n1132 = control-ref of="Zone Thermocouples"() -> (w2294:refnum<vi>)
                  n1133 = control-ref of="Max Temp Slope"() -> (w2289:refnum<vi>)
                  n1134 = control-ref of="Temperature Goal"() -> (w2292:refnum<vi>)
                  n1135 = control-ref of="Max Allowable Temp"() -> (w2291:refnum<vi>)
                  n1136 = control-ref of="Temperature Calculation"() -> (w2293:refnum<vi>)
                  n1137 = control-ref of="Min Allowable Temp"() -> (w2290:refnum<vi>)
                }
                frame 6 {
                  n1138 = control-ref of="Zone Thermocouples"() -> (w2300:refnum<vi>)
                  n1139 = control-ref of="Temperature Goal"() -> (w2298:refnum<vi>)
                  n1140 = control-ref of="Max Temp Slope"() -> (w2295:refnum<vi>)
                  n1141 = control-ref of="Max Allowable Temp"() -> (w2297:refnum<vi>)
                  n1142 = control-ref of="Temperature Calculation"() -> (w2299:refnum<vi>)
                  n1143 = control-ref of="Min Allowable Temp"() -> (w2296:refnum<vi>)
                }
                frame 7 {
                  n1144 = control-ref of="Zone Thermocouples"() -> (w2306:refnum<vi>)
                  n1145 = control-ref of="Temperature Goal"() -> (w2304:refnum<vi>)
                  n1146 = control-ref of="Max Temp Slope"() -> (w2301:refnum<vi>)
                  n1147 = control-ref of="Max Allowable Temp"() -> (w2303:refnum<vi>)
                  n1148 = control-ref of="Temperature Calculation"() -> (w2305:refnum<vi>)
                  n1149 = control-ref of="Min Allowable Temp"() -> (w2302:refnum<vi>)
                }
                frame 8 {
                  n1150 = control-ref of="Zone Thermocouples"() -> (w2312:refnum<vi>)
                  n1151 = control-ref of="Temperature Goal"() -> (w2310:refnum<vi>)
                  n1152 = control-ref of="Max Temp Slope"() -> (w2307:refnum<vi>)
                  n1153 = control-ref of="Max Allowable Temp"() -> (w2309:refnum<vi>)
                  n1154 = control-ref of="Temperature Calculation"() -> (w2311:refnum<vi>)
                  n1155 = control-ref of="Min Allowable Temp"() -> (w2308:refnum<vi>)
                }
              }
              n1156 = To Long Integer(number=w2237) -> (32bit integer=w2236:i32)
              n1157 = property class="Arr (strict)"(reference=w2228) -> ("Value"=w2229:dbl[][])  [unwired: 1 in, 2 out]
              n1158 = Initialize Array(T19 {"thermalsetpoint"=0, "tempgoal"=0, "ramp"=0, "soakduration"=0} ("thermalprofiles"), w2236) -> (w2240:T30)
              n1159 = property class="LstBox (strict)"(reference=w2233) -> ("Item Symbols"=w2234:i32[])  [unwired: 1 in, 2 out]
              n1160 = property class="Str"(reference=w2218) -> ("Value"=w2217:string)  [unwired: 1 in, 2 out]
              n1161 = Decimal String To Number(string=w2217) -> (number=w2216:i32)  [unwired: 2 in, 1 out]
              n1162 = control-ref of="RampSoakTimes"() -> (w2230:refnum<vi>)
              n1163 = Array Size(array=w2234) -> (size(s)=w2235:i32)
              n1164 = for {
                N: w2235 -> [_]
                tunnel: w2234 -> [w2254]
                shift-right: [w2250] -> w2231
                shift-left: i32[] [] -> [w2249]
                i -> [w2248]
                n1165 = Index Array(array=w2254, index=w2248) -> (element=w2252:i32)
                n1166 = Equal?(x=w2252, y=38) -> (x = y?=w2253:bool)
                n1167 = case shown="True" w2253 {
                  tunnel: w2248 -> [_ w2258]
                  tunnel: [w2255 w2256] -> w2250
                  tunnel: w2249 -> [w2255 w2257]
                  frame False {
                  }
                  frame True {
                    n1168 = Build Array (concatenate)(w2257, w2258) -> (w2256:i32[])
                  }
                }
              }
              n1169 = property class="Ring (strict)"(reference=w2238) -> ("Value"=w2215:u16)  [unwired: 1 in, 2 out]
              n1170 = property class="Str"(reference=w2222) -> ("Value"=w2224:string)  [unwired: 1 in, 2 out]
              n1171 = property class="Str"(reference=w2223) -> ("Value"=w2225:string)  [unwired: 1 in, 2 out]
              n1172 = property class="Arr (strict)"(reference=w2230) -> ("Value"=w2227:dbl[][])  [unwired: 1 in, 2 out]
              n1173 = for {
                N: w2236 -> [_]
                tunnel: w2229 -> [w2316]
                tunnel: T19 {"thermalsetpoint"=0, "tempgoal"=0, "ramp"=0, "soakduration"=0} ("thermalprofiles") -> [w2329]
                shift-right: [w2327] -> w2226
                shift-left: w2240 -> [w2328]
                tunnel: w2227 -> [w2320]
                i -> [w2323]
                n1174 = Index Array(array=w2316, index (row)=w2323) -> (element=w2315:dbl[])  [unwired: 1 in]
                n1175 = Index Array(array=w2320, index (row)=w2323) -> (element=w2319:dbl[])  [unwired: 1 in]
                n1176 = Index Array(array=w2315, index #1=0 ("index (row)"), index #2=1 ("index (row)")) -> (element #1=w2314:dbl, element #2=w2313:dbl)
                n1177 = Index Array(array=w2319, index #1=1 ("index (row)"), index #2=2 ("index (row)")) -> (element #1=w2318:dbl, element #2=w2317:dbl)
                n1178 = Bundle By Name(cluster=w2329, "thermalsetpoint"=w2314, "tempgoal"=w2313, "ramp"=w2318, "soakduration"=w2317) -> (w2326:T19)
                n1179 = Replace Array Subset(array=w2328, new element=w2326, index=w2323) -> (w2327:T30)
              }
              n1180 = Decimal String To Number(string=w2225) -> (number=w2221:i32)  [unwired: 2 in, 1 out]
              n1181 = Decimal String To Number(string=w2224) -> (number=w2220:i32)  [unwired: 2 in, 1 out]
              n1182 = case shown="0, Default" w2215 {
                tunnel: ["Average" "Min" "Max"] -> w2214
                frame 0, Default {
                }
                frame 1 {
                }
                frame 2 {
                }
              }
              n1183 = Bundle By Name(cluster=T18 {"zone"=0, "average"="", "thermocouples"=[0], "maxTemp"=0, "minTemp"=0, "maxSlope"=0, "thermalprofiles"=[{"thermalsetpoint"=0, "tempgoal"=0, "ramp"=0, "soakduration"=0}]} ("ThermalProfileCluster.profiles"), "zone"=w2244, "average"=w2214, "thermocouples"=w2231, "maxTemp"=w2221, "minTemp"=w2220, "maxSlope"=w2216, "thermalprofiles"=w2226) -> (w2211:T18)
              n1184 = local write "profilearray"(dbl[][] []) -> ()
              n1185 = Build Array (concatenate)(w2213, w2211) -> (w2212:T28)
            }
          }
        }
        n1186 = control-ref of="Thermal Profile Name"() -> (w2094:refnum<vi>)
        n1187 = case shown="True" "TVAC Labview" {
          tunnel: [path "C:/ProgramData/Anaconda3/python.exe" ("Path to Python.exe") path "C:/Users/TVAC-admin/AppData/Local/Programs/Python/Python35/python.exe" ("Path to Python.exe")] -> w2096
          frame False {
          }
          frame True {
          }
        }
        n1188 = Delete From Array(array=w2116, index=0) -> (array with subset deleted=w2114:T28)  [unwired: 1 in, 1 out]
        n1189 = property on="Property Node" class="Str"(reference=w2094) -> ("Text.Text"=w2084:string)  [unwired: 1 in, 2 out]
        n1190 = Bundle By Name(cluster=w2091, "ZoneProfile.profiles"=w2114, "ZoneSetup.Thermal Profile Name"=w2084) -> (w2121:T13)
        n1191 = Flatten To JSON(anything=w2114, error in (no error)=w2113) -> (JSON string=w2110:string, 11:w2112:errorcluster)  [unwired: 1 in]
        n1192 = Unbundle By Name(w2091) -> ("ZonesSelected"=w2090:bool[])
        n1193 = case shown="True" "TVAC Labview" {
          tunnel: [path "C:/Users/stefan/Documents/GitHub/TVAC/head/Labview2017/TVAC_GUI/TestScripts/graph.json" ("file path (use dialog)") path "C:/Users/TVAC-admin/Documents/TVAC_Github/head/Labview2017/TVAC_GUI/TestScripts/graph.json" ("file path (use dialog)")] -> w2108
          frame False {
          }
          frame True {
          }
        }
        n1194 = Open/Create/Replace File(file path (use dialog)=w2108, error in=w2112, operation (0:open)=T17."replace or create") -> (refnum out=w2111:refnum<file>, error out=w2109:errorcluster)  [unwired: 3 in, 1 out]
        n1195 = Write to Text File(file (use dialog)=w2111, text=w2110, error in=w2109) -> (refnum out=w2106:refnum<file>, error out=w2107:errorcluster)  [unwired: 1 in, 1 out]
        n1196 = call "Calling Python Script.vi"("error in (no error)"=w2107, "Path to Python.exe"=w2096, "pathToJson"=w2108) -> ("error out"=w2097:errorcluster, "graphCluster"=w2092:T31)  [unwired: 1 in]
        n1197 = Unbundle By Name(w2092) -> ("time"=w2089:dbl[])
        n1198 = Close File(refnum=w2106, error in=w2107) -> ()  [unwired: 2 out]
        n1199 = Concatenate Strings("Thermal Profile : ", w2084) -> (w2083:string)
        n1200 = for {
          N: 9 -> [_]
          tunnel: w2092 -> [w2127]
          tunnel: w2090 -> [_] mode=indexing
          shift-right: [w2128] -> w2088
          shift-left: w2089 -> [w2128]
          tunnel: w2083 -> [w2125]
          i -> [w2126]
          n1201 = case shown="8" w2126 {
            tunnel: w2127 -> [w2132 w2139 w2146 w2153 w2160 w2167 w2174 w2181 w2189]
            tunnel: w2125 -> [_ _ _ _ _ _ _ _ w2185]
            frame 0, Default {
              n1202 = Unbundle By Name(w2132) -> ("zone1"=w2131:dbl[])
              n1203 = Index Array(array=w2131) -> (element=w2129:dbl)  [unwired: 1 in]
              n1204 = Not Equal To 0?(x=w2129) -> (x != 0?=w2130:bool)
              n1205 = case shown="True" w2130 {
                tunnel: w2131 -> [_ w2134]
                frame False {
                }
                frame True {
                  n1206 = local read "profilearray"() -> (w2135:dbl[][])
                  n1207 = Build Array (concatenate)(w2135, w2134) -> (w2133:dbl[][])
                  n1208 = local write "profilearray"(w2133) -> ()
                }
              }
            }
            frame 1 {
              n1209 = Unbundle By Name(w2139) -> ("zone2"=w2138:dbl[])
              n1210 = Index Array(array=w2138) -> (element=w2136:dbl)  [unwired: 1 in]
              n1211 = Not Equal To 0?(x=w2136) -> (x != 0?=w2137:bool)
              n1212 = case shown="True" w2137 {
                tunnel: w2138 -> [_ w2141]
                frame False {
                }
                frame True {
                  n1213 = local read "profilearray"() -> (w2142:dbl[][])
                  n1214 = Build Array (concatenate)(w2142, w2141) -> (w2140:dbl[][])
                  n1215 = local write "profilearray"(w2140) -> ()
                }
              }
            }
            frame 2 {
              n1216 = Unbundle By Name(w2146) -> ("zone3"=w2145:dbl[])
              n1217 = Index Array(array=w2145) -> (element=w2143:dbl)  [unwired: 1 in]
              n1218 = Not Equal To 0?(x=w2143) -> (x != 0?=w2144:bool)
              n1219 = case shown="True" w2144 {
                tunnel: w2145 -> [_ w2148]
                frame False {
                }
                frame True {
                  n1220 = local read "profilearray"() -> (w2149:dbl[][])
                  n1221 = Build Array (concatenate)(w2149, w2148) -> (w2147:dbl[][])
                  n1222 = local write "profilearray"(w2147) -> ()
                }
              }
            }
            frame 3 {
              n1223 = Unbundle By Name(w2153) -> ("zone4"=w2152:dbl[])
              n1224 = Index Array(array=w2152) -> (element=w2150:dbl)  [unwired: 1 in]
              n1225 = Not Equal To 0?(x=w2150) -> (x != 0?=w2151:bool)
              n1226 = case shown="True" w2151 {
                tunnel: w2152 -> [_ w2155]
                frame False {
                }
                frame True {
                  n1227 = local read "profilearray"() -> (w2156:dbl[][])
                  n1228 = Build Array (concatenate)(w2156, w2155) -> (w2154:dbl[][])
                  n1229 = local write "profilearray"(w2154) -> ()
                }
              }
            }
            frame 4 {
              n1230 = Unbundle By Name(w2160) -> ("zone5"=w2159:dbl[])
              n1231 = Index Array(array=w2159) -> (element=w2157:dbl)  [unwired: 1 in]
              n1232 = Not Equal To 0?(x=w2157) -> (x != 0?=w2158:bool)
              n1233 = case shown="True" w2158 {
                tunnel: w2159 -> [_ w2162]
                frame False {
                }
                frame True {
                  n1234 = local read "profilearray"() -> (w2163:dbl[][])
                  n1235 = Build Array (concatenate)(w2163, w2162) -> (w2161:dbl[][])
                  n1236 = local write "profilearray"(w2161) -> ()
                }
              }
            }
            frame 5 {
              n1237 = Unbundle By Name(w2167) -> ("zone6"=w2166:dbl[])
              n1238 = Index Array(array=w2166) -> (element=w2164:dbl)  [unwired: 1 in]
              n1239 = Not Equal To 0?(x=w2164) -> (x != 0?=w2165:bool)
              n1240 = case shown="True" w2165 {
                tunnel: w2166 -> [_ w2169]
                frame False {
                }
                frame True {
                  n1241 = local read "profilearray"() -> (w2170:dbl[][])
                  n1242 = Build Array (concatenate)(w2170, w2169) -> (w2168:dbl[][])
                  n1243 = local write "profilearray"(w2168) -> ()
                }
              }
            }
            frame 6 {
              n1244 = Unbundle By Name(w2174) -> ("zone7"=w2173:dbl[])
              n1245 = Index Array(array=w2173) -> (element=w2171:dbl)  [unwired: 1 in]
              n1246 = Not Equal To 0?(x=w2171) -> (x != 0?=w2172:bool)
              n1247 = case shown="True" w2172 {
                tunnel: w2173 -> [_ w2176]
                frame False {
                }
                frame True {
                  n1248 = local read "profilearray"() -> (w2177:dbl[][])
                  n1249 = Build Array (concatenate)(w2177, w2176) -> (w2175:dbl[][])
                  n1250 = local write "profilearray"(w2175) -> ()
                }
              }
            }
            frame 7 {
              n1251 = Unbundle By Name(w2181) -> ("zone8"=w2180:dbl[])
              n1252 = Index Array(array=w2180) -> (element=w2178:dbl)  [unwired: 1 in]
              n1253 = Not Equal To 0?(x=w2178) -> (x != 0?=w2179:bool)
              n1254 = case shown="True" w2179 {
                tunnel: w2180 -> [_ w2183]
                frame False {
                }
                frame True {
                  n1255 = local read "profilearray"() -> (w2184:dbl[][])
                  n1256 = Build Array (concatenate)(w2184, w2183) -> (w2182:dbl[][])
                  n1257 = local write "profilearray"(w2182) -> ()
                }
              }
            }
            frame 8 {
              n1258 = Unbundle By Name(w2189) -> ("zone9"=w2188:dbl[])
              n1259 = Index Array(array=w2188) -> (element=w2186:dbl)  [unwired: 1 in]
              n1260 = Not Equal To 0?(x=w2186) -> (x != 0?=w2187:bool)
              n1261 = case shown="True" w2187 {
                tunnel: w2188 -> [_ w2191]
                frame False {
                }
                frame True {
                  n1262 = local read "profilearray"() -> (w2192:dbl[][])
                  n1263 = Build Array (concatenate)(w2192, w2191) -> (w2190:dbl[][])
                  n1264 = local write "profilearray"(w2190) -> ()
                }
              }
              "ThermalProfileStatus" <- w2185
            }
          }
        }
        n1265 = Index Array(array=w2088, index=1) -> (element=w2087:dbl)
        n1266 = Index Array(array=w2088, index=0) -> (element=w2098:dbl)
        n1267 = Subtract(x=w2087, y=w2098) -> (x-y=w2103:dbl)
        n1268 = local read "profilearray"() -> (w2086:dbl[][])
        n1269 = Divide(x=w2103, y=60.0) -> (x/y=w2101:dbl)
        n1270 = Bundle(0.0, w2101, "profilearray"=w2086) -> (→"Thermal Profile":cluster{dbl, dbl, "profilearray":dbl[][]})  [unwired: 1 in]
      }
      frame "importProfile" {
        n1271 = property on="Path" class="Path"() -> ("Text.Text"=w2360:string)  [unwired: 2 in, 2 out]
        n1272 = call-poly <vilib>:"Read Delimited Spreadsheet.vi"("file path (dialog if empty)"="Path", "delimiter (\\t)"="," ("delimiter (\\t)")) -> ("all rows"=w2344:string[][])  [unwired: 8 in, 5 out]
        n1273 = Array Size(array=w2344) -> (size(s)=w2364:i32[])
        n1274 = Index Array(array=w2364, index=0) -> (element=w2345:i32)
        n1275 = Spreadsheet String To Array(delimiter (Tab)="\\", format string="%s", spreadsheet string=w2360, array type (2D Dbl)=string[][] []) -> (array=w2355:string[][])
        n1276 = for {
          N: w2345 -> [_]
          shift-right: [w2400] -> w2343
          shift-left: w2344 -> [w2401]
          shift-right: [w2392] -> w2340
          shift-left: "LastSetPt" -> [w2391]
          i -> [w2396]
          n1277 = Add(x=7 ("y"), y=w2396) -> (x+y=w2395:i32)
          n1278 = Subtract(x=w2395, y=6) -> (x-y=w2393:i32)
          n1279 = Index Array(array=w2401, index (row)=w2395, index (col)=0 ("disabled index (col)")) -> (element=w2402:string)
          n1280 = Number To Decimal String(number=w2393) -> (decimal integer string=w2394:string)  [unwired: 1 in]
          n1281 = Equal?(x=w2402, y=w2394) -> (x = y?=w2399:bool)
          n1282 = case shown="True" w2399 {
            tunnel: w2401 -> [w2405 w2407]
            tunnel: [w2405 w2407] -> w2400
            tunnel: w2393 -> [_ w2406]
            tunnel: [w2404 w2406] -> w2392
            tunnel: w2391 -> [w2404 _]
            frame False {
            }
            frame True {
              n1283 = local write "LastSetPt"(w2406) -> ()
            }
          }
        }
        n1284 = Array Size(array=w2355) -> (size(s)=w2354:i32[])
        n1285 = Bundle By Name(cluster=w2346, "tprofilesheet"=w2344) -> (w2370:T13)
        n1286 = local write "tprofilesheet"(w2344) -> ()
        n1287 = Index Array(array=w2344, index (row)=1) -> (element=w2371:string[])  [unwired: 1 in]
        n1288 = Index Array(array=w2344, index (row)=2) -> (element=w2367:string[])  [unwired: 1 in]
        n1289 = Index Array(array=w2354, index=1) -> (element=w2352:i32)
        n1290 = Decrement(x=w2352) -> (x-1=w2351:i32)
        n1291 = Index Array(array=w2355, index (row)=0, index (col)=w2351) -> (element=w2350:string)
        n1292 = Match Pattern(string=w2350, regular expression=".csv") -> (before substring=w2347:string)  [unwired: 1 in, 3 out]
        n1293 = Unbundle By Name(w2370) -> ("ZoneSetup.Zone Selection"=w2369:i32[])
        n1294 = To Double Precision Float(number=w2340) -> (double precision float=w2361:dbl)
        n1295 = for {
          N: 9 -> [_]
          shift-right: [w2435] -> w2368
          shift-left: w2370 -> [w2449]
          tunnel: w2371 -> [w2448] mode=indexing
          shift-right: [w2446] -> w2365
          shift-left: w2369 -> [w2447]
          tunnel: w2367 -> [w2440]
          tunnel: w2343 -> [w2419]
          tunnel: w2340 -> [w2409]
          i -> [w2415]
          n1296 = case shown="6" w2415 {
            selector: w2415 -> [w2539 w2574 w2609 w2644 w2679 w2714 w2749 w2784 w2819]
            tunnel: w2449 -> [w2543 w2578 w2613 w2648 w2683 w2718 w2753 w2788 w2823]
            tunnel: [w2542 w2577 w2612 w2647 w2682 w2717 w2752 w2787 w2822] -> w2436
            tunnel: w2448 -> [w2541 w2576 w2611 w2646 w2681 w2716 w2751 w2786 w2821]
            tunnel: w2447 -> [w2540 w2575 w2610 w2645 w2680 w2715 w2750 w2785 w2820]
            tunnel: [w2538 w2573 w2608 w2643 w2678 w2713 w2748 w2783 w2818] -> w2446
            tunnel: [w2537 w2572 w2607 w2642 w2677 w2712 w2747 w2782 w2817] -> w2437
            tunnel: [w2536 w2571 w2606 w2641 w2676 w2711 w2746 w2781 w2816] -> w2432
            tunnel: [w2533 w2568 w2603 w2638 w2673 w2708 w2743 w2778 w2813] -> w2433
            tunnel: [w2531 w2566 w2601 w2636 w2671 w2706 w2741 w2776 w2811] -> w2411
            tunnel: [w2530 w2565 w2600 w2635 w2670 w2705 w2740 w2775 w2810] -> w2420
            tunnel: [w2529 w2564 w2599 w2634 w2669 w2704 w2739 w2774 w2809] -> w2410
            frame 0, Default {
              n1297 = control-ref of="Thermocouples Selected"() -> (w2533:refnum<vi>)
              n1298 = case shown="\"Min\"" w2541 {
                tunnel: [2 1 0 0] -> w2534
                tunnel: w2540 -> [w2547 w2552 w2557 w2562]
                tunnel: w2539 -> [w2546 w2551 w2556 w2561]
                tunnel: [w2545 w2550 w2555 w2560] -> w2538
                frame "Max" {
                  n1299 = Replace Array Subset(array=w2547, new element=38, index=w2546) -> (w2545:i32[])
                }
                frame "Min" {
                  n1300 = Replace Array Subset(array=w2552, new element=38, index=w2551) -> (w2550:i32[])
                }
                frame "Average" {
                  n1301 = Replace Array Subset(array=w2557, new element=38, index=w2556) -> (w2555:i32[])
                }
                frame "", Default {
                  n1302 = Replace Array Subset(array=w2562, new element=37, index=w2561) -> (w2560:i32[])
                }
              }
              n1303 = control-ref of="Max Temp Slope"() -> (w2531:refnum<vi>)
              n1304 = property class="Str"(reference=w2533, "Text.Text"="") -> ()  [unwired: 1 in, 2 out]
              n1305 = control-ref of="Min Allowable Temp"() -> (w2530:refnum<vi>)
              n1306 = control-ref of="Zone Thermocouples"() -> (w2536:refnum<vi>)
              n1307 = property class="LstBox (strict)"(reference=w2536) -> ("Item Symbols"=w2537:i32[])  [unwired: 1 in, 2 out]
              n1308 = control-ref of="Max Allowable Temp"() -> (w2529:refnum<vi>)
              n1309 = Bundle By Name(cluster=w2543, "Zone 1.Temperature Calculation"=w2534) -> (w2542:T13)
              n1310 = control-ref of="Temperature Calculation"() -> (w2535:refnum<vi>)
              n1311 = property class="Ring (strict)"(reference=w2535, "Value"=w2534) -> ()  [unwired: 1 in, 2 out]
            }
            frame 1 {
              n1312 = control-ref of="Thermocouples Selected"() -> (w2568:refnum<vi>)
              n1313 = case shown="\"Min\"" w2576 {
                tunnel: [2 1 0 0] -> w2569
                tunnel: w2575 -> [w2582 w2587 w2592 w2597]
                tunnel: w2574 -> [w2581 w2586 w2591 w2596]
                tunnel: [w2580 w2585 w2590 w2595] -> w2573
                frame "Max" {
                  n1314 = Replace Array Subset(array=w2582, new element=38, index=w2581) -> (w2580:i32[])
                }
                frame "Min" {
                  n1315 = Replace Array Subset(array=w2587, new element=38, index=w2586) -> (w2585:i32[])
                }
                frame "Average" {
                  n1316 = Replace Array Subset(array=w2592, new element=38, index=w2591) -> (w2590:i32[])
                }
                frame "", Default {
                  n1317 = Replace Array Subset(array=w2597, new element=37, index=w2596) -> (w2595:i32[])
                }
              }
              n1318 = control-ref of="Max Temp Slope"() -> (w2566:refnum<vi>)
              n1319 = property class="Str"(reference=w2568, "Text.Text"="") -> ()  [unwired: 1 in, 2 out]
              n1320 = control-ref of="Min Allowable Temp"() -> (w2565:refnum<vi>)
              n1321 = control-ref of="Zone Thermocouples"() -> (w2571:refnum<vi>)
              n1322 = property class="LstBox (strict)"(reference=w2571) -> ("Item Symbols"=w2572:i32[])  [unwired: 1 in, 2 out]
              n1323 = control-ref of="Max Allowable Temp"() -> (w2564:refnum<vi>)
              n1324 = Bundle By Name(cluster=w2578, "Zone 2.Temperature Calculation"=w2569) -> (w2577:T13)
              n1325 = control-ref of="Temperature Calculation"() -> (w2570:refnum<vi>)
              n1326 = property class="Ring (strict)"(reference=w2570, "Value"=w2569) -> ()  [unwired: 1 in, 2 out]
            }
            frame 2 {
              n1327 = control-ref of="Thermocouples Selected"() -> (w2603:refnum<vi>)
              n1328 = case shown="\"Min\"" w2611 {
                tunnel: [2 1 0 0] -> w2604
                tunnel: w2610 -> [w2617 w2622 w2627 w2632]
                tunnel: w2609 -> [w2616 w2621 w2626 w2631]
                tunnel: [w2615 w2620 w2625 w2630] -> w2608
                frame "Max" {
                  n1329 = Replace Array Subset(array=w2617, new element=38, index=w2616) -> (w2615:i32[])
                }
                frame "Min" {
                  n1330 = Replace Array Subset(array=w2622, new element=38, index=w2621) -> (w2620:i32[])
                }
                frame "Average" {
                  n1331 = Replace Array Subset(array=w2627, new element=38, index=w2626) -> (w2625:i32[])
                }
                frame "", Default {
                  n1332 = Replace Array Subset(array=w2632, new element=37, index=w2631) -> (w2630:i32[])
                }
              }
              n1333 = control-ref of="Max Temp Slope"() -> (w2601:refnum<vi>)
              n1334 = property class="Str"(reference=w2603, "Text.Text"="") -> ()  [unwired: 1 in, 2 out]
              n1335 = control-ref of="Min Allowable Temp"() -> (w2600:refnum<vi>)
              n1336 = control-ref of="Zone Thermocouples"() -> (w2606:refnum<vi>)
              n1337 = property class="LstBox (strict)"(reference=w2606) -> ("Item Symbols"=w2607:i32[])  [unwired: 1 in, 2 out]
              n1338 = control-ref of="Max Allowable Temp"() -> (w2599:refnum<vi>)
              n1339 = Bundle By Name(cluster=w2613, "Zone 3.Temperature Calculation"=w2604) -> (w2612:T13)
              n1340 = control-ref of="Temperature Calculation"() -> (w2605:refnum<vi>)
              n1341 = property class="Ring (strict)"(reference=w2605, "Value"=w2604) -> ()  [unwired: 1 in, 2 out]
            }
            frame 3 {
              n1342 = control-ref of="Thermocouples Selected"() -> (w2638:refnum<vi>)
              n1343 = case shown="\"Min\"" w2646 {
                tunnel: [2 1 0 0] -> w2639
                tunnel: w2645 -> [w2652 w2657 w2662 w2667]
                tunnel: w2644 -> [w2651 w2656 w2661 w2666]
                tunnel: [w2650 w2655 w2660 w2665] -> w2643
                frame "Max" {
                  n1344 = Replace Array Subset(array=w2652, new element=38, index=w2651) -> (w2650:i32[])
                }
                frame "Min" {
                  n1345 = Replace Array Subset(array=w2657, new element=38, index=w2656) -> (w2655:i32[])
                }
                frame "Average" {
                  n1346 = Replace Array Subset(array=w2662, new element=38, index=w2661) -> (w2660:i32[])
                }
                frame "", Default {
                  n1347 = Replace Array Subset(array=w2667, new element=37, index=w2666) -> (w2665:i32[])
                }
              }
              n1348 = control-ref of="Max Temp Slope"() -> (w2636:refnum<vi>)
              n1349 = property class="Str"(reference=w2638, "Text.Text"="") -> ()  [unwired: 1 in, 2 out]
              n1350 = control-ref of="Min Allowable Temp"() -> (w2635:refnum<vi>)
              n1351 = control-ref of="Zone Thermocouples"() -> (w2641:refnum<vi>)
              n1352 = property class="LstBox (strict)"(reference=w2641) -> ("Item Symbols"=w2642:i32[])  [unwired: 1 in, 2 out]
              n1353 = control-ref of="Max Allowable Temp"() -> (w2634:refnum<vi>)
              n1354 = Bundle By Name(cluster=w2648, "Zone 4.Temperature Calculation"=w2639) -> (w2647:T13)
              n1355 = control-ref of="Temperature Calculation"() -> (w2640:refnum<vi>)
              n1356 = property class="Ring (strict)"(reference=w2640, "Value"=w2639) -> ()  [unwired: 1 in, 2 out]
            }
            frame 4 {
              n1357 = control-ref of="Thermocouples Selected"() -> (w2673:refnum<vi>)
              n1358 = case shown="\"Min\"" w2681 {
                tunnel: [2 1 0 0] -> w2674
                tunnel: w2680 -> [w2687 w2692 w2697 w2702]
                tunnel: w2679 -> [w2686 w2691 w2696 w2701]
                tunnel: [w2685 w2690 w2695 w2700] -> w2678
                frame "Max" {
                  n1359 = Replace Array Subset(array=w2687, new element=38, index=w2686) -> (w2685:i32[])
                }
                frame "Min" {
                  n1360 = Replace Array Subset(array=w2692, new element=38, index=w2691) -> (w2690:i32[])
                }
                frame "Average" {
                  n1361 = Replace Array Subset(array=w2697, new element=38, index=w2696) -> (w2695:i32[])
                }
                frame "", Default {
                  n1362 = Replace Array Subset(array=w2702, new element=37, index=w2701) -> (w2700:i32[])
                }
              }
              n1363 = control-ref of="Max Temp Slope"() -> (w2671:refnum<vi>)
              n1364 = property class="Str"(reference=w2673, "Text.Text"="") -> ()  [unwired: 1 in, 2 out]
              n1365 = control-ref of="Min Allowable Temp"() -> (w2670:refnum<vi>)
              n1366 = control-ref of="Zone Thermocouples"() -> (w2676:refnum<vi>)
              n1367 = property class="LstBox (strict)"(reference=w2676) -> ("Item Symbols"=w2677:i32[])  [unwired: 1 in, 2 out]
              n1368 = control-ref of="Max Allowable Temp"() -> (w2669:refnum<vi>)
              n1369 = Bundle By Name(cluster=w2683, "Zone 5.Temperature Calculation"=w2674) -> (w2682:T13)
              n1370 = control-ref of="Temperature Calculation"() -> (w2675:refnum<vi>)
              n1371 = property class="Ring (strict)"(reference=w2675, "Value"=w2674) -> ()  [unwired: 1 in, 2 out]
            }
            frame 5 {
              n1372 = control-ref of="Thermocouples Selected"() -> (w2708:refnum<vi>)
              n1373 = case shown="\"Min\"" w2716 {
                tunnel: [2 1 0 0] -> w2709
                tunnel: w2715 -> [w2722 w2727 w2732 w2737]
                tunnel: w2714 -> [w2721 w2726 w2731 w2736]
                tunnel: [w2720 w2725 w2730 w2735] -> w2713
                frame "Max" {
                  n1374 = Replace Array Subset(array=w2722, new element=38, index=w2721) -> (w2720:i32[])
                }
                frame "Min" {
                  n1375 = Replace Array Subset(array=w2727, new element=38, index=w2726) -> (w2725:i32[])
                }
                frame "Average" {
                  n1376 = Replace Array Subset(array=w2732, new element=38, index=w2731) -> (w2730:i32[])
                }
                frame "", Default {
                  n1377 = Replace Array Subset(array=w2737, new element=37, index=w2736) -> (w2735:i32[])
                }
              }
              n1378 = control-ref of="Max Temp Slope"() -> (w2706:refnum<vi>)
              n1379 = property class="Str"(reference=w2708, "Text.Text"="") -> ()  [unwired: 1 in, 2 out]
              n1380 = control-ref of="Min Allowable Temp"() -> (w2705:refnum<vi>)
              n1381 = control-ref of="Zone Thermocouples"() -> (w2711:refnum<vi>)
              n1382 = property class="LstBox (strict)"(reference=w2711) -> ("Item Symbols"=w2712:i32[])  [unwired: 1 in, 2 out]
              n1383 = control-ref of="Max Allowable Temp"() -> (w2704:refnum<vi>)
              n1384 = Bundle By Name(cluster=w2718, "Zone 6.Temperature Calculation"=w2709) -> (w2717:T13)
              n1385 = control-ref of="Temperature Calculation"() -> (w2710:refnum<vi>)
              n1386 = property class="Ring (strict)"(reference=w2710, "Value"=w2709) -> ()  [unwired: 1 in, 2 out]
            }
            frame 6 {
              n1387 = control-ref of="Thermocouples Selected"() -> (w2743:refnum<vi>)
              n1388 = case shown="\"Average\"" w2751 {
                tunnel: [2 1 0 0] -> w2744
                tunnel: w2750 -> [w2757 w2762 w2767 w2772]
                tunnel: w2749 -> [w2756 w2761 w2766 w2771]
                tunnel: [w2755 w2760 w2765 w2770] -> w2748
                frame "Max" {
                  n1389 = Replace Array Subset(array=w2757, new element=38, index=w2756) -> (w2755:i32[])
                }
                frame "Min" {
                  n1390 = Replace Array Subset(array=w2762, new element=38, index=w2761) -> (w2760:i32[])
                }
                frame "Average" {
                  n1391 = Replace Array Subset(array=w2767, new element=38, index=w2766) -> (w2765:i32[])
                }
                frame "", Default {
                  n1392 = Replace Array Subset(array=w2772, new element=37, index=w2771) -> (w2770:i32[])
                }
              }
              n1393 = control-ref of="Max Temp Slope"() -> (w2741:refnum<vi>)
              n1394 = property class="Str"(reference=w2743, "Text.Text"="") -> ()  [unwired: 1 in, 2 out]
              n1395 = control-ref of="Min Allowable Temp"() -> (w2740:refnum<vi>)
              n1396 = control-ref of="Zone Thermocouples"() -> (w2746:refnum<vi>)
              n1397 = property class="LstBox (strict)"(reference=w2746) -> ("Item Symbols"=w2747:i32[])  [unwired: 1 in, 2 out]
              n1398 = control-ref of="Max Allowable Temp"() -> (w2739:refnum<vi>)
              n1399 = Bundle By Name(cluster=w2753, "Zone 7.Temperature Calculation"=w2744) -> (w2752:T13)
              n1400 = control-ref of="Temperature Calculation"() -> (w2745:refnum<vi>)
              n1401 = property class="Ring (strict)"(reference=w2745, "Value"=w2744) -> ()  [unwired: 1 in, 2 out]
            }
            frame 7 {
              n1402 = control-ref of="Thermocouples Selected"() -> (w2778:refnum<vi>)
              n1403 = case shown="\"Min\"" w2786 {
                tunnel: [2 1 0 0] -> w2779
                tunnel: w2785 -> [w2792 w2797 w2802 w2807]
                tunnel: w2784 -> [w2791 w2796 w2801 w2806]
                tunnel: [w2790 w2795 w2800 w2805] -> w2783
                frame "Max" {
                  n1404 = Replace Array Subset(array=w2792, new element=38, index=w2791) -> (w2790:i32[])
                }
                frame "Min" {
                  n1405 = Replace Array Subset(array=w2797, new element=38, index=w2796) -> (w2795:i32[])
                }
                frame "Average" {
                  n1406 = Replace Array Subset(array=w2802, new element=38, index=w2801) -> (w2800:i32[])
                }
                frame "", Default {
                  n1407 = Replace Array Subset(array=w2807, new element=37, index=w2806) -> (w2805:i32[])
                }
              }
              n1408 = control-ref of="Max Temp Slope"() -> (w2776:refnum<vi>)
              n1409 = property class="Str"(reference=w2778, "Text.Text"="") -> ()  [unwired: 1 in, 2 out]
              n1410 = control-ref of="Min Allowable Temp"() -> (w2775:refnum<vi>)
              n1411 = control-ref of="Zone Thermocouples"() -> (w2781:refnum<vi>)
              n1412 = property class="LstBox (strict)"(reference=w2781) -> ("Item Symbols"=w2782:i32[])  [unwired: 1 in, 2 out]
              n1413 = control-ref of="Max Allowable Temp"() -> (w2774:refnum<vi>)
              n1414 = Bundle By Name(cluster=w2788, "Zone 8.Temperature Calculation"=w2779) -> (w2787:T13)
              n1415 = control-ref of="Temperature Calculation"() -> (w2780:refnum<vi>)
              n1416 = property class="Ring (strict)"(reference=w2780, "Value"=w2779) -> ()  [unwired: 1 in, 2 out]
            }
            frame 8 {
              n1417 = control-ref of="Thermocouples Selected"() -> (w2813:refnum<vi>)
              n1418 = case shown="\"Min\"" w2821 {
                tunnel: [2 1 0 0] -> w2814
                tunnel: w2820 -> [w2827 w2832 w2837 w2842]
                tunnel: w2819 -> [w2826 w2831 w2836 w2841]
                tunnel: [w2825 w2830 w2835 w2840] -> w2818
                frame "Max" {
                  n1419 = Replace Array Subset(array=w2827, new element=38, index=w2826) -> (w2825:i32[])
                }
                frame "Min" {
                  n1420 = Replace Array Subset(array=w2832, new element=38, index=w2831) -> (w2830:i32[])
                }
                frame "Average" {
                  n1421 = Replace Array Subset(array=w2837, new element=38, index=w2836) -> (w2835:i32[])
                }
                frame "", Default {
                  n1422 = Replace Array Subset(array=w2842, new element=37, index=w2841) -> (w2840:i32[])
                }
              }
              n1423 = control-ref of="Max Temp Slope"() -> (w2811:refnum<vi>)
              n1424 = property class="Str"(reference=w2813, "Text.Text"="") -> ()  [unwired: 1 in, 2 out]
              n1425 = control-ref of="Min Allowable Temp"() -> (w2810:refnum<vi>)
              n1426 = control-ref of="Zone Thermocouples"() -> (w2816:refnum<vi>)
              n1427 = property class="LstBox (strict)"(reference=w2816) -> ("Item Symbols"=w2817:i32[])  [unwired: 1 in, 2 out]
              n1428 = control-ref of="Max Allowable Temp"() -> (w2809:refnum<vi>)
              n1429 = Bundle By Name(cluster=w2823, "Zone 9.Temperature Calculation"=w2814) -> (w2822:T13)
              n1430 = control-ref of="Temperature Calculation"() -> (w2815:refnum<vi>)
              n1431 = property class="Ring (strict)"(reference=w2815, "Value"=w2814) -> ()  [unwired: 1 in, 2 out]
            }
          }
          n1432 = Index Array(array=w2440, index=w2415) -> (element=w2443:string)
          n1433 = call <vilib>:"Space Constant.vi"() -> ("String"=w2444:string)
          n1434 = Initialize Array("", w2409, 3 ("dimension size")) -> (w2424:string[][])
          n1435 = Spreadsheet String To Array(delimiter (Tab)=w2444, format string="%d", spreadsheet string=w2443) -> (array=w2445:dbl[][])  [unwired: 1 in]
          n1436 = Initialize Array("", w2409, 2 ("dimension size")) -> (w2431:string[][])
          n1437 = Index Array(array=w2445, index (row)=0) -> (element=w2439:dbl[])  [unwired: 1 in]
          n1438 = To Long Integer(number=w2439) -> (32bit integer=w2438:i32[])
          n1439 = Array Size(array=w2438) -> (size(s)=w2408:i32)
          n1440 = for {
            N: w2409 -> [_]
            tunnel: w2419 -> [w2471]
            shift-right: [w2468] -> w2428
            shift-left: w2431 -> [w2469]
            tunnel: w2415 -> [w2463]
            shift-right: [w2452] -> w2423
            shift-left: w2424 -> [w2453]
            i -> [w2455]
            n1441 = Add(x=3, y=w2463) -> (x+y=w2462:i32)
            n1442 = Add(x=7, y=w2455) -> (x+y=w2461:i32)
            n1443 = Index Array(array=w2471, index (row) #1=w2461, index (col) #1=0 ("disabled index (col)"), index (row) #2=w2461, index (col) #2=w2462, index (row) #3=w2461, index (col) #3=1 ("disabled index (col)"), index (row) #4=w2461, index (col) #4=2 ("disabled index (col)")) -> (element #1=w2458:string, element #2=w2466:string, element #3=w2457:string, element #4=w2456:string)
            n1444 = Build Array(w2458, w2466) -> (w2465:string[])
            n1445 = Build Array(w2458, w2457, w2456) -> (w2454:string[])
            n1446 = Replace Array Subset(array=w2469, new element=w2465, index (row)=w2455) -> (w2468:string[][])  [unwired: 1 in]
            n1447 = Replace Array Subset(array=w2453, new element=w2454, index (row)=w2455) -> (w2452:string[][])  [unwired: 1 in]
          }
          n1448 = for {
            N: w2408 -> [_]
            tunnel: w2438 -> [w2517] mode=indexing
            shift-right: [w2521] -> w2434
            shift-left: w2437 -> [w2522]
            tunnel: w2433 -> [w2519]
            n1449 = Not Equal To 0?(x=w2517) -> (x != 0?=w2518:bool)
            n1450 = case shown="True" w2518 {
              tunnel: w2517 -> [_ w2524]
              tunnel: w2519 -> [_ w2523]
              frame False {
              }
              frame True {
                n1451 = property class="Str"(reference=w2523) -> ("Text.Text"=w2528:string)  [unwired: 1 in, 2 out]
                n1452 = Number To Decimal String(number=w2524) -> (decimal integer string=w2525:string)  [unwired: 1 in]
                n1453 = call <vilib>:"Space Constant.vi"() -> ("String"=w2526:string)
                n1454 = Concatenate Strings(w2528, w2526, w2525) -> (w2527:string)
                n1455 = property class="Str"(reference=w2523, "Text.Text"=w2527) -> ()  [unwired: 1 in, 2 out]
              }
            }
            n1456 = Replace Array Subset(array=w2522, new element=38, index=w2517) -> (w2521:i32[])
          }
          n1457 = property class="LstBox (strict)"(reference=w2432, "Item Symbols"=w2434) -> ()  [unwired: 1 in, 2 out]
          n1458 = Fract/Exp String To Number(string=w2423) -> (number=w2421:dbl[][])  [unwired: 3 in, 1 out]
          n1459 = Fract/Exp String To Number(string=w2428) -> (number=w2427:dbl[][])  [unwired: 3 in, 1 out]
          n1460 = case shown="0, Default" w2415 {
            tunnel: w2436 -> [w2476 w2481 w2486 w2491 w2496 w2501 w2506 w2511 w2516]
            tunnel: [w2475 w2480 w2485 w2490 w2495 w2500 w2505 w2510 w2515] -> w2435
            tunnel: w2434 -> [w2474 w2479 w2484 w2489 w2494 w2499 w2504 w2509 w2514]
            tunnel: w2427 -> [w2472 w2477 w2482 w2487 w2492 w2497 w2502 w2507 w2512]
            frame 0, Default {
              n1461 = Bundle By Name(cluster=w2476, "Zone 1.Zone Thermocouples"=w2474) -> (w2475:T13)
              n1462 = control-ref of="Temperature Goal"() -> (w2473:refnum<vi>)
              n1463 = property class="Arr (strict)"(reference=w2473, "Value"=w2472) -> ()  [unwired: 1 in, 2 out]
            }
            frame 1 {
              n1464 = Bundle By Name(cluster=w2481, "Zone 2.Zone Thermocouples"=w2479) -> (w2480:T13)
              n1465 = control-ref of="Temperature Goal"() -> (w2478:refnum<vi>)
              n1466 = property class="Arr (strict)"(reference=w2478, "Value"=w2477) -> ()  [unwired: 1 in, 2 out]
            }
            frame 2 {
              n1467 = Bundle By Name(cluster=w2486, "Zone 3.Zone Thermocouples"=w2484) -> (w2485:T13)
              n1468 = control-ref of="Temperature Goal"() -> (w2483:refnum<vi>)
              n1469 = property class="Arr (strict)"(reference=w2483, "Value"=w2482) -> ()  [unwired: 1 in, 2 out]
            }
            frame 3 {
              n1470 = Bundle By Name(cluster=w2491, "Zone 4.Zone Thermocouples"=w2489) -> (w2490:T13)
              n1471 = control-ref of="Temperature Goal"() -> (w2488:refnum<vi>)
              n1472 = property class="Arr (strict)"(reference=w2488, "Value"=w2487) -> ()  [unwired: 1 in, 2 out]
            }
            frame 4 {
              n1473 = Bundle By Name(cluster=w2496, "Zone 5.Zone Thermocouples"=w2494) -> (w2495:T13)
              n1474 = control-ref of="Temperature Goal"() -> (w2493:refnum<vi>)
              n1475 = property class="Arr (strict)"(reference=w2493, "Value"=w2492) -> ()  [unwired: 1 in, 2 out]
            }
            frame 5 {
              n1476 = Bundle By Name(cluster=w2501, "Zone 6.Zone Thermocouples"=w2499) -> (w2500:T13)
              n1477 = control-ref of="Temperature Goal"() -> (w2498:refnum<vi>)
              n1478 = property class="Arr (strict)"(reference=w2498, "Value"=w2497) -> ()  [unwired: 1 in, 2 out]
            }
            frame 6 {
              n1479 = Bundle By Name(cluster=w2506, "Zone 7.Zone Thermocouples"=w2504) -> (w2505:T13)
              n1480 = control-ref of="Temperature Goal"() -> (w2503:refnum<vi>)
              n1481 = property class="Arr (strict)"(reference=w2503, "Value"=w2502) -> ()  [unwired: 1 in, 2 out]
            }
            frame 7 {
              n1482 = Bundle By Name(cluster=w2511, "Zone 8.Zone Thermocouples"=w2509) -> (w2510:T13)
              n1483 = control-ref of="Temperature Goal"() -> (w2508:refnum<vi>)
              n1484 = property class="Arr (strict)"(reference=w2508, "Value"=w2507) -> ()  [unwired: 1 in, 2 out]
            }
            frame 8 {
              n1485 = Bundle By Name(cluster=w2516, "Zone 9.Zone Thermocouples"=w2514) -> (w2515:T13)
              n1486 = control-ref of="Temperature Goal"() -> (w2513:refnum<vi>)
              n1487 = property class="Arr (strict)"(reference=w2513, "Value"=w2512) -> ()  [unwired: 1 in, 2 out]
            }
          }
          n1488 = Equal To 0?(x=w2415) -> (x = 0?=w2422:bool)
          n1489 = case shown="True" w2422 {
            tunnel: w2421 -> [_ w2450]
            frame False {
            }
            frame True {
              n1490 = control-ref of="RampSoakTimes"() -> (w2451:refnum<vi>)
              n1491 = property class="Arr (strict)"(reference=w2451, "Value"=w2450) -> ()  [unwired: 1 in, 2 out]
            }
          }
          n1492 = Index Array(array=w2419, index (row) #1=3 ("dimension size"), index (col) #1=w2415, index (row) #2=4 ("dimension size"), index (col) #2=w2415, index (row) #3=5 ("dimension size"), index (col) #3=w2415) -> (element #1=w2414:string, element #2=w2413:string, element #3=w2412:string)
          n1493 = property class="Str"(reference=w2410, "Value"=w2414) -> ()  [unwired: 1 in, 2 out]
          n1494 = property class="Str"(reference=w2420, "Value"=w2413) -> ()  [unwired: 1 in, 2 out]
          n1495 = property class="Str"(reference=w2411, "Value"=w2412) -> ()  [unwired: 1 in, 2 out]
        }
        n1496 = control-ref of="Number of Set points"() -> (w2362:refnum<vi>)
        n1497 = control-ref of="Thermal Profile Name"() -> (w2348:refnum<vi>)
        n1498 = control-ref of="Zone Selection"() -> (w2366:refnum<vi>)
        n1499 = Bundle By Name(cluster=w2368, "ZoneSetup.Zone Selection"=w2365, "ZoneSetup.Number of Set points"=w2361, "ZoneSetup.Thermal Profile Name"=w2347) -> (w2333:T13)
        n1500 = property class="Str"(reference=w2348, "Text.Text"=w2347) -> ()  [unwired: 1 in, 2 out]
        n1501 = property class="DigNum (strict)"(reference=w2362, "Value"=w2361) -> ()  [unwired: 1 in, 2 out]
        n1502 = property class="LstBox (strict)"(reference=w2366, "Item Symbols"=w2365) -> ()  [unwired: 1 in, 2 out]
        n1503 = Unbundle By Name(w2333) -> ("ZoneSetup.Zone Selection"=w2337:i32[], "ZonesSelected"=w2335:bool[])
        n1504 = for {
          N: 9 -> [_]
          tunnel: w2337 -> [w2376] mode=indexing
          shift-right: [w2380] -> w2334
          shift-left: w2335 -> [w2382]
          shift-right: [w2379] -> w2330
          shift-left: w2331 -> [w2379]
          i -> [w2381]
          n1505 = Equal?(x=37, y=w2376) -> (x = y?=w2378:bool)
          n1506 = case shown="True" w2378 {
            tunnel: w2382 -> [w2386 w2390]
            tunnel: w2381 -> [w2385 w2389]
            tunnel: [w2383 w2387] -> w2380
            frame False {
              n1507 = Replace Array Subset(array=w2386, new element=TRUE ("new element/subarray"), index=w2385) -> (w2383:bool[])
            }
            frame True {
              n1508 = Replace Array Subset(array=w2390, new element=FALSE ("new element/subarray"), index=w2389) -> (w2387:bool[])
            }
          }
        }
        n1509 = Bundle By Name(cluster=w2333, "ZonesSelected"=w2334) -> (w2332:T13)
        n1510 = call-poly "Send Message.vi"("error in (no error)"=w2330, "event"="compileProfile") -> ("error out"=w2339:errorcluster)  [unwired: 9 in]
      }
      frame "saveProfile" {
        n1511 = Unbundle By Name(w2853) -> ("ZoneSetup.Number of Set points"=w2848:dbl)
        n1512 = Initialize Array("", w2848, 12 ("dimension size")) -> (w2847:string[][])
        n1513 = Build Array (concatenate)(string[][] [["zone1", "zone2", "zone3", "zone4", "zone5", "zone6", "zone7", "zone8", "zone9", "", "", ""], ["", "", "", "", "", "", "", "", "", "", "", ""], ["", "", "", "", "", "", "", "", "", "", "", ""], ["", "", "", "", "", "", "", "", "", "", "", ""], ["", "", "", "", "", "", "", "", "", "", "", ""], ["", "", "", "", "", "", "", "", "", "", "", ""], ["setpt", "ramptime", "soaktime", "zone1", "zone2", "zone3", "zone4", "zone5", "zone6", "zone7", "zone8", "zone9"]], w2847) -> (w2846:string[][])
        n1514 = for {
          N: 9 -> [_]
          shift-right: [w2877] -> w2852
          shift-left: w2853 -> [w2877]
          tunnel: w2848 -> [w2857]
          shift-right: [w2869] -> w2845
          shift-left: w2846 -> [w2873]
          i -> [w2867]
          n1515 = Unbundle By Name(w2877) -> ("ZoneProfile.profiles"=w2872:T28)
          n1516 = Index Array(array=w2872, index=w2867) -> (element=w2871:T18)
          n1517 = Unbundle By Name(w2871) -> ("zone"=w2860:i32, "average"=w2863:string, "thermocouples"=w2868:i32[], "maxTemp"=w2876:i32, "minTemp"=w2875:i32, "maxSlope"=w2874:i32, "thermalprofiles"=w2856:T30)
          n1518 = Subtract(x=w2860, y=1) -> (x-y=w2858:i32)
          n1519 = Equal?(x=w2863, y="") -> (x = y?=w2865:bool)
          n1520 = Equal?(x=w2863, y="0") -> (x = y?=w2862:bool)
          n1521 = Or(x=w2865, y=w2862) -> (x .or. y?=w2859:bool)
          n1522 = case shown="False" w2859 {
            tunnel: w2863 -> [w2921 _]
            tunnel: w2876 -> [w2917 _]
            tunnel: w2875 -> [w2912 _]
            tunnel: w2874 -> [w2908 _]
            tunnel: w2873 -> [w2907 w2942]
            tunnel: [w2896 w2942] -> w2870
            tunnel: w2868 -> [w2906 _]
            tunnel: w2858 -> [w2895 _]
            tunnel: w2857 -> [w2899 _]
            tunnel: w2856 -> [w2898 _]
            frame False {
              n1523 = Number To Decimal String(number=w2917) -> (decimal integer string=w2916:string)  [unwired: 1 in]
              n1524 = Number To Decimal String(number=w2912) -> (decimal integer string=w2915:string)  [unwired: 1 in]
              n1525 = Number To Decimal String(number=w2906) -> (decimal integer string=w2904:string[])  [unwired: 1 in]
              n1526 = Array Size(array=w2904) -> (size(s)=w2905:i32)
              n1527 = Replace Array Subset(array=w2907, new element=w2921, index (row)=1 ("disabled index (row)"), index (col)=w2895) -> (w2903:string[][])
              n1528 = Number To Decimal String(number=w2908) -> (decimal integer string=w2911:string)  [unwired: 1 in]
              n1529 = for {
                N: w2905 -> [_]
                tunnel: w2904 -> [w2938] mode=indexing
                shift-right: [w2934] -> w2901
                shift-left: w2903 -> [w2934]
                tunnel: [w2933] -> w2902
                i -> [w2936]
                n1530 = Equal To 0?(x=w2936) -> (x = 0?=w2937:bool)
                n1531 = case shown="True" w2937 {
                  tunnel: [w2940 w2941] -> w2935
                  frame False {
                    n1532 = local read "string"() -> (w2940:string)
                  }
                  frame True {
                    w2941 = ""
                    n1533 = local write "string"(w2941) -> ()
                  }
                }
                n1534 = call <vilib>:"Space Constant.vi"() -> ("String"=w2939:string)
                n1535 = Concatenate Strings(w2935, w2938, w2939) -> (w2933:string)
                n1536 = local write "string"(w2933) -> ()
              }
              n1537 = Replace Array Subset(array=w2901, new element=w2902, index (row)=2 ("disabled index (row)"), index (col)=w2895) -> (w2900:string[][])
              n1538 = Replace Array Subset(array=w2900, new element=w2916, index (row)=3 ("disabled index (row)"), index (col)=w2895) -> (w2913:string[][])
              n1539 = Replace Array Subset(array=w2913, new element=w2915, index (row)=4 ("disabled index (row)"), index (col)=w2895) -> (w2909:string[][])
              n1540 = Replace Array Subset(array=w2909, new element=w2911, index (row)=5 ("disabled index (row)"), index (col)=w2895) -> (w2897:string[][])
              n1541 = for {
                N: w2899 -> [_]
                tunnel: w2898 -> [w2932] mode=indexing
                shift-right: [w2929] -> w2896
                shift-left: w2897 -> [w2930]
                tunnel: w2895 -> [w2925]
                i -> [w2928]
                n1542 = Unbundle By Name(w2932) -> ("tempgoal"=w2931:i32)
                n1543 = Add(x=3 ("disabled index (row)"), y=w2925) -> (x+y=w2923:i32)
                n1544 = Add(x=7 ("disabled index (row)"), y=w2928) -> (x+y=w2926:i32)
                n1545 = Number To Decimal String(number=w2931) -> (decimal integer string=w2922:string)  [unwired: 1 in]
                n1546 = Replace Array Subset(array=w2930, new element=w2922, index (row)=w2926, index (col)=w2923) -> (w2929:string[][])
              }
            }
            frame True {
            }
          }
          n1547 = for {
            N: w2857 -> [_]
            tunnel: w2856 -> [w2878] mode=indexing
            shift-right: [w2881] -> w2869
            shift-left: w2870 -> [w2893]
            tunnel: w2867 -> [_]
            tunnel: w2858 -> [_]
            i -> [w2879]
            (unwired) 3 ("disabled index (row)")
            n1548 = Unbundle By Name(w2878) -> ("thermalsetpoint"=w2894:i32, "ramp"=w2888:i32, "soakduration"=w2884:i32)
            n1549 = Add(x=7 ("disabled index (row)"), y=w2879) -> (x+y=w2880:i32)
            n1550 = Number To Decimal String(number=w2894) -> (decimal integer string=w2891:string)  [unwired: 1 in]
            n1551 = Replace Array Subset(array=w2893, new element=w2891, index (row)=w2880, index (col)=0 ("disabled index (row)")) -> (w2890:string[][])
            n1552 = Number To Decimal String(number=w2888) -> (decimal integer string=w2887:string)  [unwired: 1 in]
            n1553 = Replace Array Subset(array=w2890, new element=w2887, index (row)=w2880, index (col)=1 ("disabled index (row)")) -> (w2882:string[][])
            n1554 = Number To Decimal String(number=w2884) -> (decimal integer string=w2885:string)  [unwired: 1 in]
            n1555 = Replace Array Subset(array=w2882, new element=w2885, index (row)=w2880, index (col)=2 ("disabled index (row)")) -> (w2881:string[][])
          }
        }
        n1556 = call-poly <vilib>:"Write Delimited Spreadsheet.vi"("2D data"=w2845, "delimiter (\\t)"="," ("delimiter (\\t)")) -> ()  [unwired: 12 in, 2 out]
      }
      frame "graphTC" {
        n1557 = property on="Waveform Chart" class="WFChart (strict)"("LegScrollVis"=TRUE ("Legend:Scrollbar Visible")) -> ()  [unwired: 2 in, 2 out]
        n1558 = Unbundle By Name(w2953) -> ("working array"=w2950:bool[], "Thermocouples"=w2951:T3, "TCs"=w2944:T10)
        n1559 = for {
          N: 120 -> [_]
          tunnel: w2944 -> [w2987] mode=indexing
          tunnel: [w2986] -> w2945 mode=indexing
          shift-right: [w2965] -> w2947
          shift-left: w2951 -> [w2972]
          shift-right: [w2964] -> w2952
          shift-left: w2950 -> [w2963]
          i -> [w2962]
          n1560 = Unbundle By Name(w2987) -> ("thermocouple"=w2996:i32, "temp"=w2960:dbl, "alarm"=w2991:i32, "working"=w2990:bool)
          n1561 = Quotient & Remainder(x=w2962, y=4) -> (x-y*floor(x/y)=w2970:i32, floor(x/y)=w2971:i32)
          n1562 = Index Array(array=w2972, index (row)=w2971, index (col)=w2970) -> (element=w2985:T14)
          n1563 = Multiply(x=w2971, y=4) -> (x*y=w2980:i32)
          n1564 = Multiply(x=w2971, y=4) -> (x*y=w2992:i32)
          n1565 = Unbundle By Name(w2985) -> ("Graph On/Off"=w2969:u32)
          n1566 = Add(x=w2980, y=w2970) -> (x+y=w2978:i32)
          n1567 = Add(x=w2992, y=w2970) -> (x+y=w2961:i32)
          n1568 = Replace Array Subset(array=w2963, new element=w2990, index=w2962) -> (w2964:bool[])
          n1569 = To Double Precision Float(number=w2960) -> (double precision float=w2959:dbl)
          n1570 = Get Date/Time In Seconds() -> (seconds since 1Jan1904=w2989:timestamp)
          n1571 = property on="Waveform Chart" class="WFChart (strict)"("Active Plot"=w2961) -> ()  [unwired: 2 in, 2 out]
          n1572 = Index Array(array=w2964, index=w2978) -> (element=w2977:bool)
          n1573 = Bundle By Name("t0"=w2989) -> (w2988:waveform(dbl))  [unwired: 1 in]
          n1574 = Build Array(w2959) -> (w2958:dbl[])
          n1575 = Number To Fractional String(number=w2959, precision (6)=i16 2 ("width (-)")) -> (F-format string=w2975:string)  [unwired: 2 in]
          n1576 = Bundle By Name(cluster=w2988, "Y"=w2958) -> (w2986:waveform(dbl))
          n1577 = case shown="True" w2977 {
            tunnel: w2969 -> [_ w3001]
            tunnel: [u32 12369084 ("y") w3001] -> w2973
            tunnel: w2975 -> [_ w3000]
            tunnel: ["NaN" w3000] -> w2974
            frame False {
            }
            frame True {
            }
          }
          n1578 = case shown="2" w2991 {
            tunnel: ["" "L" "H"] -> w2966
            tunnel: w2991 -> [_ _ _]
            tunnel: [u32 12369084 u32 2812927 u32 16711680] -> w2967
            frame 0, Default {
            }
            frame 1 {
            }
            frame 2 {
            }
          }
          n1579 = Number To Decimal String(number=w2996) -> (decimal integer string=w2997:string)  [unwired: 1 in]
          n1580 = Index Array(array=w2972, index (row)=w2971, index (col)=w2970) -> (element=w2983:T14)
          n1581 = Equal?(x=w2973, y=u32 6618880) -> (x = y?=w2981:bool)
          n1582 = Concatenate Strings("TC " ("string"), w2997) -> (w2968:string)
          n1583 = property on="Waveform Chart" class="WFChart (strict)"("Plot.Plot Name"=w2968) -> ()  [unwired: 2 in, 2 out]
          n1584 = case shown="True" w2981 {
            tunnel: [w3009 w3017] -> w2984
            tunnel: w2983 -> [w3008 w3016]
            tunnel: w2973 -> [w3006 w3015]
            tunnel: w2974 -> [w3007 w3014]
            tunnel: w2968 -> [w3005 w3013]
            tunnel: w2967 -> [w3004 w3012]
            tunnel: w2966 -> [w3003 w3011]
            frame False {
              n1585 = Bundle By Name(cluster=w3008, "Graph On/Off"=w3006, "TC Label"=w3005, "PlotColor"=u32 12369084 ("y"), "Temperature"=w3007, "Alarm Color"=w3004, "Alarm Status"=w3003) -> (w3009:T14)
            }
            frame True {
              n1586 = property on="Waveform Chart" class="WFChart (strict)"() -> ("Plot.Plot Color"=w3010:u32)  [unwired: 2 in, 2 out]
              n1587 = Bundle By Name(cluster=w3016, "Graph On/Off"=w3015, "TC Label"=w3013, "PlotColor"=w3010, "Temperature"=w3014, "Alarm Color"=w3012, "Alarm Status"=w3011) -> (w3017:T14)
            }
          }
          n1588 = Replace Array Subset(array=w2972, new element=w2984, index (row)=w2971, index (col)=w2970) -> (w2965:T3)
        }
        n1589 = local write "Thermocouples"(w2947) -> ()
        n1590 = Bundle By Name(cluster=w2953, "Thermocouples"=w2947, "working array"=w2952) -> (w2948:T13)
        n1591 = Build Array (concatenate)(waveform(dbl) {"t0"=timestamp(0 s since 1904-01-01), "dt"=1.0, "Y"=[]} ("element"), w2945) -> (w2956:waveform(dbl)[])
        n1592 = Delete From Array(array=w2956, index=0) -> (array with subset deleted=→"Waveform Chart":waveform(dbl)[])  [unwired: 1 in, 1 out]
      }
      frame "receiveCompressorTemp" {
        n1593 = Unflatten From JSON(JSON string=w3028, type and defaults=cluster{"CompressorTemp":dbl} {"CompressorTemp"=0.0}, default null elements? (F)=TRUE) -> (value=w3026:cluster{"CompressorTemp":dbl})  [unwired: 4 in, 1 out]
        n1594 = Unbundle(w3026) -> ("CompressorTemp"=w3025:dbl)
        n1595 = Bundle By Name(cluster=w3030, "Compressor.CompressorTemp"=w3025) -> (w3031:T13)
      }
      frame "receiveMCCData" {
        n1596 = Unflatten From JSON(JSON string=w3034, type and defaults=T20 {"DutyCycle"=0, "Stage1Temp"=0, "CryoPumpReadyState"={"MotorOn"=FALSE, "Ready"=FALSE}, "PurgeValveState"=FALSE, "RegenError"="", "RegenStep"="", "RoughingValveState"=FALSE, "RoughingInterlock"={"RoughingPermission"=FALSE, "RoughingNeeded"=FALSE, "Cryopumprunning"=FALSE}, "Stage2Temp"=0, "Status"={"PumpOn"=FALSE, "RoughOpen"=FALSE, "PurgeOpen"=FALSE, "ThermocoupleGaugeOn"=FALSE, "PowerFailureOccurred"=FALSE}, "TcPressure"=0}, default null elements? (F)=TRUE) -> (value=w3043:T20)  [unwired: 4 in, 1 out]
        n1597 = Unbundle By Name(w3043) -> ("Stage1Temp"=w3041:i32, "Stage2Temp"=w3040:i32)
        n1598 = To Double Precision Float(number=w3041) -> (double precision float=w3039:dbl)
        n1599 = To Double Precision Float(number=w3040) -> (double precision float=w3038:dbl)
        n1600 = Build Array(w3038) -> (w3037:dbl[])
        n1601 = Build Array(w3039) -> (w3036:dbl[])
        n1602 = Bundle(w3036, w3037) -> (w3033:cluster{dbl[], dbl[]})  [unwired: 1 in]
        n1603 = Bundle By Name(cluster=w3044, "PumpTemps"=w3033) -> (w3045:T13)
      }
      frame "receiveLastError" {
        w3059 = T32 0 items=["no dialog", "OK message", "continue or stop message", "OK message + warnings", "continue/stop + warnings"] ("type of dialog (OK msg:1)")
        n1604 = Unflatten From JSON(JSON string=w3065, type and defaults=T21 {"time"=[], "event"=[], "item"=[], "details"=[], "actions"=[]}, default null elements? (F)=TRUE) -> (value=w3052:T21, error out=w3060:errorcluster)  [unwired: 4 in]
        n1605 = Unbundle By Name(w3052) -> ("time"=w3049:string[])
        n1606 = Index Array(array=w3049, index=0) -> (element=w3048:string)
        n1607 = Not Equal?(x=w3048, y="") -> (x != y?=w3050:bool)
        n1608 = call <vilib>:"Simple Error Handler.vi"("type of dialog (OK msg:1)"=w3059, "error in (no error)"=w3060) -> ("error?"=w3053:bool)  [unwired: 3 in, 4 out]
        n1609 = Not Or(1:w3050, 2:w3053) -> (0:w3054:bool)
        n1610 = Unbundle By Name(w3058) -> ("ErrorArray"=w3056:string[][], "MasterErrorArray"=w3057:string[][])
        n1611 = case shown="False" w3054 {
          tunnel: [w3085 w3114] -> w3063
          tunnel: w3052 -> [w3084 _]
          tunnel: w3057 -> [w3083 w3114]
          tunnel: w3056 -> [w3082 w3113]
          tunnel: [w3081 w3113] -> w3055
          frame False {
            n1612 = Unbundle By Name(w3084) -> ("time"=w3073:string[], "details"=w3074:string[])
            n1613 = One Button Dialog(message="There has been an error", button name ("OK")="Proceed to Error Log") -> (true=w3069:bool)
            n1614 = case shown="True" w3069 {
              frame False {
              }
              frame True {
                n1615 = local write "Tab Control"(T22."General Status" ("Tab Control")) -> ()
              }
            }
            n1616 = Array Size(array=w3073) -> (size(s)=w3072:i32)
            n1617 = Initialize Array("", 3 ("dimension size")) -> (w3078:string[])
            n1618 = for {
              N: w3072 -> [_]
              tunnel: w3078 -> [w3102]
              tunnel: [w3100] -> w3077
              shift-right: [w3095] -> w3085
              shift-left: w3083 -> [w3087]
              tunnel: w3074 -> [w3096] mode=indexing
              tunnel: w3073 -> [w3088] mode=indexing
              shift-right: [w3093] -> w3081
              shift-left: w3082 -> [w3094]
              i -> [w3097]
              n1619 = Index Array(array=w3087, index (col)=1 ("index (row)")) -> (element=w3090:string[])  [unwired: 1 in]
              n1620 = control-ref of="Current Errors (click to clear)"() -> (w3105:refnum<vi>)
              n1621 = Replace Array Subset(array=w3102, new element=w3096, index=2) -> (w3099:string[])
              n1622 = Search 1D Array(1D array=w3090, element=w3088) -> (index of element=w3089:i32)  [unwired: 1 in]
              n1623 = Replace Array Subset(array=w3099, new element=w3088, index=1) -> (w3092:string[])
              n1624 = case shown="-1" w3089 {
                tunnel: [w3106 w3112] -> w3095
                tunnel: w3094 -> [w3107 w3111]
                tunnel: [w3107 w3110] -> w3093
                tunnel: w3092 -> [_ w3109]
                tunnel: w3087 -> [w3106 w3108]
                frame 0, Default {
                }
                frame -1 {
                  n1625 = Build Array (concatenate)(w3111, w3109) -> (w3110:string[][])
                  n1626 = Build Array (concatenate)(w3108, w3109) -> (w3112:string[][])
                }
              }
              n1627 = Bundle(w3097, 2) -> (w3103:cluster{i32, i32})  [unwired: 1 in]
              n1628 = property on="Property Node" class="MCListbox (strict)"(reference=w3105, "ActiveCell"=w3103) -> (reference out=w3100:refnum<vi>)  [unwired: 1 in, 1 out]
            }
            n1629 = Array Size(array=w3081) -> (size(s)=w3068:i32[])
            n1630 = property class="MCListbox (strict)"(reference=w3077, "ItemNames"=w3081) -> ()  [unwired: 1 in, 2 out]
            n1631 = Index Array(array=w3068, index=0) -> (element=w3066:i32)
            n1632 = Initialize Array(37, w3066) -> (w3075:i32[])
            n1633 = property class="MCListbox (strict)"(reference=w3077, "ItemSyms"=w3075) -> ()  [unwired: 1 in, 2 out]
          }
          frame True {
          }
        }
        n1634 = Bundle By Name(cluster=w3058, "MasterErrorArray"=w3063, "ErrorArray"=w3055) -> (w3064:T13)
      }
      frame "receiveLastEvent" {
        w3128 = T32 0 items=["no dialog", "OK message", "continue or stop message", "OK message + warnings", "continue/stop + warnings"] ("type of dialog (OK msg:1)")
        n1635 = Unflatten From JSON(JSON string=w3134, type and defaults=T23 {"time"=[], "category"=[], "message"=[]}, default null elements? (F)=TRUE) -> (value=w3121:T23, error out=w3129:errorcluster)  [unwired: 4 in]
        n1636 = Unbundle By Name(w3121) -> ("time"=w3118:string[])
        n1637 = Index Array(array=w3118, index=0) -> (element=w3117:string)
        n1638 = Not Equal?(x=w3117, y="") -> (x != y?=w3119:bool)
        n1639 = call <vilib>:"Simple Error Handler.vi"("type of dialog (OK msg:1)"=w3128, "error in (no error)"=w3129) -> ("error?"=w3122:bool)  [unwired: 3 in, 4 out]
        n1640 = Not Or(1:w3119, 2:w3122) -> (0:w3123:bool)
        n1641 = Unbundle By Name(w3127) -> ("EventArray"=w3125:string[][], "MasterEventArray"=w3126:string[][])
        n1642 = case shown="False" w3123 {
          tunnel: [w3151 w3179] -> w3132
          tunnel: w3121 -> [w3150 _]
          tunnel: w3126 -> [w3149 w3179]
          tunnel: w3125 -> [w3148 w3178]
          tunnel: [w3147 w3178] -> w3124
          frame False {
            n1643 = Unbundle By Name(w3150) -> ("time"=w3139:string[], "message"=w3140:string[])
            n1644 = Array Size(array=w3139) -> (size(s)=w3138:i32)
            n1645 = Initialize Array("", 3 ("dimension size")) -> (w3144:string[])
            n1646 = for {
              N: w3138 -> [_]
              tunnel: w3144 -> [w3167]
              tunnel: [w3165] -> w3143
              shift-right: [w3160] -> w3151
              shift-left: w3149 -> [w3152]
              tunnel: w3140 -> [w3161] mode=indexing
              tunnel: w3139 -> [w3153] mode=indexing
              shift-right: [w3158] -> w3147
              shift-left: w3148 -> [w3159]
              i -> [w3162]
              n1647 = Index Array(array=w3152, index (col)=1 ("index (row)")) -> (element=w3155:string[])  [unwired: 1 in]
              n1648 = control-ref of="Current Events (click to clear)"() -> (w3170:refnum<vi>)
              n1649 = Replace Array Subset(array=w3167, new element=w3161, index=2) -> (w3164:string[])
              n1650 = Search 1D Array(1D array=w3155, element=w3153) -> (index of element=w3154:i32)  [unwired: 1 in]
              n1651 = Replace Array Subset(array=w3164, new element=w3153, index=1) -> (w3157:string[])
              n1652 = case shown="0, Default" w3154 {
                tunnel: [w3171 w3177] -> w3160
                tunnel: w3159 -> [w3172 w3176]
                tunnel: [w3172 w3175] -> w3158
                tunnel: w3157 -> [_ w3174]
                tunnel: w3152 -> [w3171 w3173]
                frame 0, Default {
                }
                frame -1 {
                  n1653 = Build Array (concatenate)(w3176, w3174) -> (w3175:string[][])
                  n1654 = Build Array (concatenate)(w3173, w3174) -> (w3177:string[][])
                }
              }
              n1655 = Bundle(w3162, 2) -> (w3168:cluster{i32, i32})  [unwired: 1 in]
              n1656 = property on="Property Node" class="MCListbox (strict)"(reference=w3170, "ActiveCell"=w3168) -> (reference out=w3165:refnum<vi>)  [unwired: 1 in, 1 out]
            }
            n1657 = Array Size(array=w3147) -> (size(s)=w3137:i32[])
            n1658 = property class="MCListbox (strict)"(reference=w3143, "ItemNames"=w3147) -> ()  [unwired: 1 in, 2 out]
            n1659 = Index Array(array=w3137, index=0) -> (element=w3135:i32)
            n1660 = Initialize Array(37, w3135) -> (w3141:i32[])
            n1661 = property class="MCListbox (strict)"(reference=w3143, "ItemSyms"=w3141) -> ()  [unwired: 1 in, 2 out]
          }
          frame True {
          }
        }
        n1662 = Bundle By Name(cluster=w3127, "MasterEventArray"=w3132, "EventArray"=w3124) -> (w3133:T13)
      }
      frame "receivePressure" {
        n1663 = Unflatten From JSON(JSON string=w3181, type and defaults=T24 {"CryoPressure"=0.0, "ChamberPressure"=0.0, "RoughingPressure"=0.0}, default null elements? (F)=TRUE) -> (value=w3187:T24)  [unwired: 4 in, 1 out]
        n1664 = Unbundle By Name(w3187) -> ("CryoPressure"=w3186:dbl, "ChamberPressure"=w3185:dbl, "RoughingPressure"=w3184:dbl)
        n1665 = Build Array(w3186, w3185, w3184) -> (w3188:dbl[])
        n1666 = Bundle By Name(cluster=w3190, "Pressure"=w3188) -> (w3189:T13)
      }
      frame "receiveTC" {
        n1667 = Unflatten From JSON(JSON string=w3199, type and defaults=T25 {"time"="", "TCs"=[]} ("Cluster"), default null elements? (F)=TRUE) -> (value=w3201:T25)  [unwired: 4 in, 1 out]
        n1668 = Unbundle By Name(w3201) -> ("TCs"=w3193:T10)
        n1669 = Bundle By Name(cluster=w3200, "TCs"=w3193) -> (w3194:T13)
        n1670 = control-ref of="TC1to45visual"() -> (w3195:refnum<vi>)
        n1671 = property class="Clust (strict)"(reference=w3195) -> ("Controls[]"=w3191:refnum<vi>[])  [unwired: 1 in, 2 out]
        n1672 = for {
          N: 44 -> [_]
          tunnel: w3191 -> [w3203] mode=indexing
          tunnel: w3193 -> [w3205] mode=indexing
          n1673 = Unbundle By Name(w3205) -> ("temp"=w3204:dbl)
          n1674 = Number To Decimal String(number=w3204) -> (decimal integer string=w3202:string)  [unwired: 1 in]
          n1675 = property class="Ctl"(reference=w3203, "TipStrip"=w3202) -> ()  [unwired: 1 in, 2 out]
        }
      }
      frame "receiveZoneTemps" {
        n1676 = Unflatten From JSON(JSON string=w3209, type and defaults=cluster{"ZoneTemps":dbl[]} {"ZoneTemps"=[]}, default null elements? (F)=TRUE) -> (value=w3207:cluster{"ZoneTemps":dbl[]})  [unwired: 4 in, 1 out]
        n1677 = Bundle By Name(cluster=w3211, "ZoneTemps"=w3207) -> (w3212:T13)
      }
      frame "masterDatabase" {
        n1678 = Unbundle By Name(w3226) -> ("Thermocouples"=w3227:T3, "Pressure"=w3219:dbl[], "PumpTemps"=w3222:T11, "NumberTCs"=w3228:i32, "ZoneTemps"=w3216:cluster{"ZoneTemps":dbl[]}, "Compressor.CompressorTemp"=w3214:dbl)  [unwired: 1 out]
        n1679 = Initialize Array(0.0 ("element"), w3228) -> (w3230:dbl[])
        n1680 = Unbundle(w3222) -> ("Cp Stage 1 Temp"=w3221:dbl[], "Cp Stage 2 Temp"=w3220:dbl[])
        n1681 = Unbundle(w3216) -> ("ZoneTemps"=w3215:dbl[])
        n1682 = Build Array (concatenate)(w3221, w3220) -> (w3218:dbl[])
        n1683 = Build Array(w3214) -> (w3213:dbl[])
        n1684 = for {
          N: w3228 -> [_]
          shift-right: [w3240] -> w3217
          shift-left: w3230 -> [w3241]
          tunnel: w3227 -> [w3236]
          i -> [w3238]
          n1685 = Quotient & Remainder(x=w3238, y=4) -> (x-y*floor(x/y)=w3235:i32, floor(x/y)=w3237:i32)
          n1686 = Index Array(array=w3236, index (row)=w3237, index (col)=w3235) -> (element=w3234:T14)
          n1687 = Unbundle By Name(w3234) -> ("Temperature"=w3233:string)
          n1688 = Fract/Exp String To Number(string=w3233) -> (number=w3232:dbl)  [unwired: 3 in, 1 out]
          n1689 = To Double Precision Float(number=w3232) -> (double precision float=w3242:dbl)
          n1690 = Replace Array Subset(array=w3241, new element=w3242, index=w3238) -> (w3240:dbl[])
        }
        n1691 = Build Array (concatenate)(dbl[] [0.0], w3219, w3215, w3217, w3218, w3213) -> (w3224:dbl[])
        n1692 = Bundle By Name(cluster=w3226, "Database"=w3224) -> (w3225:T13)
      }
      frame "multipleGraphs" {
        n1693 = local read "Custom Graph Selector"() -> (w3243:i32)
        n1694 = for {
          N: 6 ("Numeric") -> [_]
          tunnel: w3246 -> [w3260]
          tunnel: w3245 -> [w3259]
          tunnel: w3243 -> [w3250]
          i -> [w3247]
          n1695 = case shown="1" w3247 {
            tunnel: [w3306 w3307 w3309 w3311 w3313 w3315] -> w3252
            tunnel: [w3305 w3308 w3310 w3312 w3314 w3316] -> w3251
            frame 0, Default {
              n1696 = control-ref of="Custom Chart 1 Selection"() -> (w3305:refnum<vi>)
              n1697 = control-ref of="Custom Chart 1"() -> (w3306:refnum<vi>)
            }
            frame 1 {
              n1698 = control-ref of="Custom Chart 2 Selection"() -> (w3308:refnum<vi>)
              n1699 = control-ref of="Custom Chart 2"() -> (w3307:refnum<vi>)
            }
            frame 2 {
              n1700 = control-ref of="Custom Chart 3 Selection"() -> (w3310:refnum<vi>)
              n1701 = control-ref of="Custom Chart 3"() -> (w3309:refnum<vi>)
            }
            frame 3 {
              n1702 = control-ref of="Custom Chart 4 Selection"() -> (w3312:refnum<vi>)
              n1703 = control-ref of="Custom Chart 4"() -> (w3311:refnum<vi>)
            }
            frame 4 {
              n1704 = control-ref of="Custom Chart 5 Selection"() -> (w3314:refnum<vi>)
              n1705 = control-ref of="Custom Chart 5"() -> (w3313:refnum<vi>)
            }
            frame 5 {
              n1706 = control-ref of="Custom Chart 6 Selection"() -> (w3316:refnum<vi>)
              n1707 = control-ref of="Custom Chart 6"() -> (w3315:refnum<vi>)
            }
          }
          n1708 = Equal?(x=w3250, y=w3247) -> (x = y?=w3248:bool)
          n1709 = Unbundle By Name(w3259) -> ("Database"=w3257:dbl[], "numSensors"=w3258:i32)
          n1710 = case shown="True" w3248 {
            tunnel: w3260 -> [_ w3274]
            tunnel: [w3263 w3268] -> w3256
            tunnel: [1000 w3267] -> w3255
            tunnel: w3251 -> [w3264 w3266]
            tunnel: [FALSE w3265] -> w3249
            frame False {
              n1711 = property on="Property Node" class="LstBox (strict)"(reference=w3264) -> ("Item Symbols"=w3263:i32[])  [unwired: 1 in, 2 out]
            }
            frame True {
              n1712 = property on="Property Node" class="LstBox (strict)"(reference=w3266) -> ("Item Symbols"=w3268:i32[])  [unwired: 1 in, 2 out]
              n1713 = Decimal String To Number(string=w3274) -> (number=w3267:i32)  [unwired: 2 in, 1 out]
              n1714 = Index Array(array=w3268, index=0) -> (element=w3269:i32)
              n1715 = Equal?(x=37, y=w3269) -> (x = y?=w3271:bool)
              n1716 = Equal To 0?(x=w3267) -> (x = 0?=w3273:bool)
              n1717 = And(x=w3271, y=w3273) -> (x .and. y?=w3265:bool)
            }
          }
          n1718 = case shown="True" w3249 {
            tunnel: [0 ("index") w3379] -> w3254
            tunnel: w3258 -> [w3323 w3375]
            tunnel: w3257 -> [w3322 _]
            tunnel: [w3321 _] -> w3253
            tunnel: w3255 -> [w3319 w3379]
            tunnel: w3256 -> [w3320 w3378]
            tunnel: w3251 -> [w3318 w3374]
            tunnel: w3252 -> [w3317 w3373]
            frame False {
              n1719 = for {
                N: w3323 -> [_]
                tunnel: [w3348] -> w3321 mode=indexing
                tunnel: w3319 -> [w3342]
                tunnel: w3320 -> [w3337]
                tunnel: w3322 -> [w3326] mode=indexing
                tunnel: w3318 -> [w3335]
                tunnel: w3317 -> [w3334]
                i -> [w3333]
                n1720 = Wait (ms)(milliseconds to wait=u32 0) -> ()  [unwired: 1 out]
                n1721 = In Range and Coerce(upper limit=22, x=w3333, lower limit=3) -> (In Range?=w3330:bool)  [unwired: 1 out]
                n1722 = Equal To 0?(x=w3326) -> (x = 0?=w3327:bool)
                n1723 = Not A Number/Path/Refnum?(number/path/refnum=w3326) -> (NaN/Path/Refnum?=w3325:bool)
                n1724 = Or(x=w3325, y=w3327) -> (x .or. y?=w3328:bool)
                n1725 = Not And(1:w3330, 2:w3328) -> (0:w3329:bool)
                n1726 = case shown="True" w3329 {
                  tunnel: [waveform(dbl) {"t0"=timestamp(0 s since 1904-01-01), "dt"=1.0, "Y"=[]} w3352] -> w3348
                  tunnel: w3326 -> [_ w3350]
                  frame False {
                  }
                  frame True {
                    n1727 = Get Date/Time In Seconds() -> (seconds since 1Jan1904=w3354:timestamp)
                    n1728 = Bundle By Name("t0"=w3354) -> (w3353:waveform(dbl))  [unwired: 1 in]
                    n1729 = Build Array(w3350) -> (w3351:dbl[])
                    n1730 = Bundle By Name(cluster=w3353, "Y"=w3351) -> (w3352:waveform(dbl))
                  }
                }
                n1731 = Index Array(array=w3337, index=w3342) -> (element=w3340:i32)
                n1732 = Index Array(array=w3337, index=w3342) -> (element=w3343:i32)
                n1733 = Equal?(x=w3340, y=38) -> (x = y?=w3339:bool)
                n1734 = Equal?(x=w3343, y=37) -> (x = y?=w3345:bool)
                n1735 = Equal?(x=w3333, y=w3342) -> (x = y?=w3338:bool)
                n1736 = And(x=w3338, y=w3339) -> (x .and. y?=w3336:bool)
                n1737 = And(x=w3338, y=w3345) -> (x .and. y?=w3344:bool)
                n1738 = case shown="True" w3344 {
                  tunnel: w3337 -> [_ w3372]
                  tunnel: w3342 -> [_ _]
                  tunnel: w3333 -> [_ w3367]
                  tunnel: w3334 -> [_ w3366]
                  tunnel: w3335 -> [_ w3365]
                  frame False {
                  }
                  frame True {
                    n1739 = property on="Property Node" class="WFChart (strict)"(reference=w3366, "Active Plot"=w3367) -> (reference out=w3370:refnum<vi>)  [unwired: 1 in, 1 out]
                    n1740 = Replace Array Subset(array=w3372, new element=38, index=w3367) -> (w3368:i32[])
                    n1741 = property on="Property Node" class="WFChart (strict)"(reference=w3366) -> ("Plot.Plot Color"=w3364:u32)  [unwired: 1 in, 2 out]
                    n1742 = property on="Property Node" class="WFChart (strict)"(reference=w3370, "Plot.Visible?"=TRUE ("Plot.Visible")) -> ()  [unwired: 1 in, 2 out]
                    n1743 = property on="Property Node" class="LstBox (strict)"(reference=w3365, "Active Row"=w3367) -> ()  [unwired: 1 in, 2 out]
                    n1744 = property on="Property Node" class="LstBox (strict)"(reference=w3365, "CellBG"=w3364) -> ()  [unwired: 1 in, 2 out]
                    n1745 = property on="Property Node" class="LstBox (strict)"(reference=w3365, "Item Symbols"=w3368) -> ()  [unwired: 1 in, 2 out]
                  }
                }
                n1746 = case shown="True" w3336 {
                  tunnel: w3337 -> [_ w3363]
                  tunnel: w3333 -> [_ w3356]
                  tunnel: w3334 -> [_ w3357]
                  tunnel: w3335 -> [_ w3358]
                  frame False {
                  }
                  frame True {
                    n1747 = property on="Property Node" class="WFChart (strict)"(reference=w3357, "Active Plot"=w3356) -> (reference out=w3361:refnum<vi>)  [unwired: 1 in, 1 out]
                    n1748 = Replace Array Subset(array=w3363, new element=37, index=w3356) -> (w3359:i32[])
                    n1749 = property on="Property Node" class="WFChart (strict)"(reference=w3361, "Plot.Visible?"=FALSE ("Plot.Visible")) -> ()  [unwired: 1 in, 2 out]
                    n1750 = property on="Property Node" class="LstBox (strict)"(reference=w3358, "Active Row"=w3356) -> ()  [unwired: 1 in, 2 out]
                    n1751 = property on="Property Node" class="LstBox (strict)"(reference=w3358, "CellBG"=u32 13816530 ("Active Row:Cell Background Color")) -> ()  [unwired: 1 in, 2 out]
                    n1752 = property on="Property Node" class="LstBox (strict)"(reference=w3358, "Item Symbols"=w3359) -> ()  [unwired: 1 in, 2 out]
                  }
                }
              }
            }
            frame True {
              n1753 = for {
                N: w3375 -> [_]
                tunnel: w3378 -> [_]
                tunnel: w3374 -> [w3381]
                tunnel: w3373 -> [w3380]
                i -> [w3382]
                n1754 = property on="Property Node" class="WFChart (strict)"(reference=w3380, "Active Plot"=w3382) -> (reference out=w3385:refnum<vi>)  [unwired: 1 in, 1 out]
                n1755 = property on="Property Node" class="WFChart (strict)"(reference=w3385, "Plot.Visible?"=FALSE ("Plot.Visible")) -> ()  [unwired: 1 in, 2 out]
                n1756 = property on="Property Node" class="LstBox (strict)"(reference=w3381, "Active Row"=w3382) -> ()  [unwired: 1 in, 2 out]
                n1757 = property on="Property Node" class="LstBox (strict)"(reference=w3381, "CellBG"=u32 13816530 ("Active Row:Cell Background Color")) -> ()  [unwired: 1 in, 2 out]
              }
              n1758 = Initialize Array(37, w3375) -> (w3376:i32[])
              n1759 = property on="Property Node" class="LstBox (strict)"(reference=w3374, "Item Symbols"=w3376) -> ()  [unwired: 1 in, 2 out]
            }
          }
          n1760 = case shown="0, Default" w3247 {
            tunnel: w3254 -> [w3276 w3281 w3286 w3291 w3296 w3301]
            tunnel: w3253 -> [w3275 w3280 w3285 w3290 w3295 w3300]
            frame 0, Default {
              n1761 = Build Array (concatenate)(waveform(dbl) {"t0"=timestamp(0 s since 1904-01-01), "dt"=1.0, "Y"=[]} ("element"), w3275) -> (w3279:waveform(dbl)[])
              n1762 = Delete From Array(array=w3279, index=w3276) -> (array with subset deleted=→"Custom Chart 1":waveform(dbl)[])  [unwired: 1 in, 1 out]
            }
            frame 1 {
              n1763 = Build Array (concatenate)(waveform(dbl) {"t0"=timestamp(0 s since 1904-01-01), "dt"=1.0, "Y"=[]} ("element"), w3280) -> (w3284:waveform(dbl)[])
              n1764 = Delete From Array(array=w3284, index=w3281) -> (array with subset deleted=→"Custom Chart 2":waveform(dbl)[])  [unwired: 1 in, 1 out]
            }
            frame 2 {
              n1765 = Build Array (concatenate)(waveform(dbl) {"t0"=timestamp(0 s since 1904-01-01), "dt"=1.0, "Y"=[]} ("element"), w3285) -> (w3289:waveform(dbl)[])
              n1766 = Delete From Array(array=w3289, index=w3286) -> (array with subset deleted=→"Custom Chart 3":waveform(dbl)[])  [unwired: 1 in, 1 out]
            }
            frame 3 {
              n1767 = Build Array (concatenate)(waveform(dbl) {"t0"=timestamp(0 s since 1904-01-01), "dt"=1.0, "Y"=[]} ("element"), w3290) -> (w3294:waveform(dbl)[])
              n1768 = Delete From Array(array=w3294, index=w3291) -> (array with subset deleted=→"Custom Chart 4":waveform(dbl)[])  [unwired: 1 in, 1 out]
            }
            frame 4 {
              n1769 = Build Array (concatenate)(waveform(dbl) {"t0"=timestamp(0 s since 1904-01-01), "dt"=1.0, "Y"=[]} ("element"), w3295) -> (w3299:waveform(dbl)[])
              n1770 = Delete From Array(array=w3299, index=w3296) -> (array with subset deleted=→"Custom Chart 5":waveform(dbl)[])  [unwired: 1 in, 1 out]
            }
            frame 5 {
              n1771 = Build Array (concatenate)(waveform(dbl) {"t0"=timestamp(0 s since 1904-01-01), "dt"=1.0, "Y"=[]} ("element"), w3300) -> (w3304:waveform(dbl)[])
              n1772 = Delete From Array(array=w3304, index=w3301) -> (array with subset deleted=→"Custom Chart 6":waveform(dbl)[])  [unwired: 1 in, 1 out]
            }
          }
        }
      }
      frame "exit" {
        n1773 = Unbundle By Name(w3387) -> ("Http session"=w3388:T12)
        n1774 = call <vilib>:"CloseHandle.vi"("client handle"=w3388, "error in (no error)"=w3390) -> ("error out"=w3389:errorcluster)  [unwired: 13 in]
        n1775 = Bundle By Name(cluster=w3387, "go"=FALSE ("Bundle Element")) -> (w3391:T13)
      }
      frame Default {
        n1776 = call "Unknown Message Dialog.vi"("error in (no error)"=w3394, "event name"=w3393) -> ("error out"=w3392:errorcluster)  [unwired: 9 in]
      }
    }
    n1777 = Unbundle By Name(w70) -> ("go"=w69:bool)
    n1778 = call "log system event.vi"("error in (no error)"=w72) -> ("error out"=w71:errorcluster, "description"=→"system log event":string)  [unwired: 9 in]
  }
  n1779 = local read "Local Debug"() -> (w37:bool)
  n1780 = call "getData.vi"("Local Debug"=w37) -> ()  [unwired: 11 in]
  n1781 = call <vilib>:"Read PNG File.vi"("path to PNG file"=path "C:/Users/stefan/Documents/GitHub/TVAC/head/Labview2017/TVAC_GUI/Visualization/chamber_test.png") -> ("image data"=w13:T33)  [unwired: 8 in, 2 out]
  n1782 = call <vilib>:"Draw Flattened Pixmap.vi"("image data"=w13) -> ("new picture"=w12:picture)  [unwired: 8 in]
  n1783 = local read "TC1to45visual"() -> (w11:T7)
  n1784 = Bundle By Name(cluster=w11, "new picture"=w12) -> (w10:T7)
  n1785 = local write "TC1to45visual"(w10) -> ()
  n1786 = control-ref of="TC1to45visual"() -> (w6:refnum<vi>)
  n1787 = property class="Clust (strict)"(reference=w6) -> ("Controls[]"=w5:refnum<vi>[])  [unwired: 1 in, 2 out]
  n1788 = Initialize Array(T1 {"Left"=0, "Top"=0} ("Position"), 45 ("dimension size")) -> (w2:T1[])
  n1789 = for {
    N: 45 -> [_]
    tunnel: w5 -> [w3400] mode=indexing
    shift-right: [w3398] -> _
    shift-left: w2 -> [w3399]
    i -> [w3396]
    # "Delete at End"
    n1790 = property class="Ctl"(reference=w3400) -> ("Position"=w3397:T1)  [unwired: 1 in, 2 out]
    n1791 = Replace Array Subset(array=w3399, new element=w3397, index=w3396) -> (w3398:T1[])
  }
  n1792 = call "Flush Module Queue.vi"("error in (no error)"=w21) -> ("error out"=w20:errorcluster, "flushed msgs"=→"flushed msgs":T8)  [unwired: 9 in]
  n1793 = call "Unload Module.vi"("error in (no error)"=w20) -> ()  [unwired: 10 in, 1 out]
  n1794 = property on="Waveform Chart" class="WFChart (strict)" props=["Plot", "Visible?"]() -> ()  [unwired: 2 in, 3 out]
